vi "TLB Native Dynamic Events ver 0.26g.vi"() -> ()   [LabVIEW 2018]
uses:
  TLB Type Definitions/Intruction Type Definitions.ctl
  TLB Type Definitions/State Type Definitions, for 0.26g versions and later 3.ctl
  <vilib>/Studica/Studica Toolkit/NavX/TypeDefs/Flags/Z900_navX_Flags_OpStatusTypeDef.ctl
  <vilib>/Studica/Studica Toolkit/NavX/TypeDefs/Flags/Z900_navX_Flags_CalibrationStatusTypeDef.ctl
  TLB Type Definitions/Vision cluster.ctl
  TLB Type Definitions/PING CLUSTER.ctl
  TLB Type Definitions/Encoder cluster.ctl
  TLB Type Definitions/Stepper cluster.ctl
  TLB Type Definitions/Yaw Cluster.ctl
  TLB Type Definitions/IR Sensor Type Def.ctl
  TLB Type Definitions/Line Sensor Cluster.ctl
  TLB Type Definitions/Time cluster.ctl
  TLB Type Definitions/Box Colour Detection Cluster (0.26d and above).ctl
  Underlying VI's/FGV's/Box FGV/Box Colour FGV Colours.ctl
  <vilib>/Studica/Studica Toolkit/Background/DIO Channel.ctl
  TLB Type Definitions/Y Stepper cluster.ctl
  TLB Type Definitions/Motor Speed Cluster.ctl
  Labview Training Phase 2/Enum Controls/States for Action Engine.ctl
  Underlying VI's/NavX VI/navX type def.ctl
  <vilib>/Studica/Studica Toolkit/Background/I2C Channel.ctl
  Underlying VI's/I2C Master VI/Arduino_Interfacing.ctl
  Underlying VI's/Motor Control VI with PID/MOTOR CONTROL WITH PID AE DATA MODE TYPE DEF.ctl
  Underlying VI's/Motor Control VI with PID/MOTOR CONTROL WITH PID AE DIRECTION TYPE DEF.ctl
  Experimental VI's/Archived VI's/MOTOR CONTROL NO PID Type Def.ctl
  <vilib>/myRIO/Common/Instrument Driver Framework/myRIO v1.0/AI/typedefs/AI Channels List.ctl
  <vilib>/myRIO/Common/Instrument Driver Framework/myRIO v1.0/AI/typedefs/AI Channels Enum.ctl
  Underlying VI's/Line Sensor AE/Line Sensor AE Type Def.ctl
  Underlying VI's/I2C Master VI/I2C MASTER Type Def.ctl
  Underlying VI's/Elasped Timer/Elapsed timer control.ctl
  Underlying VI's/IMAQ Create Reference AE/IMAQ Reference AE.ctl
  Underlying VI's/FGV's/Box FGV/Box Colour FGV States.ctl
  Underlying VI's/I2C Master VI/I2C_MASTER_WRITE_NEW Type Def.ctl
  Underlying VI's/Modified webcam FGV/Webcam AE.ctl
  <vilib>/userdefined/High Color/IMAQdx.ctl
  <vilib>/Studica/Studica Toolkit/NavX/NavX.lvlib
  <vilib>/NI_Real-Time Target Support.lvlib
panel:
  out "Distance to move":dbl
  out "Same colour?":bool
  out "Box Colour Detection":T1
  out "Errors detected":bool
  out "Robot ready":bool
  out "Time cluster":T3
  out "Table IR obstruct":bool
  out "Front IR obstruct":bool
  out "CPU 1 Usage":dbl
  out "CPU 0 Usage":dbl
  out "Line sensors":T4
  out "IR Sensors":T5
  out "NAVX Values":T6
  out "Stepper position values":T7
  out "Encoder values":T8
  out "Ultrasonic sensors":T9
  out "Selected Task":T10=enum."Start Task 9"
  out "Object recognition mode":enum16{"Ball", "Soap", "Gel", "Pipe", "None"}(ring)
  out "Image Processing Error":errorcluster
  out "Object Detection":T11
  out "Status":T14 {"OP Status" items=["INITIALIZING", "SELFTEST_IN_PROGRESS", "ERROR", "IMU_AUTOCAL_IN_PROGRESS", "NORMAL"]; "Calibration Status" items=["IMU_CAL_STATE_MASK"=3, "IMU_CAL_STATE_INPROGRESS"=0, "IMU_CAL_STATE_ACCUMULATE"=1, "IMU_CAL_STATE_COMPLETE"=2]}
  out "General Errors":errorcluster
  in  "Red LED":bool
  out "Front Ultrasonic obstruct":bool
  out "Speed & distance":T15
  out "Task selection":u8
  out "NavX Readings":T16
  out "Arduino Data":T17
  out "TASK ENABLE":bool
  out "Rising Edge":bool
  in  "Green LED":bool
  out "State Logic":T18=enum."Startup"
  out "elements":T10[](array[typedef])
  in  "STOP TASK":bool
  in  "OK Button":bool
  in  "STOP":bool
  out "Queue Errors":errorcluster
  out "Action Queue Items":i32
  out "State Logic Queue Items":i32
  out "Action Queues items":string[](array[string])=["Hardware reset", "Software reset", ""]
  out "Action State":string
  # "VISION"
  # "TLB FRAMEWORK STATUS"
  # "System Health Status Update"
  # "Test Programme written by Calvin Loke    Dated: 28 Aug 2019\nTest Programme revised by Dr Alex See   Dated 30 Aug 2019\n\nRevision date: 20/03/2020\nProgramme version:   TLB Native Dynamic Events ver 0.19a"
  # "0: Task 1\n1: Task 2\n2: Task 3\n3: Task 4\n4: Task 5\n5: Task 6\n6: Task 7\n7: Task 8 Ball\n8: Task 8 Soap\n9: Task 8 Gel\n10: Task 8 Pipe\n11: Task 9 Blue\n12: Task 9 Black\n13: Task 9 Green\n14: Task 9 Red\n15: Task 9 Yellow"
  # "Ball: Right\nSoap: Left\nGel: Reverse\nPipe: Forward"
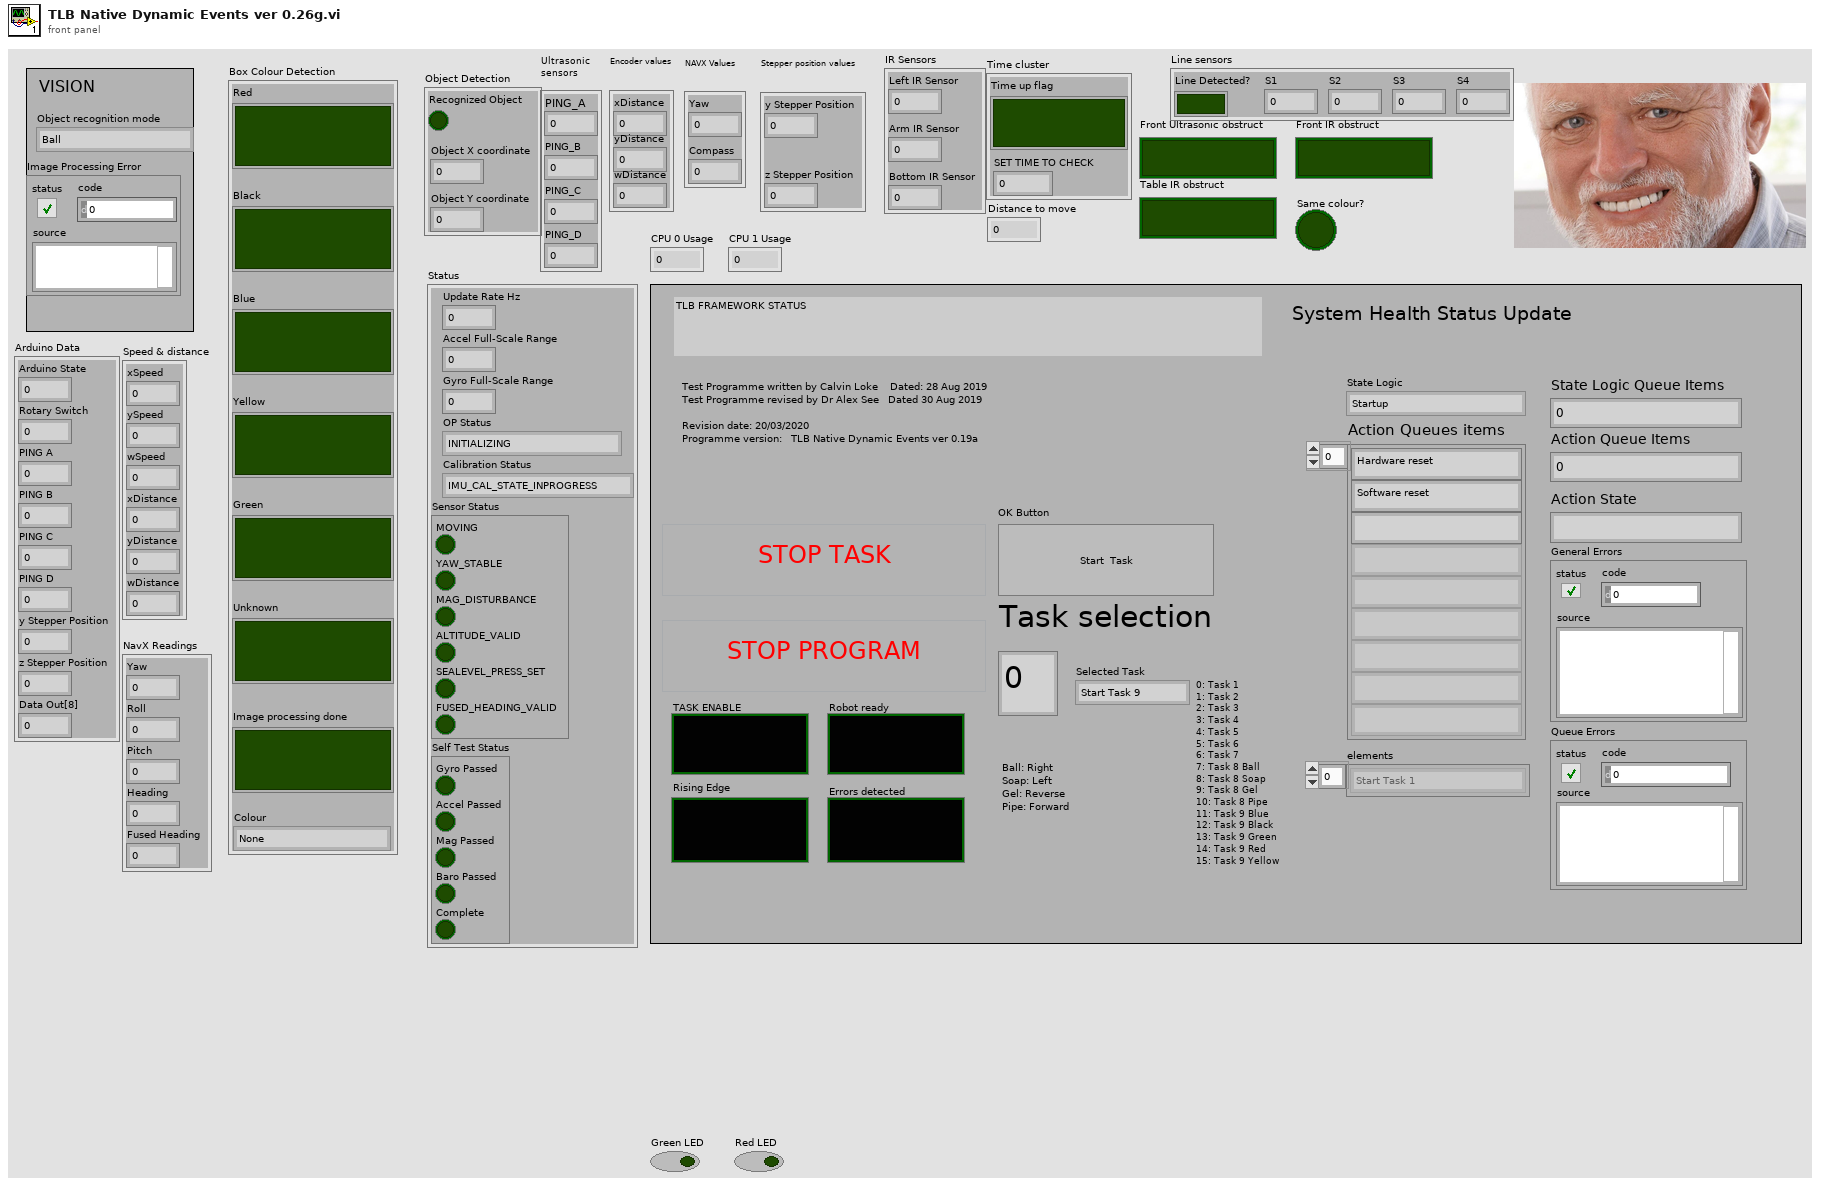
[diagram p1: front panel]
types:
  T1 = typedef "Box Colour Detection Cluster (0.26d and above).ctl" = cluster{"Red":bool, "Black":bool, "Blue":bool, "Yellow":bool, "Green":bool, "Unknown":bool, "Image processing done":bool, "Colour":T2}
  T2 = typedef "Box Colour FGV Colours.ctl" = enum16{"None", "Black", "Blue", "Green", "Red", "Yellow"}
  T3 = typedef "Time cluster.ctl" = cluster{"Time up flag":bool, "SET TIME TO CHECK":dbl}
  T4 = typedef "Line Sensor Cluster.ctl" = cluster{"Line Detected?":bool, "S1":dbl, "S2":dbl, "S3":dbl, "S4":dbl}
  T5 = typedef "IR Sensor Type Def.ctl" = cluster{"Left IR Sensor":dbl, "Arm IR Sensor":dbl, "Bottom IR Sensor":dbl}
  T6 = typedef "Yaw Cluster.ctl" = cluster{"Yaw":dbl, "Compass":dbl}
  T7 = typedef "Stepper cluster.ctl" = cluster{"y Stepper Position":u8, "z Stepper Position":u8}
  T8 = typedef "Encoder cluster.ctl" = cluster{"xDistance":dbl, "yDistance":dbl, "wDistance":dbl}
  T9 = typedef "PING CLUSTER.ctl" = cluster{"PING_A":u8, "PING_B":u8, "PING_C":u8, "PING_D":u8}
  T10 = typedef "Intruction Type Definitions.ctl" = enum16{"None", "Start Task 1", "Start Task 2", "Start Task 3", "Start Task 4", "Start Task 5", "Start Task 6", "Start Task 7", "Start Task 8 - BALL", "Start Task 8 - Gel", "Start Task 8 - Pipe", "Start Task 8 - Soap", "Start Task 9", "Start Task A", "Start Task B", "Exit"}
  T11 = typedef "Vision cluster.ctl" = cluster{"Recognized Object":bool, "Object X coordinate":dbl, "Object Y coordinate":dbl}
  T12 = typedef "NavX.lvlib/Z900_navX_Flags_OpStatusTypeDef.ctl" = u8
  T13 = typedef "NavX.lvlib/Z900_navX_Flags_CalibrationStatusTypeDef.ctl" = u8
  T14 = cluster{"Update Rate Hz":u8, "Accel Full-Scale Range":u8, "Gyro Full-Scale Range":u16, "OP Status":T12, "Calibration Status":T13, "Sensor Status":cluster{"MOVING":bool, "YAW_STABLE":bool, "MAG_DISTURBANCE":bool, "ALTITUDE_VALID":bool, "SEALEVEL_PRESS_SET":bool, "FUSED_HEADING_VALID":bool}, "Self Test Status":cluster{"Gyro Passed":bool, "Accel Passed":bool, "Mag Passed":bool, "Baro Passed":bool, "Complete":bool}}
  T15 = cluster{"xSpeed":dbl, "ySpeed":dbl, "wSpeed":dbl, "xDistance":dbl, "yDistance":dbl, "wDistance":dbl}
  T16 = cluster{"Yaw":dbl, "Roll":dbl, "Pitch":dbl, "Heading":dbl, "Fused Heading":dbl}
  T17 = cluster{"Arduino State":u8, "Rotary Switch":u8, "PING A":u8, "PING B":u8, "PING C":u8, "PING D":u8, "y Stepper Position":u8, "z Stepper Position":u8, "Data Out[8]":u8}
  T18 = typedef "State Type Definitions, for 0.26g versions and later 3.ctl" = enum16{"None", "Startup", "Move to Angle", "True Stop", "Idle", "Shutdown", "Task 1A", "Task 1B", "Task 2:Raise Arm", "Task 2:Sensor Mode", "Task 2:Reverse Mode", "Task 3", "Task 4_A", "Task 4_B", "Task 4_C", "Task 4_D", "Task 5A: RAISING ARM", "Task 5B: STILL WAITING", "Task 5C: GOING DOWN", "Task 5D: GRAB", "Task 5E: GOING UP", "Task 5F: ARM GRAB HEIGHT", "Task 5G: CLOSE CLAW", "Task 5H: RAISE ARM", "Task 6A: RAISE ARM", "Task 6B: CAM BURST", "Task 6C: PROCESS IMAGE", "Task 6D: BALL BUSTER", "Task 6E: STILL WAITING", "Task 6F: CAM BURST 2", "Task 6G: PROCESS IMAGE 2", "Task 6H: SKADI SOAPS", "Task 6I: STILL WAITING 2", "Task 6J: CAM BURST 3", "Task 6K: PROCESS IMAGE 3", "Task 6L: JAM IT IN", "Task 6M: STILL WAITING 3", "Task 6N: CAM BURST 4", "Task 6O: PROCESS IMAGE 4", "Task 6P: PIPE BOMB", "Task 7", "Task 8A: RAISE ARM", "Task 8B: MOVE TO BOX", "Task 8C: CAM BURST", "Task 8D: PROCESS IMAGE", "Task 8E: ROBOT ADJUST", "Task 8F: CAM BURST 2", "Task 8G: PROCESS IMAGE 2", "Task 8H: ARM ADJUST", "Task 8I: ARM GRAB HEIGHT", "Task 8J: CLOSE CLAW", "Task 8K: RAISE MY SWORD", "Task 9A: Raise Arm", "Task 9B: Rotate to Angle", "Task 9C: Detect Box", "Task 9D: MOVE FORWARD", "Task 9E: MOVE LEFT", "Task 9F: SCAN BOX", "Task 9G: MOVE RIGHT", "Task 9H: SCAN BOX 2", "Task 9I: ROTATE 90 CW", "Task 9J: FORWARD", "Task 9K: RAM WALL", "Task 9L: MOVE RIGHT", "Task 9M: SCAN BOX 3", "Task 9N: MOVE RIGHT", "Task 9O: SCAN BOX 4"}
  T19 = typedef "Motor Speed Cluster.ctl" = cluster{"ySpeed":dbl, "xSpeed":dbl, "wSpeed":dbl}
  T20 = typedef "Y Stepper cluster.ctl" = cluster{"yStepper desired":u8}
  T21 = typedef "DIO Channel.ctl" = enum16{"Not Connected", "A/DIO1", "A/DIO2", "A/DIO3", "A/DIO4", "A/DIO5", "A/DIO6", "A/DIO7", "A/DIO13", "B/DIO1", "B/DIO2", "B/DIO3", "B/DIO4", "B/DIO5", "B/DIO6", "B/DIO7", "B/DIO13", "C/DIO0", "C/DIO1", "C/DIO2", "C/DIO3", "C/DIO4", "C/DIO5", "C/DIO6", "C/DIO7"}
  T22 = cluster{"DIO Channel":T21, "FPGA VI Reference Out":refnum<k20>}
  T23 = typedef "States for Action Engine.ctl" = enum16{"Initialize", "Write", "Read"}
  T24 = typedef "NI_Real-Time Target Support.lvlib/RT CPU Load.ctl" = cluster{"Total (%)":dbl, "Time Critical (%)":dbl, "Timed Structures (%)":dbl, "High (%)":dbl, "Above Normal (%)":dbl, "Normal (%)":dbl, "Background (%)":dbl, "Idle (%)":dbl, "ISR (%)":dbl}
  T25 = cluster{"CPU loads[0]":T24, "CPU loads[1]":T24, "CPU loads[2]":T24, "CPU loads[3]":T24, "CPU loads[4]":T24, "CPU loads[5]":T24, "CPU loads[6]":T24, "CPU loads[7]":T24, "CPU loads[8]":T24}
  T26 = typedef "navX type def.ctl" = enum16{"Get i2C reference", "Read Values", "Zero Yaw"}
  T27 = typedef "Arduino_Interfacing.ctl" = enum16{"Initialize", "Write to Arduino", "Read From Arduino"}
  T28 = typedef "I2C Channel.ctl" = enum16{"Not Connected", "A", "B"}
  T29 = cluster{"I2C Ref Out":cluster{"I2C Channel":T28, "FPGA VI Reference Out":refnum<k20>}, "Connected":bool, "Slave Address (7-bit)":u8, "Registry":u8[]}
  T30 = typedef "Box Colour FGV States.ctl" = enum16{"Initialize", "Read", "Write"}
  T31 = typedef "MOTOR CONTROL WITH PID AE DIRECTION TYPE DEF.ctl" = enum16{"y-axis movement", "x-axis movement", "rotation", "stop", "reset encoders"}
  T32 = typedef "MOTOR CONTROL WITH PID AE DATA MODE TYPE DEF.ctl" = enum16{"Init AE", "Write to AE", "Read from AE"}
  T33 = typedef "Line Sensor AE Type Def.ctl" = enum16{"INIT AE", "READ FROM LINE SENSORS"}
  T34 = typedef "IMAQ Reference AE.ctl" = enum16{"Initialize AE", "Get IMAQ Reference", "Dispose Processing Buffer"}
  T35 = typedef "Elapsed timer control.ctl" = enum16{"Start", "Pause", "Initialize"}
  T36 = typedef "I2C_MASTER_WRITE_NEW Type Def.ctl" = enum16{"Ultrasonic sensors", "Stepper origin", "zStepper 13.3k", "zStepper 13k", "zStepper 12k", "zStepper 11k", "zStepper 10k", "zStepper 9k", "zStepper 8k", "zStepper 7k", "zStepper 6k", "zStepper 5k", "zStepper 4k", "zStepper 3k", "zStepper 2k", "zStepper 1k", "zStepper 900", "zStepper 800", "zStepper 700", "zStepper 600", "zStepper 500", "zStepper 400", "zStepper 300", "zStepper 200", "zStepper 100", "zStepper 0", "yStepper control", "Open Claw", "Close Claw", "Soft Reset"}
  T37 = typedef "Webcam AE.ctl" = enum16{"Initialize Camera", "Open Camera", "Continuous Acquisition", "Close Camera", "Retrieve Image", "Dispose Camera Image Buffer"}
  T38 = typedef "IMAQdx.ctl" = refnum<k21>
  T39 = typedef "MOTOR CONTROL NO PID Type Def.ctl" = enum16{"Init", "Front Back", "Left Right", "Rotate", "Stop", "Latch"}
  T40 = typedef "AI Channels List.ctl" = T41[]
  T41 = typedef "AI Channels Enum.ctl" = enum16{"Not Connected", "AudioIn/Left", "AudioIn/Right", "C/AI0", "C/AI1", "A/AI0", "A/AI1", "A/AI2", "A/AI3", "A/AI4", "A/AI5", "A/AI6", "A/AI7", "B/AI0", "B/AI1", "B/AI2", "B/AI3", "B/AI4", "B/AI5", "B/AI6", "B/AI7", "AI/AI0", "AI/AI1", "AI/AI2", "AI/AI3", "A/AI0 (DIFF)", "A/AI1 (DIFF)", "A/AI2 (DIFF)", "A/AI3 (DIFF)", "B/AI0 (DIFF)", "B/AI1 (DIFF)", "B/AI2 (DIFF)", "B/AI3 (DIFF)"}
  T42 = cluster{"S1":dbl, "S2":dbl, "S3":dbl, "S4":dbl, "Array[4]":dbl, "Array[5]":dbl, "Array[6]":dbl, "Array[7]":dbl, "Array[8]":dbl}
  T43 = typedef "I2C MASTER Type Def.ctl" = enum16{"Last State", "Mode 0", "Mode 1", "Mode 2", "Mode 3", "Mode 4", "Mode 5", "Mode 6", "Mode 7", "Mode 8", "Mode 9", "Mode 10"}
  T44 = typedef "IMAQ Image.ctl" = refnum<image>
  T45 = cluster{"Number of Matches":i32, "Object detected?":bool}
  T46 = cluster{"Red":bool, "Black":bool, "Blue":bool, "Yellow":bool, "Green":bool, "No recognizable coolour":bool}
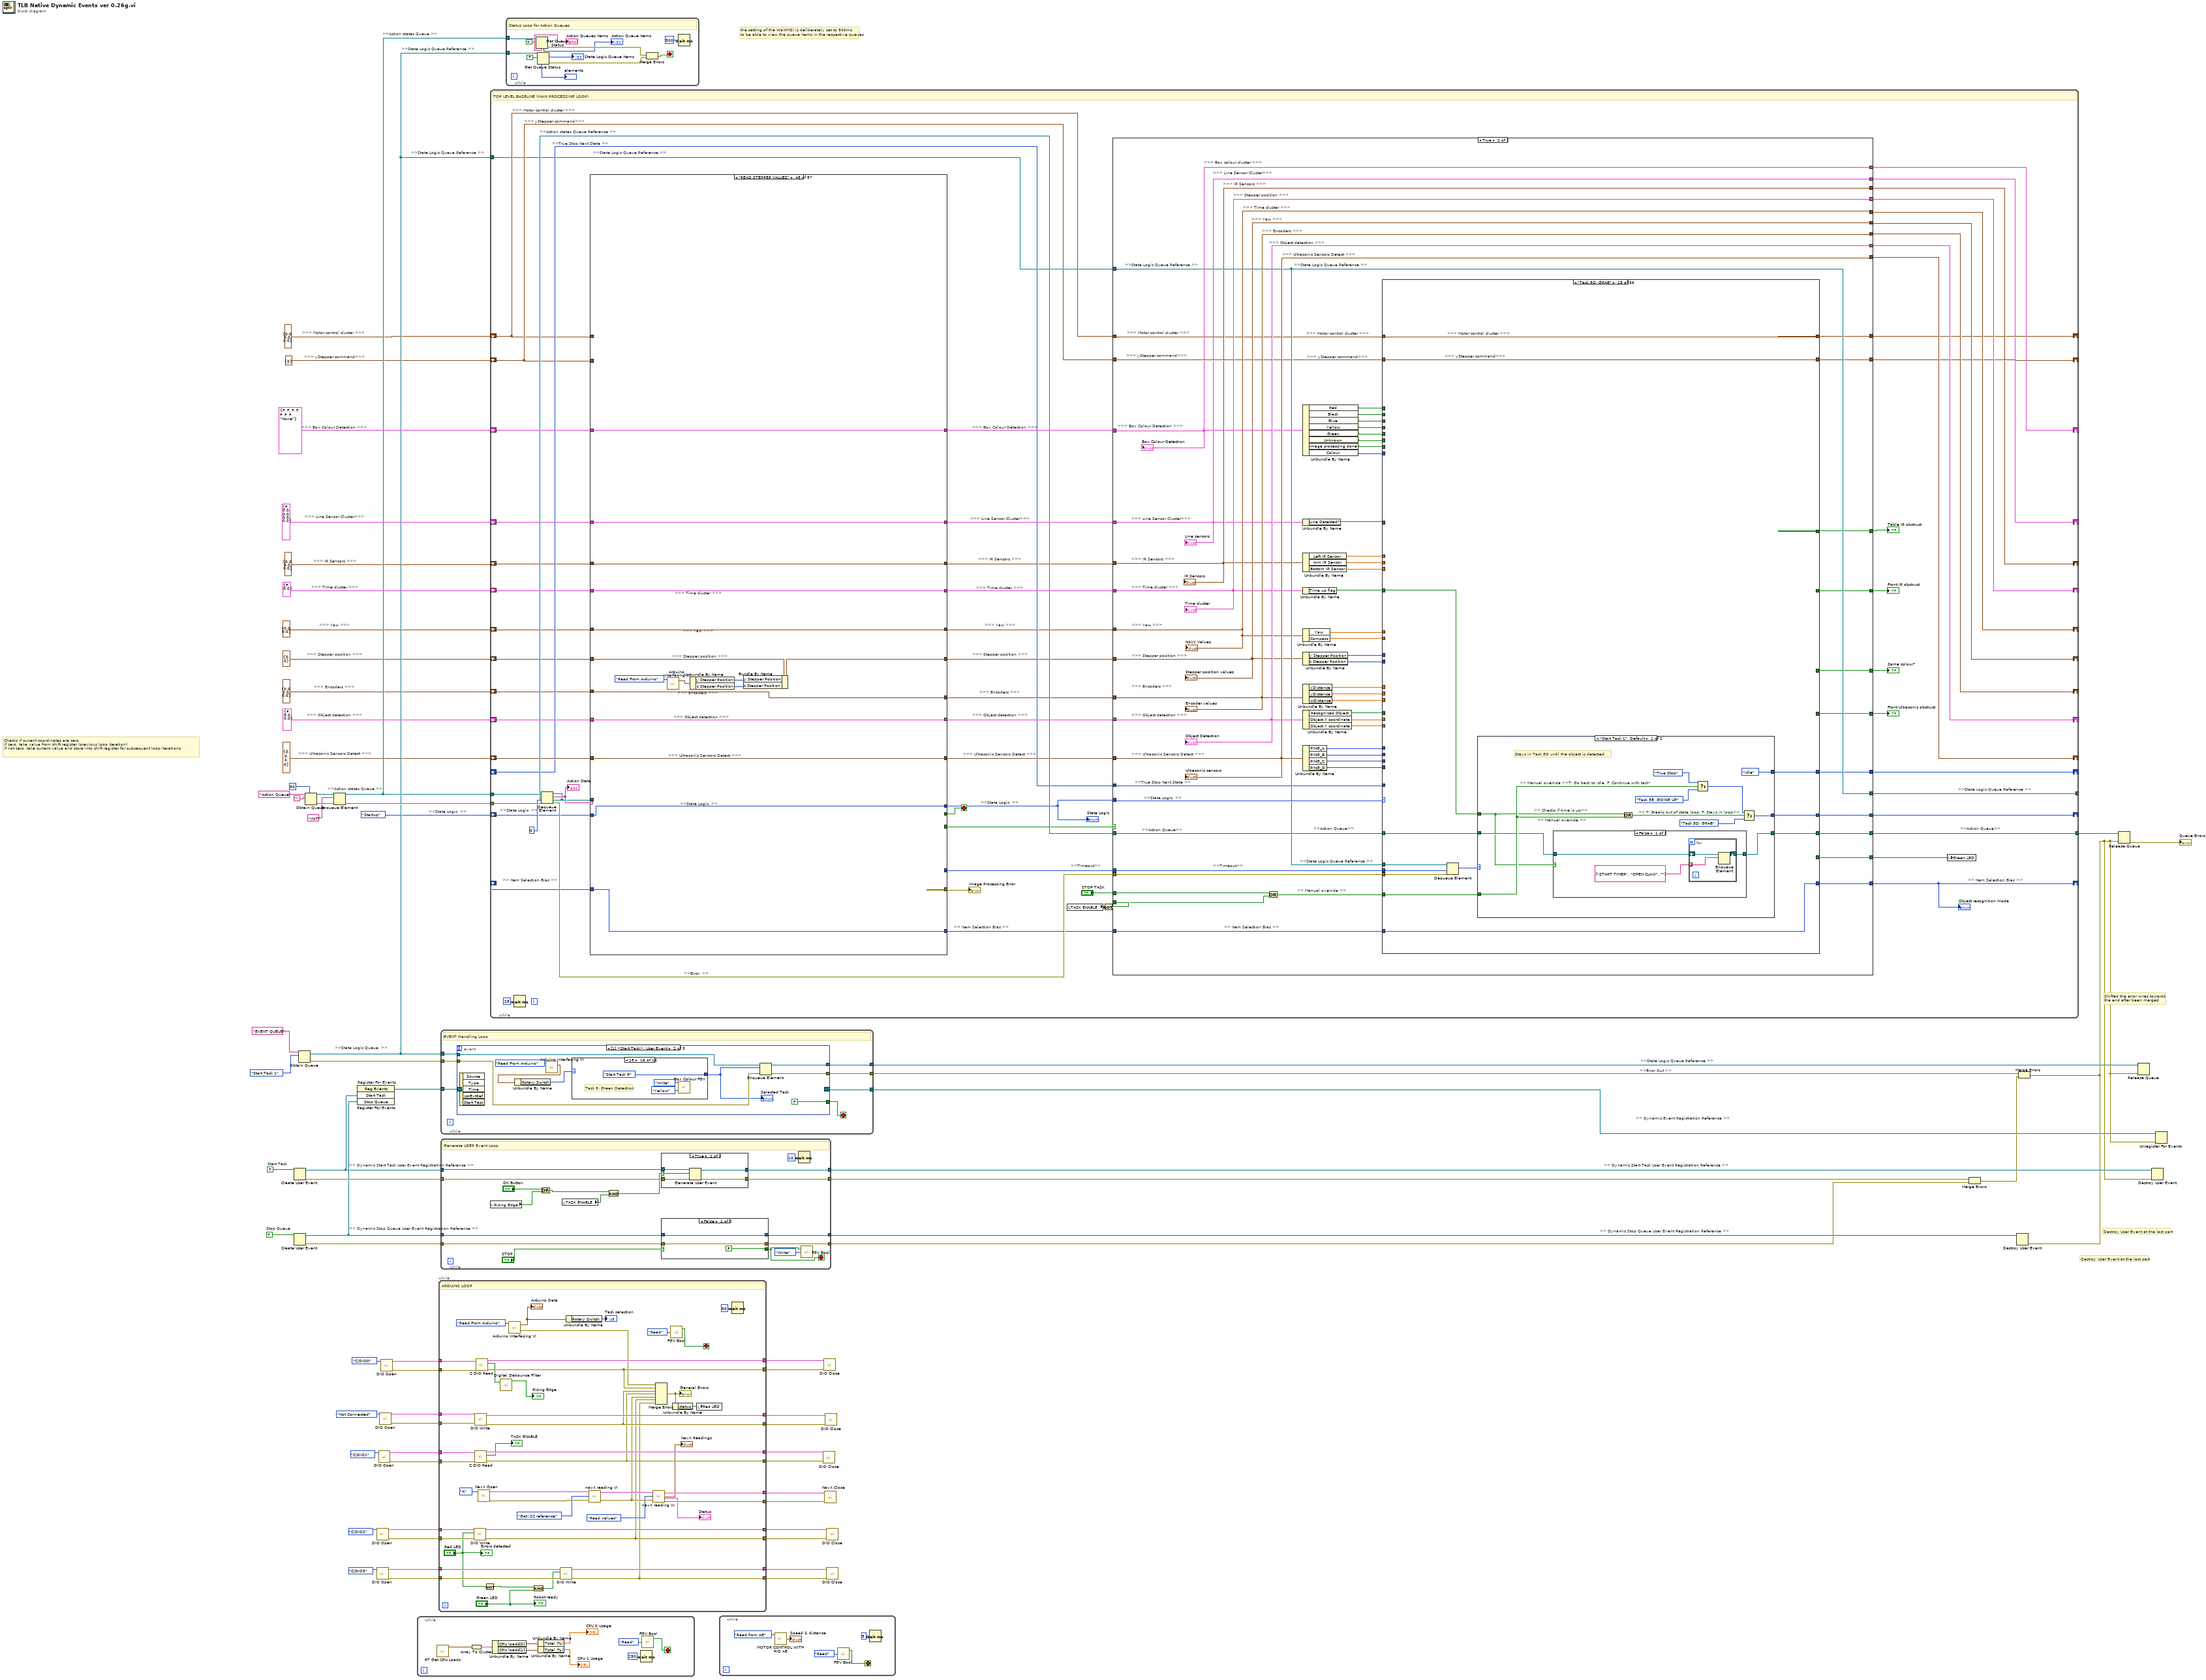
[diagram p0: block diagram]
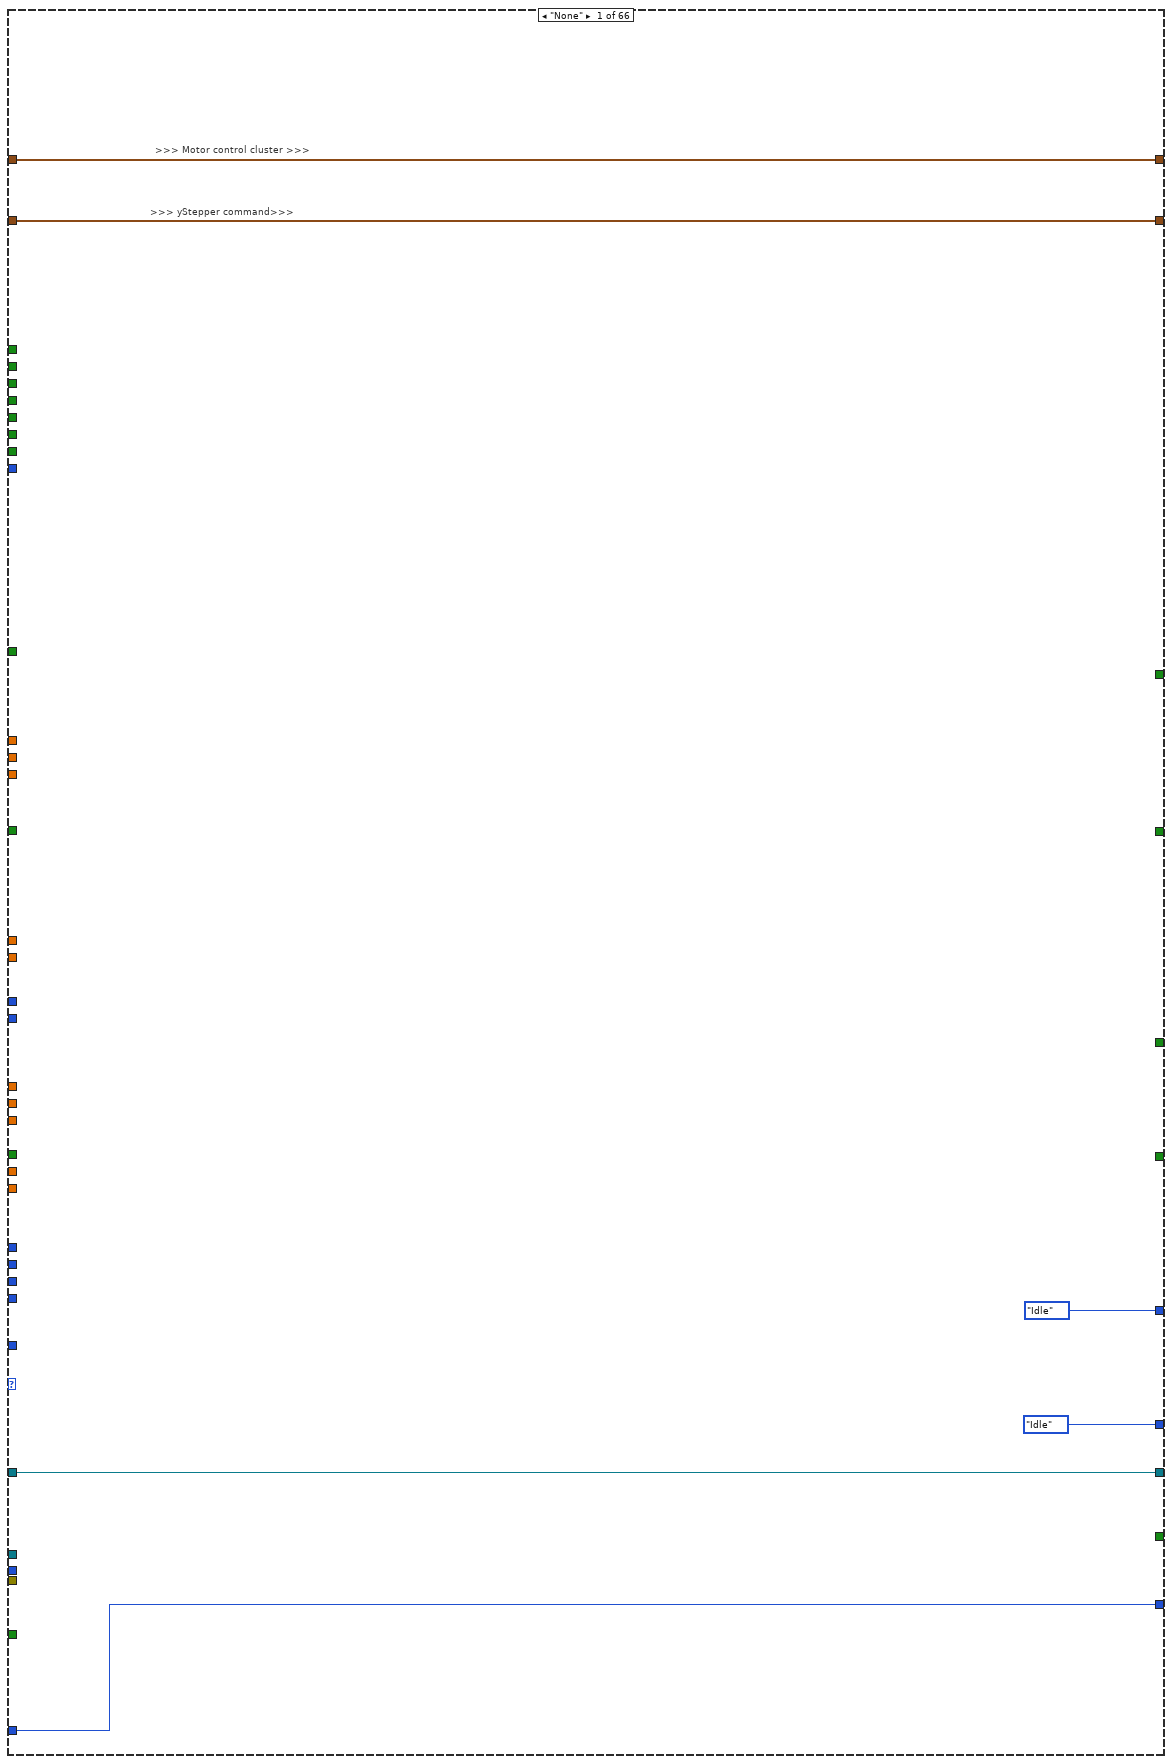
[diagram p3: hidden frame]
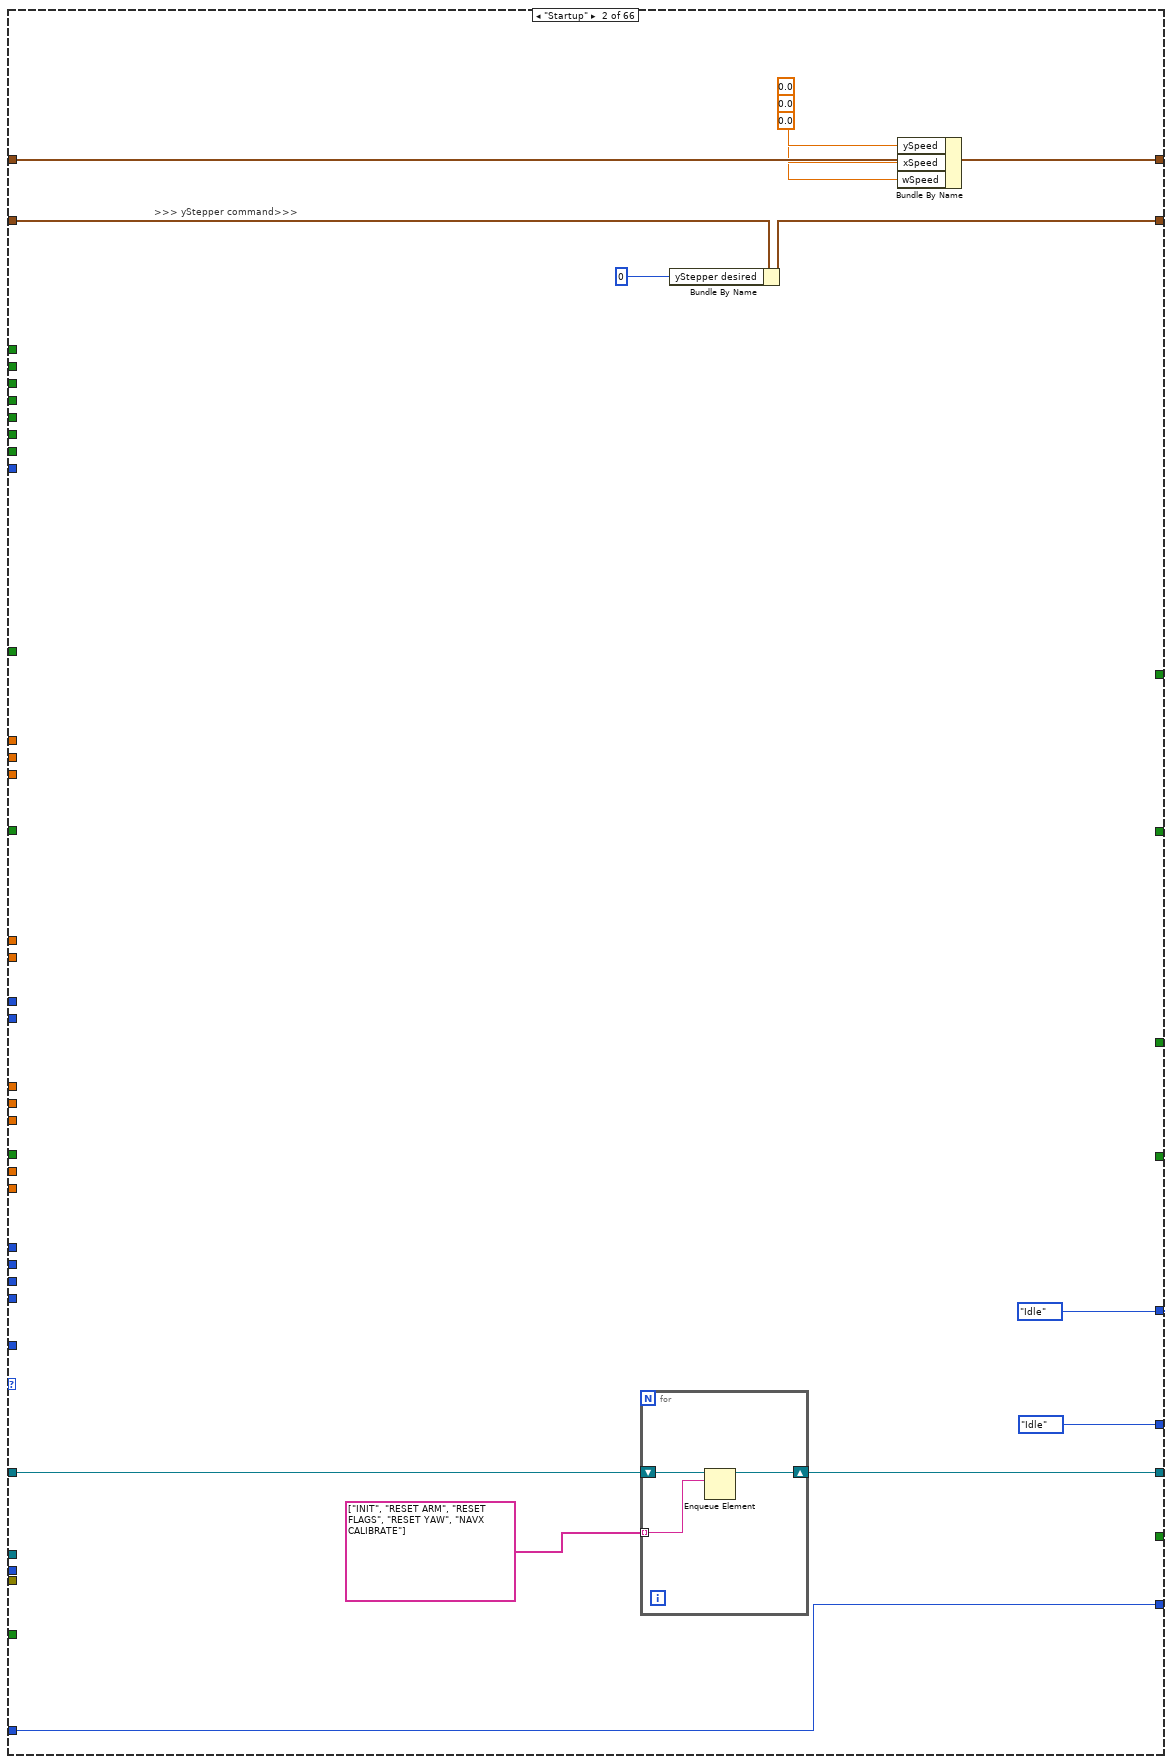
[diagram p4: hidden frame]
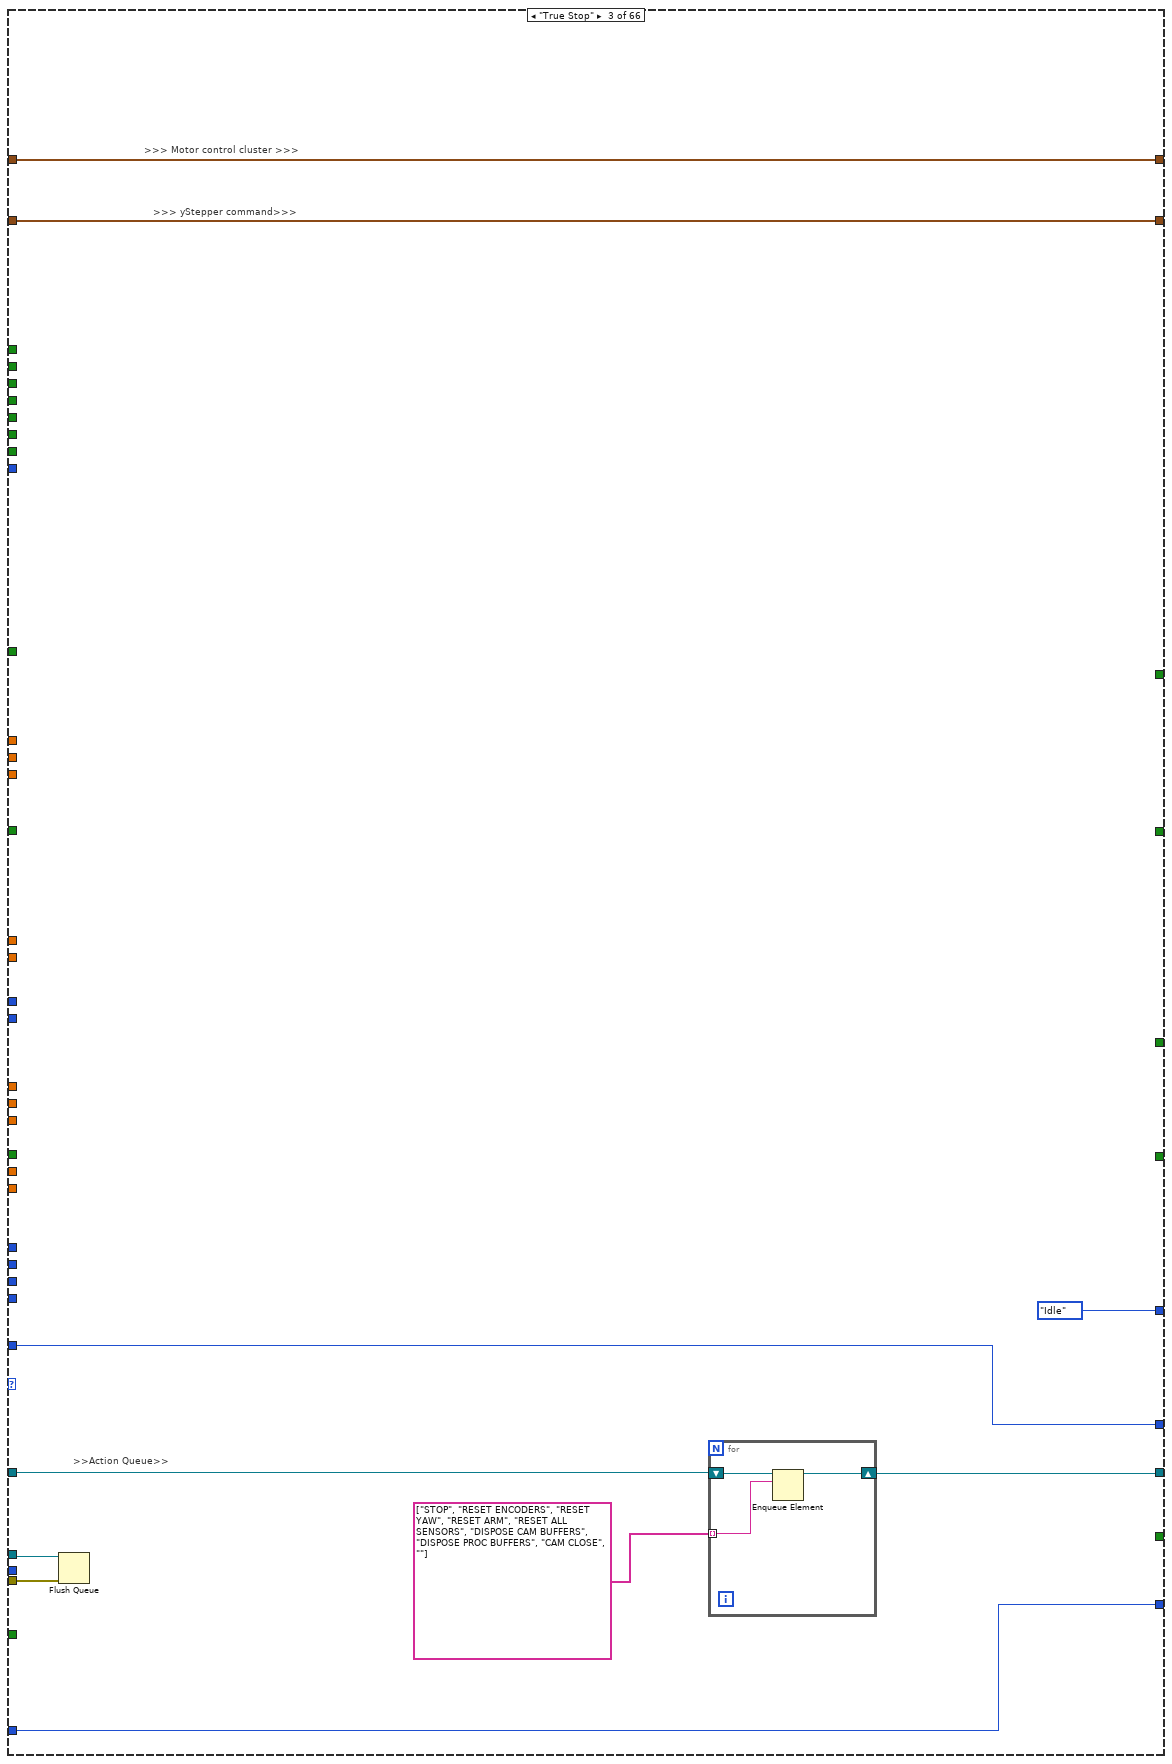
[diagram p5: hidden frame]
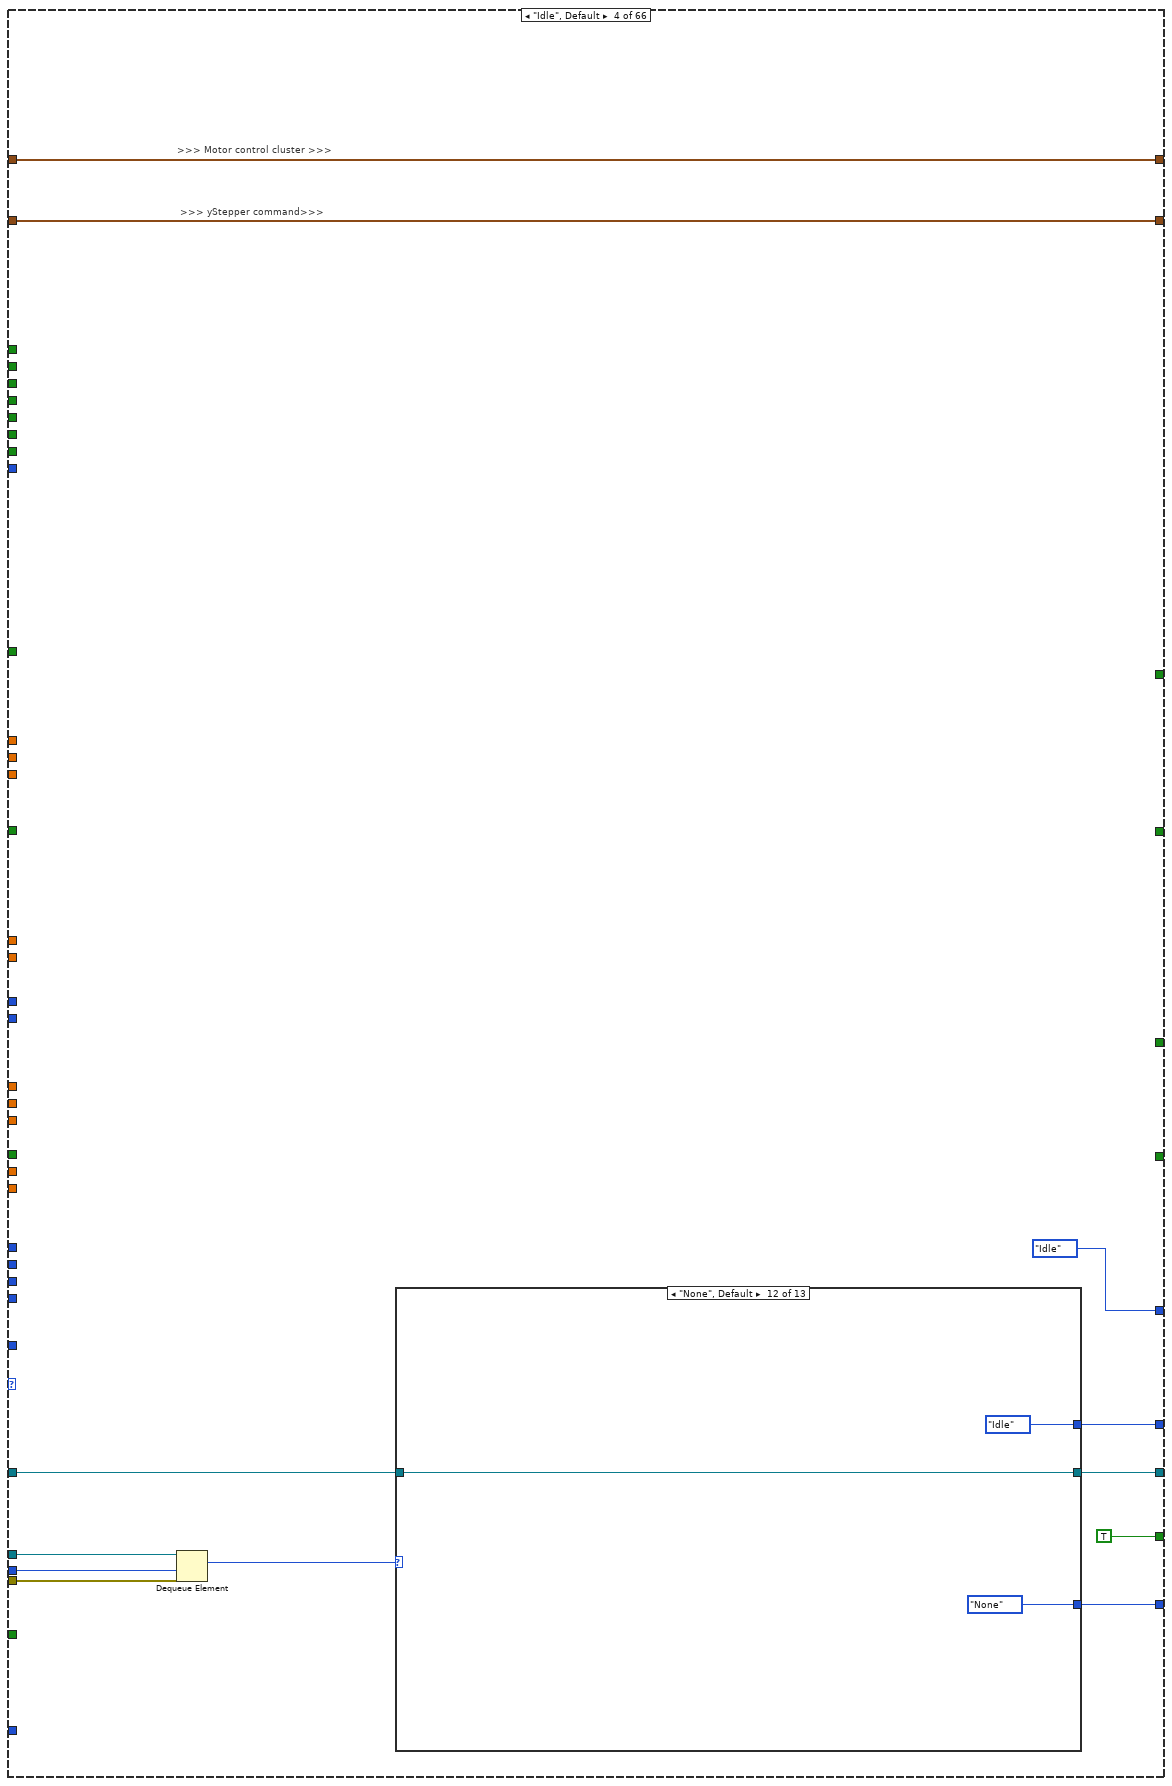
[diagram p6: hidden frame]
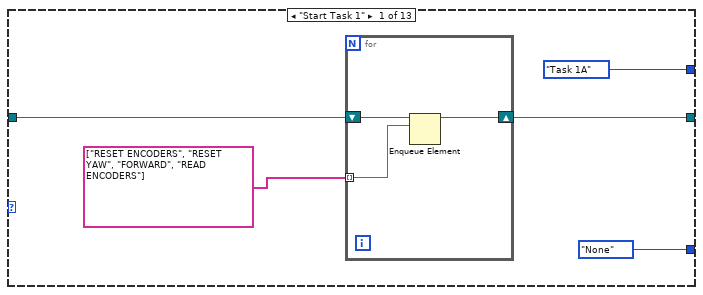
[diagram p7: hidden frame]
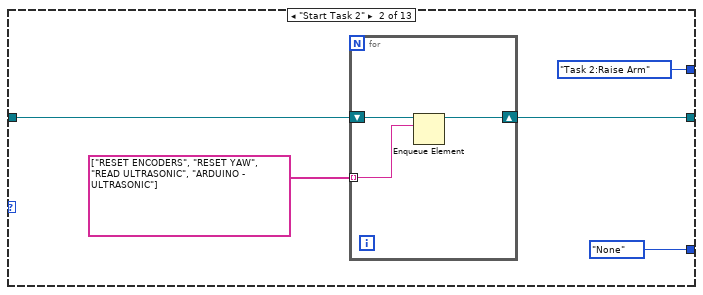
[diagram p8: hidden frame]
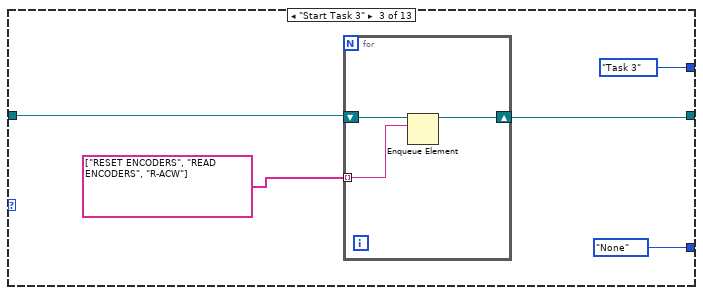
[diagram p9: hidden frame]
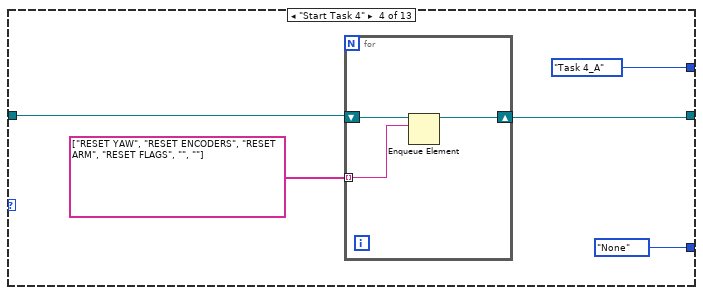
[diagram p10: hidden frame]
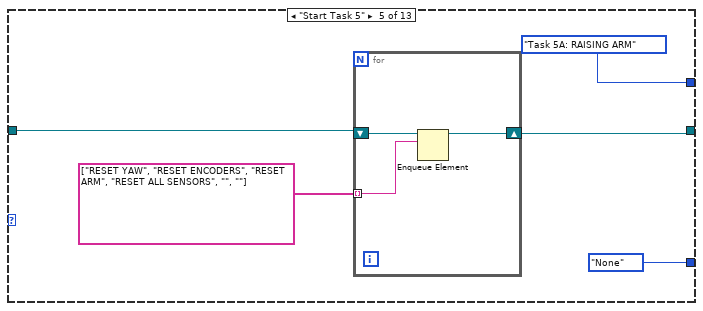
[diagram p11: hidden frame]
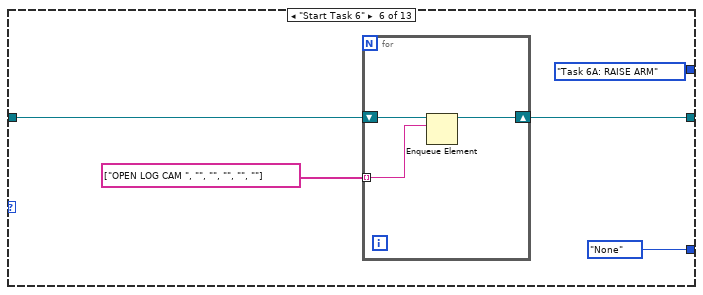
[diagram p12: hidden frame]
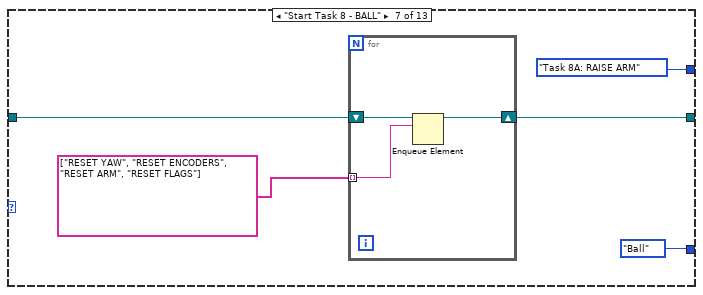
[diagram p13: hidden frame]
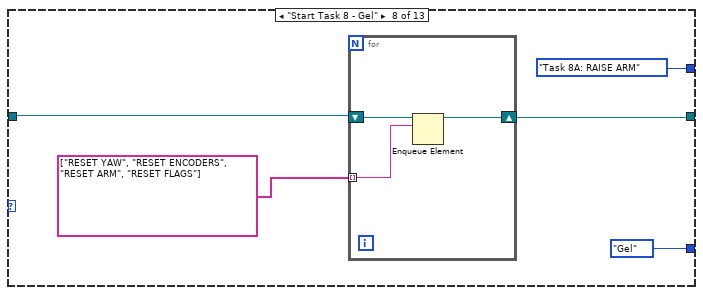
[diagram p14: hidden frame]
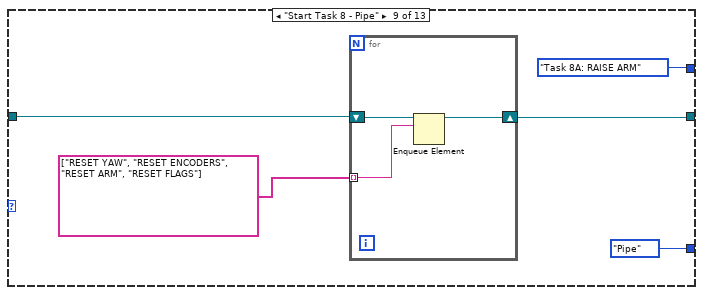
[diagram p15: hidden frame]
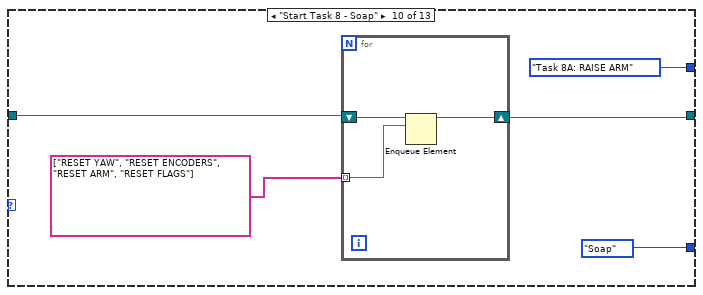
[diagram p16: hidden frame]
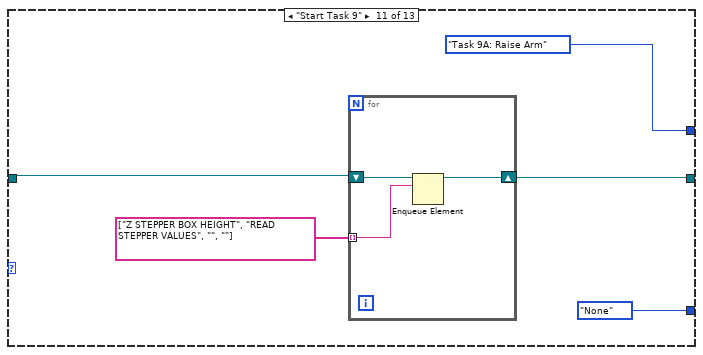
[diagram p17: hidden frame]
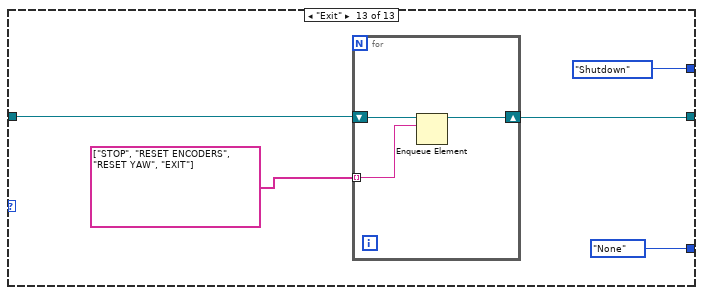
[diagram p18: hidden frame]
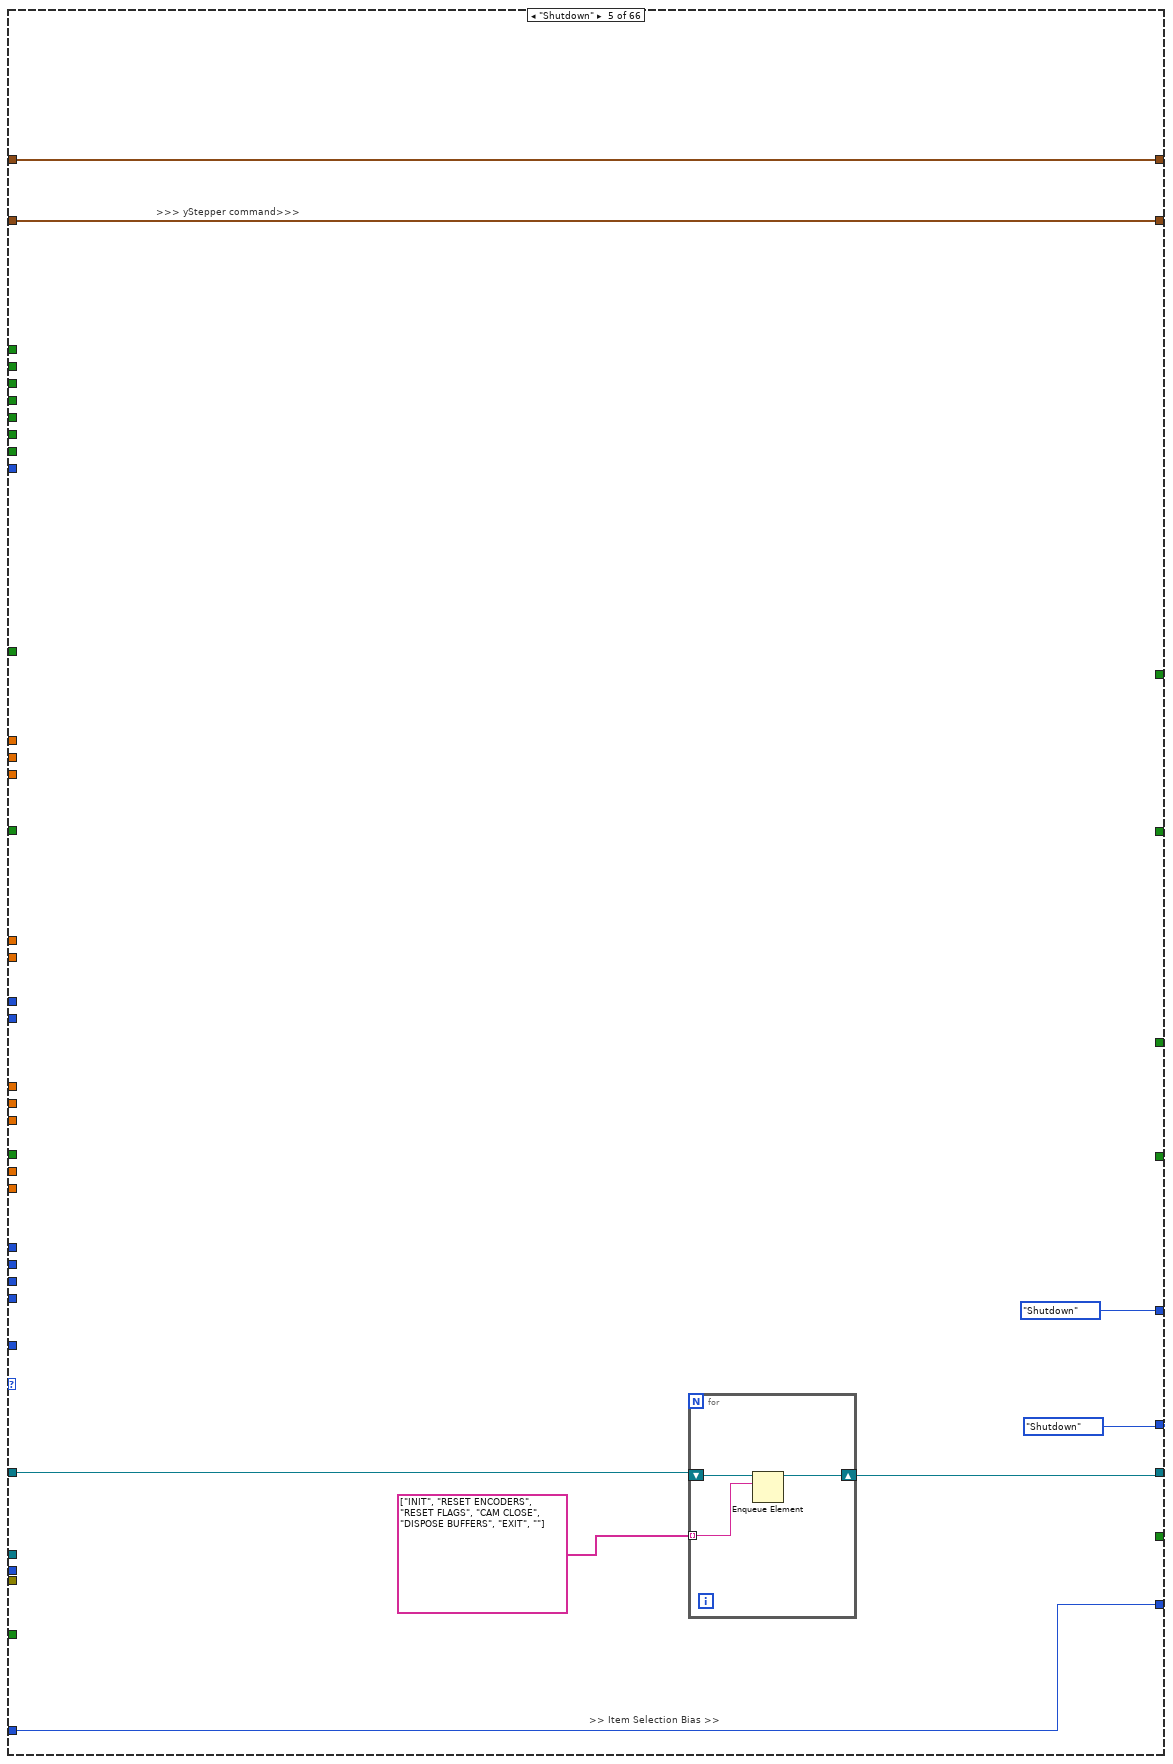
[diagram p19: hidden frame]
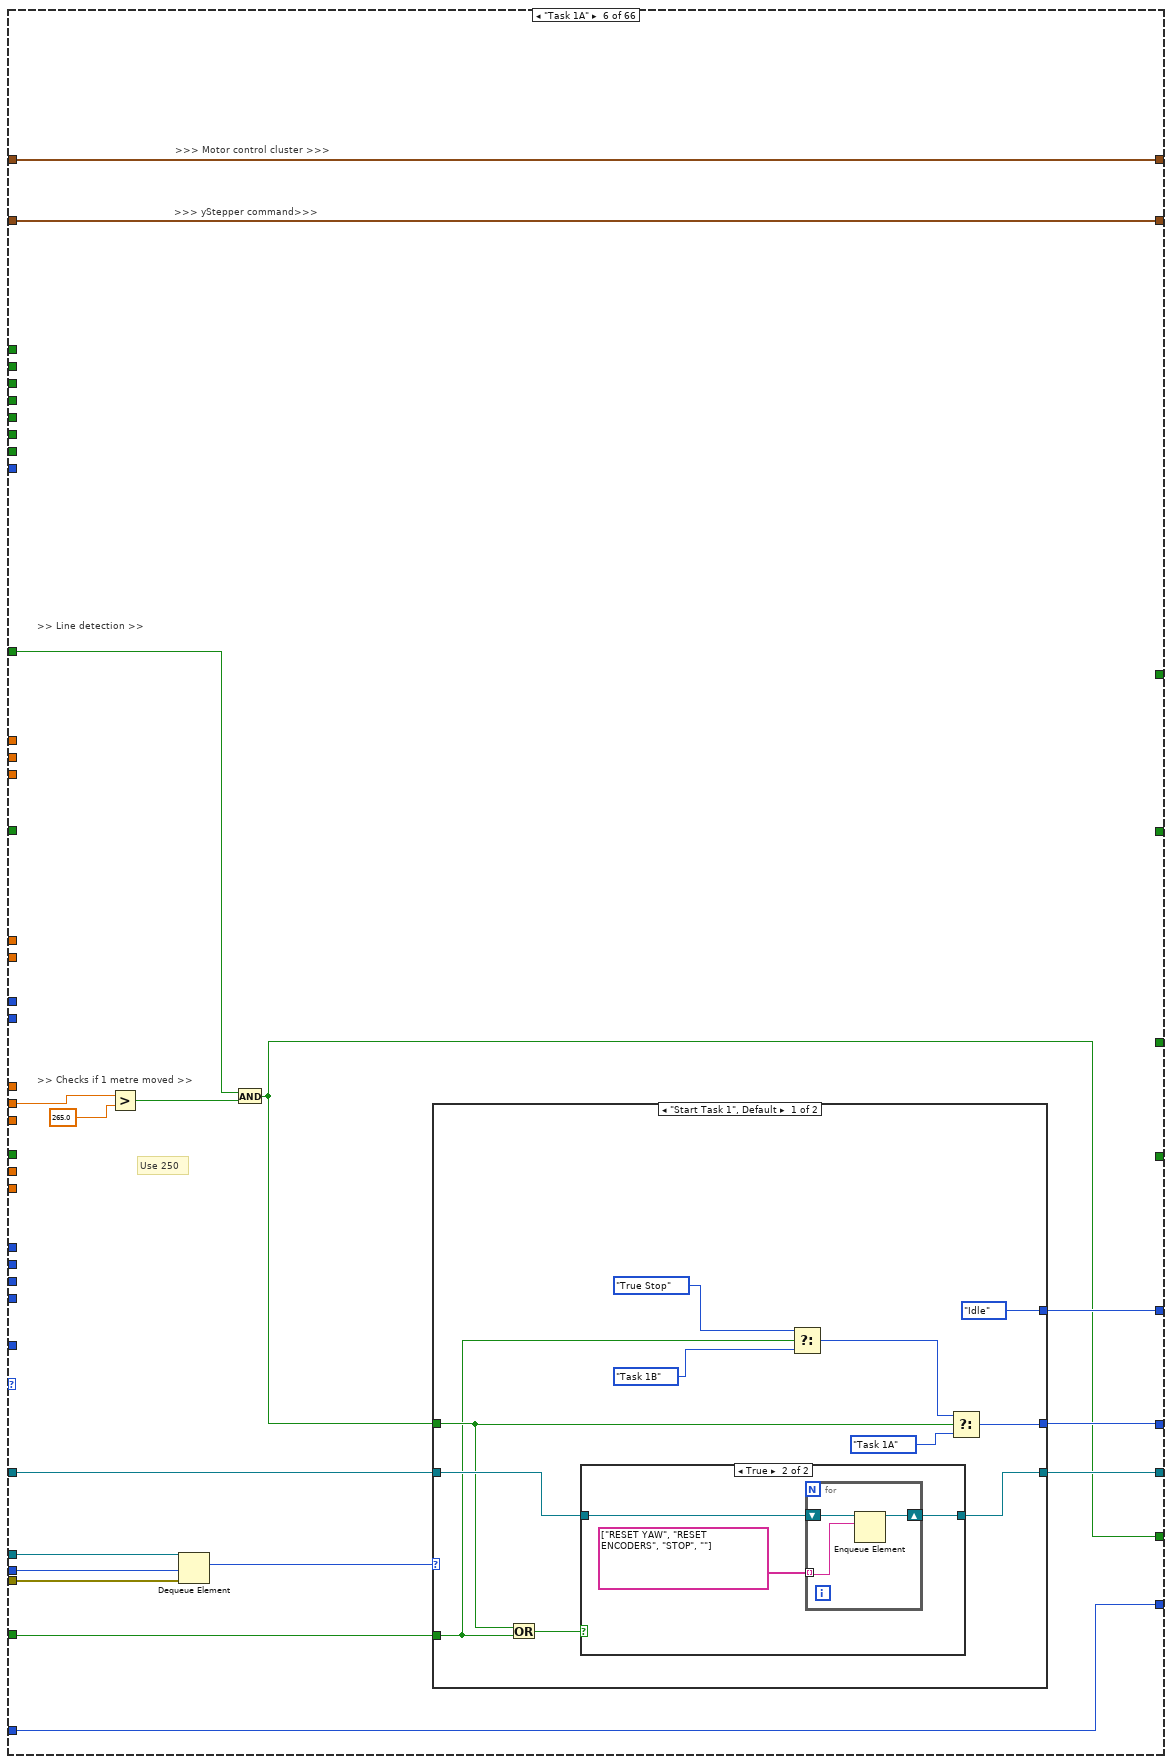
[diagram p20: hidden frame]
diagram:
  w69 = TRUE  # Stop Queue
  w68 = TRUE  # Start Task
  # ">>State Logic Queue Reference >>"
  # ">>Action states Queue >>"
  # ">>> Box Colour Detection >>>"
  # ">>State Logic Queue Reference >>"
  # ">>State Logic  >>"
  # ">>> Line Sensor Cluster>>>"
  # ">>> Motor control cluster >>>"
  # ">>> IR Sensors >>>"
  # "Checks if current coordinates are zero\nif zero, take value from shift register (previous loop iteration)\nif not zero, take current value and store into shift register for subsequent loop iterations"
  # ">>> yStepper command>>>"
  # ">>> Time cluster >>>"
  # ">>> Yaw >>>"
  # ">>> Stepper position >>>"
  # ">>> Encoders >>>"
  # ">>> Object detection >>>"
  # ">>> Ultrasonic Sensors Detect >>>"
  # "the setting of the Wait(MS) is deliberately set to 500ms\nto be able to view the queue items in the respective queues"
  # ">>Error Out >>"
  # ">> Dynamic Stop Queue User Event Registration Reference >>"
  # ">> Dynamic Start Task User Event Registration Reference >>"
  # ">> Dynamic Stop Queue User Event Registration Reference >>"
  # ">> Dynamic Start Task User Event Registration Reference >>"
  # ">> Dynamic Event Registration Reference >>"
  # ">>Action states Queue >>"
  # ">>State Logic Queue  >>"
  # ">>State Logic Queue Reference >>"
  # "Destroy User Event at the last part"
  # "Destroy User Event at the last part"
  # "Shifted the error wires towards\nthe end after been merged"
  n1 = Create User Event(user event datatype=w68) -> (user event=w60:refnum<user-event>, error out=w65:errorcluster)  [unwired: 1 in]
  n2 = Create User Event(user event datatype=w69) -> (user event=w61:refnum<user-event>, error out=w64:errorcluster)  [unwired: 1 in]
  n3 = Obtain Queue(name (unnamed)="EVENT QUEUE", element data type=Intruction_Type_Definitions."Start Task 1" ("Enum")) -> (queue out=w46:refnum<queue>, error out=w52:errorcluster)  [unwired: 3 in, 1 out]
  n4 = Obtain Queue(max queue size (-1, unlimited)=50, name (unnamed)="Action Queue", element data type="") -> (queue out=w55:refnum<queue>, error out=w51:errorcluster)  [unwired: 2 in, 1 out]
  n5 = Enqueue Element(queue=w55, element="INIT", error in (no error)=w51) -> (queue out=w47:refnum<queue>, error out=w50:errorcluster)  [unwired: 1 in, 1 out]
  n6 = register-events "Register For Events"(w60, w61) -> (reference out=w59:refnum<event-registration>)  [unwired: 2 in, 1 out]
  n7 = call <vilib>:"DIO Open.vi"("DIO Channel"=DIO_Channel."C/DIO2") -> ("error out"=w19:errorcluster, "DIO Info Out"=w20:T22)  [unwired: 9 in]
  n8 = call <vilib>:"DIO Open.vi"("DIO Channel"=DIO_Channel."C/DIO3") -> ("error out"=w14:errorcluster, "DIO Info Out"=w15:T22)  [unwired: 9 in]
  n9 = call <vilib>:"DIO Open.vi"("DIO Channel"=DIO_Channel."C/DIO1") -> ("error out"=w24:errorcluster, "DIO Info Out"=w25:T22)  [unwired: 9 in]
  n10 = call <vilib>:"DIO Open.vi"("DIO Channel"=DIO_Channel."Not Connected") -> ("error out"=w29:errorcluster, "DIO Info Out"=w31:T22)  [unwired: 9 in]
  n11 = call <vilib>:"DIO Open.vi"("DIO Channel"=DIO_Channel."C/DIO0") -> ("error out"=w34:errorcluster, "DIO Info Out"=w37:T22)  [unwired: 9 in]
  n12 = while {
    stop <- w76 stop-if-true
    n13 = call <vilib>:"RT Get CPU Loads.vi"() -> ("CPU loads"=w75:T24[])  [unwired: 10 in, 1 out]
    n14 = Array To Cluster(array=w75) -> (cluster=w74:T25)
    n15 = Unbundle By Name(w74) -> ("CPU loads[0]"=w73:T24, "CPU loads[1]"=w72:T24)
    n16 = Unbundle By Name(w73) -> ("Total (%)"=→"CPU 0 Usage":dbl)
    n17 = Unbundle By Name(w72) -> ("Total (%)"=→"CPU 1 Usage":dbl)
    n18 = Wait (ms)(milliseconds to wait=u32 250) -> ()  [unwired: 1 out]
    n19 = call "FGV Bool.vi"("Init/Read/Write State"=States_for_Action_Engine."Read") -> ("Output node"=w76:bool)  [unwired: 2 in, 1 out]
  }
  n20 = while {
    tunnel: w37 -> [w122]
    tunnel: [w121] -> w35
    tunnel: w34 -> [w120]
    tunnel: [w91] -> w33
    tunnel: w31 -> [w117]
    tunnel: [w116] -> w30
    tunnel: w29 -> [w115]
    tunnel: [w90] -> w28
    tunnel: [w114] -> w26
    tunnel: w25 -> [w113]
    tunnel: w24 -> [w112]
    tunnel: [w89] -> w23
    tunnel: w20 -> [w106]
    tunnel: w19 -> [w105]
    tunnel: [w104] -> w18
    tunnel: [w87] -> w17
    tunnel: w15 -> [w103]
    tunnel: w14 -> [w102]
    tunnel: [w101] -> w13
    tunnel: [w86] -> w12
    tunnel: [w98] -> w9
    tunnel: [w97] -> w10
    stop <- w124 stop-if-true
    # "ARDUINO LOOP"
    n21 = call <vilib>:"DIO Write.vi"("error in (no error)"=w105, "Input"="Red LED", "DIO Info In"=w106) -> ("error out"=w87:errorcluster, "DIO Info Out"=w104:T22)  [unwired: 7 in]
    n22 = call <vilib>:"DIO Write.vi"("error in (no error)"=w115, "DIO Info In"=w117) -> ("error out"=w90:errorcluster, "DIO Info Out"=w116:T22)  [unwired: 8 in]
    n23 = call <vilib>:"C DIO Read.vi"("error in (no error)"=w112, "DIO Info In in"=w113) -> ("error out"=w89:errorcluster, "IN"=→"TASK ENABLE":bool, "DIO Info In out"=w114:T22)  [unwired: 7 in]
    n24 = call <vilib>:"C DIO Read.vi"("error in (no error)"=w120, "DIO Info In in"=w122) -> ("error out"=w91:errorcluster, "IN"=w119:bool, "DIO Info In out"=w121:T22)  [unwired: 7 in]
    n25 = call <vilib>:"NavX Open.vi"("I2C Channel"=I2C_Channel."A") -> ("error out"=w108:errorcluster, "NavX Info"=w110:T29)  [unwired: 9 in]
    n26 = Not(x="Red LED") -> (.not. x?=w81:bool)
    n27 = call "Digital Debounce Filter.vi"("Boolean input"=w119) -> ("Rising Edge"=→"Rising Edge":bool)  [unwired: 1 in, 2 out]
    n28 = call "Arduino Interfacing VI.vi"("AE Mode"=Arduino_Interfacing."Read From Arduino") -> ("error out"=w92:errorcluster, "Arduino Data"=w94:T17)  [unwired: 3 in]
    "Arduino Data" <- w94
    n29 = And(x=w81, y="Green LED") -> (x .and. y?=w83:bool)
    n30 = call <vilib>:"DIO Write.vi"("error in (no error)"=w102, "Input"=w83, "DIO Info In"=w103) -> ("error out"=w86:errorcluster, "DIO Info Out"=w101:T22)  [unwired: 7 in]
    n31 = Unbundle By Name(w94) -> ("Rotary Switch"=→"Task selection":u8)
    n32 = call "navX reading VI.vi"("NavX Info In"=w110, "Mode"=navX_type_def."Get i2C reference", "error in (no error)"=w108) -> ("NavX Info Out"=w99:T29, "Error Out"=w88:errorcluster)  [unwired: 2 out]
    n33 = call "navX reading VI.vi"("NavX Info In"=w99, "Mode"=navX_type_def."Read Values", "error in (no error)"=w88) -> ("NavX Info Out"=w98:T29, "NavX Readings"=→"NavX Readings":T16, "Status"=→"Status":T14, "Error Out"=w97:errorcluster)
    n34 = Merge Errors(w92, w91, w90, w89, w88, w87, w86) -> (w84:errorcluster)
    "General Errors" <- w84
    n35 = call "FGV Bool.vi"("Init/Read/Write State"=States_for_Action_Engine."Read") -> ("Output node"=w124:bool)  [unwired: 2 in, 1 out]
    n36 = Unbundle By Name(w84) -> ("status"=w82:bool)
    n37 = local write "Red LED"(w82) -> ()
    n38 = Wait (ms)(milliseconds to wait=u32 50) -> ()  [unwired: 1 out]
    "Robot ready" <- "Green LED"
    "Errors detected" <- "Red LED"
  }
  n39 = while {
    tunnel: w60 -> [w142]
    tunnel: w61 -> [w141]
    tunnel: [w140] -> w67
    tunnel: [w139] -> w66
    tunnel: w65 -> [w138]
    tunnel: [w137] -> w63
    tunnel: w64 -> [w136]
    tunnel: [w135] -> w62
    stop <- w133 stop-if-true
    # "Generate USER Event Loop"
    n40 = local read "Rising Edge"() -> (w130:bool)
    n41 = Or(x="OK Button", y=w130) -> (x .or. y?=w129:bool)
    n42 = local read "TASK ENABLE"() -> (w128:bool)
    n43 = And(x=w129, y=w128) -> (x .and. y?=w127:bool)
    n44 = case shown="True" w127 {
      selector: w127 -> [_ w153]
      tunnel: w142 -> [w152 w157]
      tunnel: [w152 w156] -> w139
      tunnel: w138 -> [w151 w155]
      tunnel: [w151 w154] -> w137
      frame False {
      }
      frame True {
        n45 = Generate User Event(user event=w157, event data cluster=w153, error in=w155) -> (user event out=w156:refnum<user-event>, error out=w154:errorcluster)  [unwired: 1 in]
      }
    }
    n46 = case shown="False" "STOP" {
      selector: "STOP" -> [_ w146]
      tunnel: w141 -> [w145 w150]
      tunnel: [w145 w149] -> w140
      tunnel: w136 -> [w144 w148]
      tunnel: [w144 w147] -> w135
      tunnel: [FALSE w146] -> w133
      frame False {
      }
      frame True {
        n47 = Generate User Event(user event=w150, event data cluster=w146, error in=w148) -> (user event out=w149:refnum<user-event>, error out=w147:errorcluster)  [unwired: 1 in]
      }
    }
    n48 = Wait (ms)(milliseconds to wait=u32 10) -> ()  [unwired: 1 out]
    n49 = call "FGV Bool.vi"("Init/Read/Write State"=States_for_Action_Engine."Write", "Input Node"=w133) -> ()  [unwired: 1 in, 2 out]
  }
  n50 = while {
    tunnel: w59 -> [w164]
    tunnel: [w163] -> w58
    tunnel: w46 -> [w161]
    tunnel: [w160] -> w57
    tunnel: w52 -> [w159]
    tunnel: [w158] -> w49
    stop <- w162 stop-if-true
    # "EVENT Handling Loop"
    n51 = event shown="[1] <Start Task>: User Event" {
      selector: w164 -> [_ _ _]
      dyn-events: [_ _ _] -> w163
      timeout: _ -> [_ _ _]
      tunnel: [FALSE FALSE w211] -> w162
      tunnel: w161 -> [w169 w178 w209]
      tunnel: [w168 w177 w210] -> w160
      tunnel: w159 -> [w167 w176 w208]
      tunnel: [w166 w175 w207] -> w158
      event Timeout {
        n52 = event-data() -> ()  [unwired: 1 in, 3 out]
        n53 = Enqueue Element(queue=w169, element=Intruction_Type_Definitions."Start Task 1" ("Enum"), error in (no error)=w167) -> (queue out=w168:refnum<queue>, error out=w166:errorcluster)  [unwired: 1 in, 1 out]
      }
      event User Event {
        n54 = event-data() -> ()  [unwired: 1 in, 5 out]
        n55 = call "Arduino Interfacing VI.vi"("AE Mode"=Arduino_Interfacing."Read From Arduino") -> ("Arduino Data"=w172:T17)  [unwired: 3 in, 1 out]
        n56 = Unbundle By Name(w172) -> ("Rotary Switch"=w171:u8)
        n57 = case shown="15" w171 {
          tunnel: [Intruction_Type_Definitions."Start Task 1" ("Enum") Intruction_Type_Definitions."Start Task 2" ("Enum") Intruction_Type_Definitions."Start Task 3" ("Enum") Intruction_Type_Definitions."Start Task 4" ("Enum") Intruction_Type_Definitions."Start Task 5" ("Enum") Intruction_Type_Definitions."Start Task 6" ("Enum") Intruction_Type_Definitions."Start Task 7" ("Enum") Intruction_Type_Definitions."Start Task 8 - BALL" ("Enum") Intruction_Type_Definitions."Start Task 8 - Soap" ("Enum") Intruction_Type_Definitions."Start Task 8 - Gel" ("Enum") Intruction_Type_Definitions."Start Task 8 - Pipe" ("Enum") Intruction_Type_Definitions."Start Task 9" ("Enum") Intruction_Type_Definitions."Start Task 9" ("Enum") Intruction_Type_Definitions."Start Task 9" ("Enum") Intruction_Type_Definitions."Start Task 9" ("Enum") Intruction_Type_Definitions."Start Task 9" ("Enum")] -> w174
          frame 0, Default {
          }
          frame 1 {
          }
          frame 2 {
          }
          frame 3 {
          }
          frame 4 {
          }
          frame 5 {
          }
          frame 6 {
          }
          frame 7 {
          }
          frame 8 {
          }
          frame 9 {
          }
          frame 10 {
          }
          frame 11 {
            # "Task 9: Red Detection"
            n58 = call "Box Colour FGV.vi"("Colour to detect"=Box_Colour_FGV_Colours."Blue", "Init/R/W State"=Box_Colour_FGV_States."Write") -> ()  [unwired: 8 in, 2 out]
          }
          frame 12 {
            # "Task 9: Black Detection"
            n59 = call "Box Colour FGV.vi"("Colour to detect"=Box_Colour_FGV_Colours."Black", "Init/R/W State"=Box_Colour_FGV_States."Write") -> ()  [unwired: 8 in, 2 out]
          }
          frame 13 {
            # "Task 9: Blue Detection"
            n60 = call "Box Colour FGV.vi"("Colour to detect"=Box_Colour_FGV_Colours."Green", "Init/R/W State"=Box_Colour_FGV_States."Write") -> ()  [unwired: 8 in, 2 out]
          }
          frame 14 {
            # "Task 9: Yellow Detection"
            n61 = call "Box Colour FGV.vi"("Colour to detect"=Box_Colour_FGV_Colours."Red", "Init/R/W State"=Box_Colour_FGV_States."Write") -> ()  [unwired: 8 in, 2 out]
          }
          frame 15 {
            # "Task 9: Green Detection"
            n62 = call "Box Colour FGV.vi"("Colour to detect"=Box_Colour_FGV_Colours."Yellow", "Init/R/W State"=Box_Colour_FGV_States."Write") -> ()  [unwired: 8 in, 2 out]
          }
        }
        "Selected Task" <- w174
        n63 = Enqueue Element(queue=w178, element=w174, error in (no error)=w176) -> (queue out=w177:refnum<queue>, error out=w175:errorcluster)  [unwired: 1 in, 1 out]
      }
      event User Event {
        n64 = event-data() -> ("Stop Queue"=w211:bool)  [unwired: 1 in, 4 out]
        n65 = Enqueue Element At Opposite End(queue=w209, element=Intruction_Type_Definitions."Exit" ("Enum"), error in (no error)=w208) -> (queue out=w210:refnum<queue>, error out=w207:errorcluster)  [unwired: 1 in, 1 out]
      }
    }
  }
  n66 = while {
    tunnel: w46 -> [w214]
    tunnel: w47 -> [w272]
    tunnel: w50 -> [w270]
    tunnel: [w269] -> _
    tunnel: [w268] -> w40
    shift-right: [w261] -> _
    shift-left: T9 {"PING_A"=0, "PING_B"=0, "PING_C"=0, "PING_D"=0} -> [w263]
    shift-right: [w255] -> _
    shift-left: State_Type_Definitions,_for_0.26g_versions_and_later_3."Startup" ("Enum") -> [w258]
    shift-right: [w251] -> _
    shift-left: T8 {"xDistance"=0.0, "yDistance"=0.0, "wDistance"=0.0} -> [w253]
    shift-right: [w248] -> _
    shift-left: _ -> [w247]
    shift-right: [w244] -> _
    shift-left: T11 {"Recognized Object"=FALSE, "Object X coordinate"=0.0, "Object Y coordinate"=0.0} -> [w246]
    shift-right: [w241] -> _
    shift-left: T7 {"y Stepper Position"=0, "z Stepper Position"=0} -> [w243]
    shift-right: [w238] -> _
    shift-left: T6 {"Yaw"=0.0, "Compass"=0.0} -> [w240]
    shift-right: [w235] -> _
    shift-left: T3 {"Time up flag"=FALSE, "SET TIME TO CHECK"=0.0} -> [w237]
    shift-right: [w233] -> _
    shift-left: T20 {"yStepper desired"=0} -> [w234]
    shift-right: [w229] -> _
    shift-left: T5 {"Left IR Sensor"=0.0, "Arm IR Sensor"=0.0, "Bottom IR Sensor"=0.0} -> [w231]
    shift-right: [w227] -> _
    shift-left: T19 {"ySpeed"=0.0, "xSpeed"=0.0, "wSpeed"=0.0} -> [w228]
    shift-right: [w224] -> _
    shift-left: T4 {"Line Detected?"=FALSE, "S1"=0.0, "S2"=0.0, "S3"=0.0, "S4"=0.0} -> [w226]
    shift-right: [w222] -> _
    shift-left: _ -> [w221]
    shift-right: [w213] -> _
    shift-left: T1 {"Red"=FALSE, "Black"=FALSE, "Blue"=FALSE, "Yellow"=FALSE, "Green"=FALSE, "Unknown"=FALSE, "Image processing done"=FALSE, "Colour"=enum."None"} -> [w216]
    stop <- w260 stop-if-true
    # ">>> Box Colour Detection >>>"
    # ">>State Logic Queue Reference >>"
    # ">>Action Queue>>"
    # ">>State Logic Queue Reference >>"
    # ">>> Line Sensor Cluster>>>"
    # ">>> IR Sensors >>>"
    # ">>> Time cluster >>>"
    # ">>> Object detection >>>"
    # ">>> Yaw >>>"
    # ">>> Ultrasonic Sensors Detect >>>"
    # ">>> Encoders >>>"
    # ">>> Stepper position >>>"
    # ">>State Logic  >>"
    # ">> Item Selection Bias >>"
    # ">> Item Selection Bias >>"
    # ">> Item Selection Bias >>"
    # ">>State Logic  >>"
    # ">>> Motor control cluster >>>"
    # ">>> yStepper command>>>"
    # ">>True Stop Next State >>"
    # ">>Error  >>"
    # ">>Timeout>>"
    # ">>Action states Queue Reference >>"
    # "TOP LEVEL BASELINE (MAIN PROCESSING LOOP)"
    n67 = Wait (ms)(milliseconds to wait=u32 25) -> ()  [unwired: 1 out]
    n68 = Dequeue Element(queue=w272, timeout in ms (-1)=0, error in (no error)=w270) -> (queue out=w264:refnum<queue>, element=w271:string, error out=w265:errorcluster)  [unwired: 1 out]
    "Action State" <- w271
    n69 = case shown="\"READ STEPPER VALUES\"" w271 {
      tunnel: [_ _ _ _ _ _ _ _ _ _ _ _ _ _ _ _ _ _ _ _ 0 w3641 _ _ _ _ _ _ _ _ _ _ _ _ _ _ _ _ _ _ _ _ _ _ _ _ _ _ _ _ _ _ _ _ _ _ _] -> w267
      tunnel: w264 -> [_ _ _ _ _ _ _ _ _ _ _ _ _ _ _ _ _ _ _ _ _ _ _ _ _ _ _ _ _ _ _ _ _ _ _ _ _ _ _ _ _ _ _ _ _ _ _ _ _ _ _ _ _ _ _ _ _]
      tunnel: w263 -> [w3313 w3325 w3340 w3354 w3374 w3389 w3403 w3417 w3433 w3448 w3462 w3472 w3490 w3507 w3522 w3537 w3561 w3571 w3602 w3615 w3629 w3642 w3654 w3667 w3687 w3722 w3759 w3773 w3784 w3796 w3809 w3824 w3840 w3852 w3864 w3884 w3907 w3918 w3934 w3965 w3975 w3988 w4001 w4014 w4024 w4042 w4052 w4071 w4080 w4096 w4112 w4128 w4144 w4160 w4174 w4189 w4209]
      tunnel: [w3313 w3325 w3340 w3354 w3374 w3389 w3403 w3417 w3433 w3448 w3462 w3472 w3490 w3508 w3522 w3537 w3561 w3571 w3603 w3615 w3629 w3642 w3654 w3667 w3687 w3721 w3758 w3773 w3784 w3796 w3809 w3824 w3840 w3852 w3864 w3884 w3907 w3918 w3934 w3965 w3975 w3988 w4001 w4014 w4024 w4042 w4052 w4071 w4080 w4096 w4112 w4128 w4144 w4160 w4174 w4189 w4209] -> w262
      tunnel: [TRUE TRUE _ _ _ _ _ _ _ _ _ _ _ _ _ _ _ _ _ _ _ _ _ _ _ _ _ _ _ _ _ _ _ _ _ _ _ _ _ _ _ _ _ _ _ _ _ _ _ _ _ _ _ _ _ _ _] -> w260
      tunnel: w258 -> [w3311 w3323 w3339 w3353 w3373 w3388 w3402 w3416 w3432 w3447 w3461 w3471 w3489 w3506 w3521 w3535 w3554 w3570 w3601 w3614 w3626 w3639 w3653 w3666 w3686 w3720 w3757 w3772 w3783 w3795 w3801 w3823 w3839 w3851 w3863 w3883 w3906 w3917 w3928 w3959 w3974 w3987 w4000 w4013 w4023 w4033 w4051 w4070 w4079 w4095 w4111 w4127 w4143 w4159 w4173 w4179 w4197]
      tunnel: [_ _ _ _ _ _ _ _ _ _ _ _ _ _ _ _ _ _ _ _ _ TRUE _ _ _ _ _ _ _ _ _ _ _ _ _ _ _ _ _ _ _ _ _ _ _ _ _ _ _ _ _ _ _ _ _ _ _] -> w257
      tunnel: [w3311 w3323 w3339 w3353 w3373 w3388 w3402 w3416 w3432 w3447 w3461 w3471 w3489 w3506 w3521 w3535 w3554 w3570 w3601 w3614 w3626 w3639 w3653 w3666 w3686 w3720 w3757 w3772 w3783 w3795 w3801 w3823 w3839 w3851 w3863 w3883 w3906 w3917 w3928 w3959 w3974 w3987 w4000 w4013 w4023 w4033 w4051 w4070 w4079 w4095 w4111 w4127 w4143 w4159 w4173 w4179 w4197] -> w256
      tunnel: w253 -> [w3310 w3322 w3338 w3356 w3372 w3387 w3401 w3415 w3431 w3446 w3460 w3473 w3488 w3505 w3523 w3539 w3556 w3572 w3600 w3616 w3625 w3638 w3655 w3668 w3682 w3711 w3747 w3771 w3786 w3797 w3806 w3825 w3841 w3853 w3865 w3885 w3908 w3920 w3932 w3963 w3977 w3990 w4003 w4016 w4026 w4037 w4054 w4073 w4082 w4098 w4114 w4130 w4146 w4162 w4176 w4181 w4202]
      tunnel: [w3310 w3322 w3338 w3356 w3372 w3387 w3401 w3415 w3431 w3446 w3460 w3473 w3487 w3505 w3523 w3539 w3556 w3572 w3599 w3616 w3625 w3638 w3655 w3668 w3682 w3710 w3746 w3771 w3786 w3797 w3806 w3825 w3841 w3853 w3865 w3885 w3908 w3920 w3932 w3963 w3977 w3990 w4003 w4016 w4026 w4037 w4054 w4073 w4082 w4098 w4114 w4130 w4146 w4162 w4176 w4181 w4202] -> w252
      tunnel: w246 -> [w3309 w3321 w3337 w3355 w3371 w3386 w3400 w3414 w3430 w3445 w3458 w3470 w3486 w3504 w3516 w3538 w3555 w3569 w3591 w3613 w3624 w3637 w3652 w3665 w3685 w3715 w3752 w3769 w3785 w3794 w3807 w3822 w3838 w3847 w3862 w3881 w3901 w3919 w3933 w3964 w3976 w3989 w4002 w4015 w4025 w4036 w4053 w4072 w4081 w4097 w4113 w4129 w4145 w4161 w4175 w4180 w4201]
      tunnel: [w3309 w3321 w3337 w3355 w3371 w3386 w3400 w3414 w3430 w3445 w3458 w3470 w3486 w3504 w3516 w3538 w3555 w3569 w3590 w3613 w3624 w3637 w3652 w3665 w3684 w3714 w3751 w3769 w3785 w3794 w3807 w3822 w3838 w3847 w3862 w3880 w3901 w3919 w3933 w3964 w3976 w3989 w4002 w4015 w4025 w4036 w4053 w4072 w4081 w4097 w4113 w4129 w4145 w4161 w4175 w4180 w4201] -> w245
      tunnel: w243 -> [w3308 w3320 w3336 w3357 w3370 w3385 w3399 w3413 w3429 w3444 w3457 w3469 w3485 w3503 w3524 w3540 w3557 w3568 w3596 w3612 w3623 w3636 w3651 w3664 w3681 w3706 w3742 w3768 w3782 w3793 w3805 w3821 w3837 w3850 w3861 w3886 w3909 w3921 w3931 w3962 w3973 w3986 w3999 w4012 w4027 w4038 w4055 w4069 w4083 w4099 w4115 w4131 w4147 w4163 w4177 w4182 w4203]
      tunnel: [w3308 w3320 w3336 w3357 w3370 w3385 w3399 w3413 w3429 w3444 w3457 w3469 w3485 w3503 w3524 w3540 w3557 w3568 w3595 w3612 w3623 w3636 w3651 w3664 w3681 w3705 w3741 w3768 w3782 w3793 w3805 w3821 w3837 w3850 w3861 w3886 w3909 w3921 w3931 w3962 w3973 w3986 w3999 w4012 w4027 w4038 w4055 w4068 w4083 w4099 w4115 w4131 w4147 w4163 w4177 w4182 w4203] -> w242
      tunnel: w240 -> [w3307 w3319 w3334 w3358 w3368 w3383 w3397 w3412 w3427 w3442 w3456 w3468 w3484 w3496 w3519 w3541 w3558 w3567 w3586 w3611 w3622 w3635 w3650 w3663 w3680 w3702 w3738 w3767 w3779 w3792 w3804 w3820 w3836 w3849 w3860 w3887 w3910 w3922 w3930 w3961 w3972 w3983 w3996 w4009 w4028 w4039 w4056 w4063 w4084 w4100 w4116 w4132 w4148 w4164 w4178 w4183 w4204]
      tunnel: [w3307 w3319 w3334 w3358 w3368 w3383 w3397 w3412 w3427 w3442 w3456 w3468 w3484 w3496 w3518 w3541 w3558 w3567 w3585 w3611 w3622 w3635 w3650 w3663 w3680 w3701 w3737 w3767 w3779 w3792 w3804 w3820 w3836 w3849 w3860 w3887 w3910 w3922 w3930 w3961 w3972 w3983 w3996 w4009 w4028 w4039 w4056 w4063 w4084 w4100 w4116 w4132 w4148 w4164 w4178 w4183 w4204] -> w239
      tunnel: w237 -> [w3305 w3318 w3335 w3359 w3369 w3384 w3398 w3411 w3428 w3443 w3455 w3467 w3483 w3495 w3515 w3542 w3559 w3566 w3582 w3608 w3621 w3634 w3649 w3662 w3679 w3699 w3735 w3765 w3778 w3791 w3803 w3819 w3835 w3848 w3859 w3888 w3911 w3923 w3929 w3960 w3971 w3982 w3995 w4008 w4029 w4040 w4057 w4062 w4078 w4094 w4110 w4126 w4142 w4158 w4172 w4184 w4205]
      tunnel: [w3305 w3318 w3335 w3359 w3369 w3384 w3398 w3411 w3428 w3443 w3455 w3467 w3483 w3495 w3515 w3542 w3559 w3566 w3582 w3608 w3621 w3634 w3649 w3662 w3678 w3698 w3734 w3765 w3778 w3791 w3803 w3819 w3835 w3848 w3859 w3888 w3911 w3923 w3929 w3960 w3971 w3982 w3995 w4008 w4029 w4040 w4057 w4062 w4078 w4092 w4108 w4124 w4140 w4157 w4171 w4184 w4205] -> w236
      tunnel: w234 -> [_ _ _ _ _ _ _ _ _ _ _ _ _ _ _ _ _ _ _ _ _ _ _ _ _ _ _ _ _ _ _ _ _ _ _ _ _ _ _ _ _ _ _ _ _ _ w4048 _ _ _ _ _ _ _ _ _ _]
      tunnel: [w3304 w3317 w3329 w3349 w3363 w3378 w3393 w3407 w3423 w3437 w3452 w3466 w3477 w3494 w3512 w3533 w3560 w3565 w3579 w3607 w3620 w3633 w3648 w3659 w3672 w3692 w3726 w3764 w3777 w3790 w3808 w3813 w3829 w3845 w3857 w3876 w3904 w3915 w3935 w3966 w3970 w3981 w3994 w4007 w4020 w4041 w4046 w4061 w4077 w4090 w4106 w4122 w4138 w4155 w4168 w4188 w4208] -> w230
      tunnel: w231 -> [w3304 w3317 w3329 w3349 w3363 w3378 w3393 w3407 w3423 w3437 w3452 w3466 w3477 w3494 w3512 w3534 w3560 w3565 w3579 w3607 w3620 w3633 w3648 w3659 w3672 w3693 w3727 w3764 w3777 w3790 w3808 w3813 w3829 w3845 w3857 w3876 w3904 w3915 w3935 w3966 w3970 w3981 w3994 w4007 w4020 w4041 w4046 w4061 w4077 w4090 w4106 w4122 w4138 w4155 w4168 w4188 w4208]
      tunnel: w228 -> [_ _ _ _ _ _ _ _ w3422 _ _ _ _ _ _ _ _ _ _ _ _ _ _ _ _ _ _ _ _ _ _ _ _ _ _ _ _ _ _ _ _ _ _ _ _ _ _ _ _ _ _ _ _ _ _ _ _]
      tunnel: w226 -> [w3303 w3316 w3328 w3343 w3362 w3377 w3392 w3406 w3420 w3436 w3451 w3465 w3476 w3493 w3511 w3529 w3553 w3564 w3577 w3606 w3619 w3632 w3647 w3658 w3675 w3695 w3730 w3763 w3776 w3789 w3800 w3812 w3828 w3844 w3856 w3874 w3903 w3914 w3926 w3958 w3969 w3980 w3993 w4006 w4019 w4032 w4045 w4060 w4076 w4089 w4105 w4121 w4137 w4154 w4167 w4187 w4207]
      tunnel: [w3303 w3316 w3328 w3343 w3362 w3377 w3392 w3406 w3420 w3436 w3451 w3465 w3476 w3493 w3511 w3529 w3552 w3564 w3577 w3606 w3619 w3632 w3647 w3658 w3674 w3694 w3729 w3763 w3776 w3789 w3800 w3812 w3828 w3844 w3856 w3874 w3903 w3914 w3926 w3958 w3969 w3980 w3993 w4006 w4019 w4032 w4045 w4060 w4076 w4089 w4105 w4121 w4137 w4154 w4167 w4187 w4207] -> w225
      tunnel: [_ _ _ _ _ _ _ _ _ _ _ _ _ _ _ _ _ _ _ _ _ _ _ _ _ _ _ _ _ _ _ _ _ _ _ w3868 w3898 _ _ _ _ _ _ _ _ _ _ _ _ _ _ _ _ _ _ _ _] -> w223
      tunnel: w221 -> [w3302 w3315 w3327 w3342 w3361 w3376 w3391 w3405 w3419 w3435 w3450 w3464 w3475 w3492 w3510 w3528 w3544 w3563 w3575 w3605 w3618 w3631 w3646 w3657 w3676 w3696 w3731 w3762 w3775 w3788 w3799 w3811 w3827 w3843 w3855 w3870 w3902 w3913 w3925 w3957 w3968 w3979 w3992 w4005 w4018 w4031 w4044 w4059 w4075 w4088 w4104 w4120 w4136 w4153 w4166 w4186 w4206]
      tunnel: [w3302 w3315 w3327 w3342 w3361 w3376 w3391 w3405 w3419 w3435 w3450 w3464 w3475 w3492 w3510 w3528 w3544 w3563 w3575 w3605 w3618 w3631 w3646 w3657 w3676 w3696 w3731 w3762 w3775 w3788 w3799 w3811 w3827 w3843 w3855 w3870 w3902 w3913 w3925 w3957 w3968 w3979 w3992 w4005 w4018 w4031 w4044 w4059 w4075 w4088 w4104 w4120 w4136 w4153 w4166 w4186 w4206] -> w220
      tunnel: w216 -> [w3301 w3314 w3326 w3341 w3360 w3375 w3390 w3404 w3418 w3434 w3449 w3463 w3474 w3491 w3509 w3525 w3543 w3562 w3574 w3604 w3617 w3630 w3645 w3656 w3671 w3689 w3725 w3761 w3774 w3787 w3798 w3810 w3826 w3842 w3854 w3873 w3896 w3912 w3924 w3956 w3967 w3978 w3991 w4004 w4017 w4030 w4043 w4058 w4074 w4087 w4103 w4119 w4135 w4152 w4165 w4185 w4200]
      tunnel: [w3301 w3314 w3326 w3341 w3360 w3375 w3390 w3404 w3418 w3434 w3449 w3463 w3474 w3491 w3509 w3525 w3543 w3562 w3574 w3604 w3617 w3630 w3645 w3656 w3670 w3689 w3725 w3761 w3774 w3787 w3798 w3810 w3826 w3842 w3854 w3873 w3889 w3912 w3924 w3955 w3967 w3978 w3991 w4004 w4017 w4030 w4043 w4058 w4074 w4087 w4103 w4119 w4135 w4152 w4165 w4185 w4199] -> w215
      frame "Exit" {
        # ">>State Logic  >>"
        # ">>> Time cluster >>>"
        # ">>> Yaw >>>"
        # ">>> Stepper position >>>"
        # ">>> Encoders >>>"
        # ">>> Object detection >>>"
        # ">>> Ultrasonic Sensors Detect >>>"
        n70 = call "Imaq Dispose"("All Images? (No)"=TRUE) -> ()  [unwired: 5 in, 1 out]
      }
      frame "----Movement States----" {
        # ">>State Logic  >>"
        # ">>> Time cluster >>>"
        # ">>> Yaw >>>"
        # ">>> Stepper position >>>"
        # ">>> Encoders >>>"
        # ">>> Object detection >>>"
        # ">>> Ultrasonic Sensors Detect >>>"
      }
      frame "FORWARD" {
        # "High voltage values: 30\nMid voltage values: 40\nLow voltage values: 50"
        # ">>State Logic  >>"
        # ">>> Time cluster >>>"
        # ">>> Yaw >>>"
        # ">>> Stepper position >>>"
        # ">>> Encoders >>>"
        # ">>> Object detection >>>"
        # ">>> Ultrasonic Sensors Detect >>>"
        n71 = Unbundle By Name(w3334) -> ("Yaw"=w3330:dbl)
        n72 = call "MOTOR CONTROL WITH PID AE.vi"("Yaw"=w3330, "Speed"=30.0, "Direction"=MOTOR_CONTROL_WITH_PID_AE_DIRECTION_TYPE_DEF."y-axis movement", "AE Mode"=MOTOR_CONTROL_WITH_PID_AE_DATA_MODE_TYPE_DEF."Write to AE") -> ()  [unwired: 1 out]
      }
      frame "FORWARD - IR ASSIST" {
        # "Algorithm sensitivity"
        # "Distance to maintain from wall"
        # ">>State Logic  >>"
        # ">>> Time cluster >>>"
        # ">>> Yaw >>>"
        # ">>> Stepper position >>>"
        # ">>> Encoders >>>"
        # ">>> Object detection >>>"
        # ">>> Ultrasonic Sensors Detect >>>"
        n73 = Unbundle By Name(w3349) -> ("Left IR Sensor"=w3348:dbl)
        n74 = Subtract(x=w3348, y=20.0) -> (x-y=w3346:dbl)
        n75 = Multiply(x=w3346, y=0.2) -> (x*y=w3344:dbl)
        n76 = call "MOTOR CONTROL WITH PID AE.vi"("Yaw"=w3344, "Speed"=35.0, "Direction"=MOTOR_CONTROL_WITH_PID_AE_DIRECTION_TYPE_DEF."y-axis movement", "AE Mode"=MOTOR_CONTROL_WITH_PID_AE_DATA_MODE_TYPE_DEF."Write to AE") -> ()  [unwired: 1 out]
      }
      frame "LEFT" {
        # ">>State Logic  >>"
        # ">>> Time cluster >>>"
        # ">>> Yaw >>>"
        # ">>> Stepper position >>>"
        # ">>> Encoders >>>"
        # ">>> Object detection >>>"
        # ">>> Ultrasonic Sensors Detect >>>"
        n77 = Unbundle By Name(w3368) -> ("Yaw"=w3365:dbl)
        n78 = call "MOTOR CONTROL WITH PID AE.vi"("Yaw"=w3365, "Speed"=-25.0, "Direction"=MOTOR_CONTROL_WITH_PID_AE_DIRECTION_TYPE_DEF."x-axis movement", "AE Mode"=MOTOR_CONTROL_WITH_PID_AE_DATA_MODE_TYPE_DEF."Write to AE") -> ()  [unwired: 1 out]
      }
      frame "RIGHT" {
        # ">>> Time cluster >>>"
        # ">>> Yaw >>>"
        # ">>> Stepper position >>>"
        # ">>> Encoders >>>"
        # ">>> Object detection >>>"
        # ">>> Ultrasonic Sensors Detect >>>"
        n79 = Unbundle By Name(w3383) -> ("Yaw"=w3379:dbl)
        n80 = call "MOTOR CONTROL WITH PID AE.vi"("Yaw"=w3379, "Speed"=25.0, "Direction"=MOTOR_CONTROL_WITH_PID_AE_DIRECTION_TYPE_DEF."x-axis movement", "AE Mode"=MOTOR_CONTROL_WITH_PID_AE_DATA_MODE_TYPE_DEF."Write to AE") -> ()  [unwired: 1 out]
      }
      frame "R-ACW" {
        # ">>> IR Sensors >>>"
        # ">>> Time cluster >>>"
        # ">>> Yaw >>>"
        # ">>> Stepper position >>>"
        # ">>> Encoders >>>"
        # ">>> Object detection >>>"
        # ">>> Ultrasonic Sensors Detect >>>"
        n81 = call "MOTOR CONTROL WITH PID AE.vi"("Speed"=10.0, "Direction"=MOTOR_CONTROL_WITH_PID_AE_DIRECTION_TYPE_DEF."rotation", "AE Mode"=MOTOR_CONTROL_WITH_PID_AE_DATA_MODE_TYPE_DEF."Write to AE") -> ()  [unwired: 1 in, 1 out]
      }
      frame "R-CW" {
        (unwired) -0.2 ("Speed")
        # ">>> Time cluster >>>"
        # ">>> Yaw >>>"
        # ">>> Stepper position >>>"
        # ">>> Encoders >>>"
        # ">>> Object detection >>>"
        # ">>> Ultrasonic Sensors Detect >>>"
        n82 = call "MOTOR CONTROL WITH PID AE.vi"("Speed"=-10.0, "Direction"=MOTOR_CONTROL_WITH_PID_AE_DIRECTION_TYPE_DEF."rotation", "AE Mode"=MOTOR_CONTROL_WITH_PID_AE_DATA_MODE_TYPE_DEF."Write to AE") -> ()  [unwired: 1 in, 1 out]
      }
      frame "X AXIS - SLOW" {
        # ">>> Line Sensor Cluster>>>"
        # ">>> IR Sensors >>>"
        # ">>> Time cluster >>>"
        # ">>> Yaw >>>"
        # ">>> Stepper position >>>"
        # ">>> Encoders >>>"
        # ">>> Object detection >>>"
        # ">>> Ultrasonic Sensors Detect >>>"
        n83 = Unbundle By Name(w3422) -> ("xSpeed"=w3421:dbl)
        n84 = Unbundle By Name(w3427) -> ("Yaw"=w3424:dbl)
        n85 = call "MOTOR CONTROL WITH PID AE.vi"("Yaw"=w3424, "Speed"=w3421, "Direction"=MOTOR_CONTROL_WITH_PID_AE_DIRECTION_TYPE_DEF."x-axis movement", "AE Mode"=MOTOR_CONTROL_WITH_PID_AE_DATA_MODE_TYPE_DEF."Write to AE") -> ()  [unwired: 1 out]
      }
      frame "REVERSE" {
        # ">>> Time cluster >>>"
        # ">>> Yaw >>>"
        # ">>> Stepper position >>>"
        # ">>> Encoders >>>"
        # ">>> Object detection >>>"
        # ">>> Ultrasonic Sensors Detect >>>"
        n86 = Unbundle By Name(w3442) -> ("Yaw"=w3438:dbl)
        n87 = call "MOTOR CONTROL WITH PID AE.vi"("Yaw"=w3438, "Speed"=-40.0, "Direction"=MOTOR_CONTROL_WITH_PID_AE_DIRECTION_TYPE_DEF."y-axis movement", "AE Mode"=MOTOR_CONTROL_WITH_PID_AE_DATA_MODE_TYPE_DEF."Write to AE") -> ()  [unwired: 1 out]
      }
      frame "STOP" {
        n88 = Wait (ms)(milliseconds to wait=u32 100) -> ()  [unwired: 1 out]
        n89 = call "MOTOR CONTROL WITH PID AE.vi"("Direction"=MOTOR_CONTROL_WITH_PID_AE_DIRECTION_TYPE_DEF."stop", "AE Mode"=MOTOR_CONTROL_WITH_PID_AE_DATA_MODE_TYPE_DEF."Write to AE") -> ()  [unwired: 2 in, 1 out]
      }
      frame "----SENSOR READING---- " {
      }
      frame "READ ENCODERS" {
        # ">>> Time cluster >>>"
        # ">>> Yaw >>>"
        # ">>> Stepper position >>>"
        # ">>> Object detection >>>"
        # ">>> Current encoder distance >>>"
        # ">>> Ultrasonic Sensors Detect >>>"
        n90 = call "MOTOR CONTROL WITH PID AE.vi"("AE Mode"=MOTOR_CONTROL_WITH_PID_AE_DATA_MODE_TYPE_DEF."Read from AE") -> ("Speed & distance"=w3481:T15)  [unwired: 3 in]
        n91 = Unbundle By Name(w3481) -> ("xDistance"=w3480:dbl, "yDistance"=w3479:dbl, "wDistance"=w3478:dbl)
        n92 = Bundle By Name(cluster=w3488, "xDistance"=w3480, "yDistance"=w3479, "wDistance"=w3478) -> (w3487:T8)
      }
      frame "READ ULTRASONIC" {
        (unwired) navX_type_def."Read Values" ("Mode")
        (unwired) MOTOR_CONTROL_NO_PID_Type_Def."Latch" ("Direction")
        # ">>> Line Sensor Cluster>>>"
        # ">>> IR Sensors >>>"
        # ">>State Logic  >>"
        # ">>> Time cluster >>>"
        # ">>> Ultrasonic Sensors Detect >>>"
        # ">>> Object detection >>>"
        # ">>> Encoders >>>"
        # ">>> Stepper position >>>"
        # ">>> Yaw >>>"
        n93 = call "Arduino Interfacing VI.vi"("AE Mode"=Arduino_Interfacing."Read From Arduino") -> ("Arduino Data"=w3501:T17)  [unwired: 3 in, 1 out]
        n94 = Unbundle By Name(w3501) -> ("PING A"=w3500:u8, "PING B"=w3499:u8, "PING C"=w3498:u8, "PING D"=w3497:u8)
        n95 = Bundle By Name(cluster=w3507, "PING_A"=w3500, "PING_B"=w3499, "PING_C"=w3498, "PING_D"=w3497) -> (w3508:T9)
      }
      frame "READ NAVX" {
        # ">> Item Selection Bias >>"
        # ">>State Logic  >>"
        # ">>> Line Sensor Cluster>>>"
        # ">>> IR Sensors >>>"
        # ">>> Time cluster >>>"
        # ">>> Yaw >>>"
        # ">>> Ultrasonic Sensors Detect >>>"
        # ">>> Object detection >>>"
        # ">>> Encoders >>>"
        # ">>> Stepper position >>>"
        n96 = call "navX reading VI.vi"("Mode"=navX_type_def."Read Values") -> ("NavX Readings"=w3514:T16)  [unwired: 2 in, 3 out]
        n97 = Unbundle By Name(w3514) -> ("Heading"=w3513:dbl)
        n98 = Unbundle By Name(w3514) -> ("Yaw"=w3517:dbl)
        n99 = Bundle By Name(cluster=w3519, "Yaw"=w3517, "Compass"=w3513) -> (w3518:T6)
      }
      frame "READ IR" {
        w3527 = T40 [enum."B/AI2"] items=["Not Connected", "AudioIn/Left", "AudioIn/Right", "C/AI0", "C/AI1", "A/AI0", "A/AI1", "A/AI2", "A/AI3", "A/AI4", "A/AI5", "A/AI6", "A/AI7", "B/AI0", "B/AI1", "B/AI2", "B/AI3", "B/AI4", "B/AI5", "B/AI6", "B/AI7", "AI/AI0", "AI/AI1", "AI/AI2", "AI/AI3", "A/AI0 (DIFF)", "A/AI1 (DIFF)", "A/AI2 (DIFF)", "A/AI3 (DIFF)", "B/AI0 (DIFF)", "B/AI1 (DIFF)", "B/AI2 (DIFF)", "B/AI3 (DIFF)"] ("AI Channel")
        w3531 = T40 [enum."B/AI1"] items=["Not Connected", "AudioIn/Left", "AudioIn/Right", "C/AI0", "C/AI1", "A/AI0", "A/AI1", "A/AI2", "A/AI3", "A/AI4", "A/AI5", "A/AI6", "A/AI7", "B/AI0", "B/AI1", "B/AI2", "B/AI3", "B/AI4", "B/AI5", "B/AI6", "B/AI7", "AI/AI0", "AI/AI1", "AI/AI2", "AI/AI3", "A/AI0 (DIFF)", "A/AI1 (DIFF)", "A/AI2 (DIFF)", "A/AI3 (DIFF)", "B/AI0 (DIFF)", "B/AI1 (DIFF)", "B/AI2 (DIFF)", "B/AI3 (DIFF)"] ("AI Channel")
        w3536 = T40 [enum."B/AI0"] items=["Not Connected", "AudioIn/Left", "AudioIn/Right", "C/AI0", "C/AI1", "A/AI0", "A/AI1", "A/AI2", "A/AI3", "A/AI4", "A/AI5", "A/AI6", "A/AI7", "B/AI0", "B/AI1", "B/AI2", "B/AI3", "B/AI4", "B/AI5", "B/AI6", "B/AI7", "AI/AI0", "AI/AI1", "AI/AI2", "AI/AI3", "A/AI0 (DIFF)", "A/AI1 (DIFF)", "A/AI2 (DIFF)", "A/AI3 (DIFF)", "B/AI0 (DIFF)", "B/AI1 (DIFF)", "B/AI2 (DIFF)", "B/AI3 (DIFF)"] ("AI Channel")
        # ">>> Line Sensor Cluster>>>"
        # ">>> IR Sensors >>>"
        # ">>State Logic  >>"
        # ">>> Time cluster >>>"
        # ">>> Ultrasonic Sensors Detect >>>"
        # ">>> Object detection >>>"
        # ">>> Encoders >>>"
        # ">>> Stepper position >>>"
        # ">>> Yaw >>>"
        n100 = call <vilib>:"Sharp IR.vi"("AI Channel"=w3536) -> ("Sharp IR Distance"=w3532:dbl)  [unwired: 8 in, 2 out]
        n101 = call <vilib>:"Sharp IR.vi"("AI Channel"=w3531) -> ("Sharp IR Distance"=w3530:dbl)  [unwired: 8 in, 2 out]
        n102 = call <vilib>:"Sharp IR.vi"("AI Channel"=w3527) -> ("Sharp IR Distance"=w3526:dbl)  [unwired: 8 in, 2 out]
        n103 = Bundle By Name(cluster=w3534, "Left IR Sensor"=w3532, "Arm IR Sensor"=w3530, "Bottom IR Sensor"=w3526) -> (w3533:T5)
      }
      frame "READ LINE SENSOR" {
        # ">>> IR Sensors >>>"
        # ">>> Line Sensor Cluster>>>"
        # ">>State Logic  >>"
        # ">>> Time cluster >>>"
        # ">>> Object detection >>>"
        # ">>> Yaw >>>"
        # ">>> Ultrasonic Sensors Detect >>>"
        # ">>> Encoders >>>"
        # ">>> Stepper position >>>"
        n104 = call "Line Sensor AE.vi"("AE State"=Line_Sensor_AE_Type_Def."READ FROM LINE SENSORS") -> ("Line Detected?"=w3550:bool, "Line Sensor Raw Values"=w3549:T42)
        n105 = Unbundle By Name(w3549) -> ("S1"=w3548:dbl, "S2"=w3547:dbl, "S3"=w3546:dbl, "S4"=w3545:dbl)
        n106 = Bundle By Name(cluster=w3553, "Line Detected?"=w3550, "S1"=w3548, "S2"=w3547, "S3"=w3546, "S4"=w3545) -> (w3552:T4)
      }
      frame "----SYSTEM MODES----" {
        (unwired) I2C_MASTER_Type_Def."Last State" ("Arduino Mode")
        # ">>> Object detection >>>"
        # ">>> Yaw >>>"
        # ">>> Ultrasonic Sensors Detect >>>"
        # ">>> Encoders >>>"
        # ">>> Stepper position >>>"
      }
      frame "INIT" {
        w3597 = u8 0
        w3598 = 0.0
        # ">>> IR Sensors >>>"
        # ">>> IR Sensors >>>"
        # ">>> Line Sensor Cluster>>>"
        # ">>> Time cluster >>>"
        # ">>> Object detection >>>"
        # ">>> Yaw >>>"
        # ">>> Ultrasonic Sensors Detect >>>"
        # ">>> Encoders >>>"
        # ">>> Stepper position >>>"
        # ">>State Logic  >>"
        n107 = call "Arduino Interfacing VI.vi"("AE Mode"=Arduino_Interfacing."Initialize") -> ()  [unwired: 3 in, 2 out]
        n108 = call "FGV Bool.vi"("Init/Read/Write State"=States_for_Action_Engine."Initialize") -> ()  [unwired: 2 in, 2 out]
        n109 = call "Elasped Timer.vi"("Action"=Elapsed_timer_control."Initialize") -> ()  [unwired: 7 in, 4 out]
        n110 = call "MOTOR CONTROL WITH PID AE.vi"("AE Mode"=MOTOR_CONTROL_WITH_PID_AE_DATA_MODE_TYPE_DEF."Init AE") -> ()  [unwired: 3 in, 1 out]
        n111 = call "IMAQ Reference AE.vi"("IMAQ AE States"=IMAQ_Reference_AE."Initialize AE") -> ()  [unwired: 1 in, 2 out]
        n112 = call "Line Sensor AE.vi"("AE State"=Line_Sensor_AE_Type_Def."INIT AE") -> ()  [unwired: 2 out]
        n113 = Bundle By Name(cluster=w3591, "Recognized Object"=FALSE, "Object X coordinate"=0.0, "Object Y coordinate"=0.0) -> (w3590:T11)
        n114 = Bundle By Name(cluster=w3596, "y Stepper Position"=u8 0, "z Stepper Position"=u8 0) -> (w3595:T7)
        n115 = Bundle By Name(cluster=w3600, "xDistance"=w3598, "yDistance"=w3598, "wDistance"=w3598) -> (w3599:T8)
        n116 = Bundle By Name(cluster=w3602, "PING_A"=w3597, "PING_B"=w3597, "PING_C"=w3597, "PING_D"=w3597) -> (w3603:T9)
        n117 = invoke class="VI" method="Default Vals.Reinit All"() -> ()  [unwired: 3 in, 3 out]
        n118 = Bundle By Name(cluster=w3586, "Yaw"=0.0) -> (w3585:T6)
        n119 = call "Box Colour FGV.vi"("Init/R/W State"=Box_Colour_FGV_States."Initialize") -> ()  [unwired: 9 in, 2 out]
      }
      frame "ARDUINO - ULTRASONIC" {
        # ">>> Time cluster >>>"
        # ">>> Line Sensor Cluster>>>"
        # ">>> Object detection >>>"
        # ">>> Yaw >>>"
        # ">>> Ultrasonic Sensors Detect >>>"
        # ">>> Encoders >>>"
        # ">>> Stepper position >>>"
        # ">>State Logic  >>"
        n120 = call "Arduino Interfacing VI.vi"("Data to Write"=I2C_MASTER_WRITE_NEW_Type_Def."Ultrasonic sensors", "AE Mode"=Arduino_Interfacing."Write to Arduino") -> ()  [unwired: 2 in, 2 out]
      }
      frame "NAVX CALIBRATE" {
        # ">>> Object detection >>>"
        # ">>> Yaw >>>"
        # ">>> Ultrasonic Sensors Detect >>>"
        # ">>> Encoders >>>"
        # ">>> Stepper position >>>"
        # ">>State Logic  >>"
        # "Adds a 15 second delay to the startup process \nfor the NavX to calibrate"
        n121 = Wait (ms)(milliseconds to wait=u32 1000) -> ()  [unwired: 1 out]
      }
      frame "NO ACTION", Default {
        (unwired) u8 0 ("y Stepper value")
        (unwired) TRUE ("Latch")
        (unwired) navX_type_def."Read Values" ("Mode")
        (unwired) MOTOR_CONTROL_NO_PID_Type_Def."Latch" ("Direction")
        # ">>> Object detection >>>"
        # ">>> Yaw >>>"
        # ">>> Ultrasonic Sensors Detect >>>"
        # ">>> Encoders >>>"
        # ">>> Stepper position >>>"
        # ">>State Logic  >>"
        n122 = case shown="\"Idle\"" w3639 {
          tunnel: [0 100] -> w3641
          frame "Startup", Default {
          }
          frame "Idle" {
          }
        }
      }
      frame "----RESET CASES----" {
        (unwired) I2C_MASTER_Type_Def."Last State" ("Arduino Mode")
        # ">>> Object detection >>>"
        # ">>> Yaw >>>"
        # ">>> Ultrasonic Sensors Detect >>>"
        # ">>> Encoders >>>"
        # ">>> Stepper position >>>"
        # ">>State Logic  >>"
      }
      frame "RESET ENCODERS" {
        # ">>> Object detection >>>"
        # ">>> Yaw >>>"
        # ">>> Ultrasonic Sensors Detect >>>"
        # ">>> Encoders >>>"
        # ">>> Stepper position >>>"
        # ">>State Logic  >>"
        n123 = call "MOTOR CONTROL WITH PID AE.vi"("Direction"=MOTOR_CONTROL_WITH_PID_AE_DIRECTION_TYPE_DEF."reset encoders", "AE Mode"=MOTOR_CONTROL_WITH_PID_AE_DATA_MODE_TYPE_DEF."Write to AE") -> ()  [unwired: 2 in, 1 out]
      }
      frame "RESET FLAGS" {
        w3669 = FALSE ("Line Detected?")
        # ">>> Line Sensor Cluster>>>"
        # ">>> IR Sensors >>>"
        # ">>> Time cluster >>>"
        # ">>> Object detection >>>"
        # ">>> Yaw >>>"
        # ">>> Ultrasonic Sensors Detect >>>"
        # ">>> Encoders >>>"
        # ">>> Stepper position >>>"
        # ">>> Line Sensor Cluster>>>"
        # ">>> IR Sensors >>>"
        # ">>> Time cluster >>>"
        # ">>> Object detection >>>"
        # ">>> Yaw >>>"
        # ">>> Ultrasonic Sensors Detect >>>"
        # ">>> Encoders >>>"
        # ">>> Stepper position >>>"
        # "Resets BOOLEAN FLAGS only"
        n124 = Wait (ms)(milliseconds to wait=u32 20) -> ()  [unwired: 1 out]
        n125 = Bundle By Name(cluster=w3685, "Recognized Object"=FALSE) -> (w3684:T11)
        n126 = Bundle By Name(cluster=w3675, "Line Detected?"=FALSE) -> (w3674:T4)
        n127 = Bundle By Name(cluster=w3679, "Time up flag"=FALSE) -> (w3678:T3)
        n128 = Bundle By Name(cluster=w3671, "Red"=w3669, "Black"=w3669, "Blue"=w3669, "Yellow"=w3669, "Green"=w3669, "Unknown"=w3669, "Image processing done"=w3669) -> (w3670:T1)
      }
      frame "RESET SENSOR VALUES" {
        w3690 = 0.0 ("S4")
        w3691 = 0.0 ("S4")
        # "Resets SENSOR VALUES only"
        # ">>> Line Sensor Cluster>>>"
        # ">>> IR Sensors >>>"
        # ">>> Time cluster >>>"
        # ">>> Object detection >>>"
        # ">>> Yaw >>>"
        # ">>> Ultrasonic Sensors Detect >>>"
        # ">>> Encoders >>>"
        # ">>> Stepper position >>>"
        # ">>> Line Sensor Cluster>>>"
        # ">>> IR Sensors >>>"
        # ">>> Time cluster >>>"
        # ">>> Object detection >>>"
        # ">>> Yaw >>>"
        # ">>> Ultrasonic Sensors Detect >>>"
        # ">>> Encoders >>>"
        # ">>> Stepper position >>>"
        # "Resets any software variables\nand/or non-critical states"
        n129 = Wait (ms)(milliseconds to wait=u32 20) -> ()  [unwired: 1 out]
        n130 = Bundle By Name(cluster=w3699, "SET TIME TO CHECK"=0.0) -> (w3698:T3)
        n131 = Bundle By Name(cluster=w3715, "Object X coordinate"=0.0, "Object Y coordinate"=0.0) -> (w3714:T11)
        n132 = Bundle By Name(cluster=w3706, "y Stepper Position"=u8 0, "z Stepper Position"=u8 0) -> (w3705:T7)
        n133 = Bundle By Name(cluster=w3693, "Left IR Sensor"=w3690, "Arm IR Sensor"=w3690) -> (w3692:T5)
        n134 = Bundle By Name(cluster=w3711, "xDistance"=0.0, "yDistance"=0.0, "wDistance"=0.0) -> (w3710:T8)
        n135 = Bundle By Name(cluster=w3722, "PING_A"=u8 0, "PING_B"=u8 0, "PING_C"=u8 0, "PING_D"=u8 0) -> (w3721:T9)
        n136 = Bundle By Name(cluster=w3702, "Yaw"=0.0) -> (w3701:T6)
        n137 = Bundle By Name(cluster=w3695, "S1"=w3691, "S2"=w3691, "S3"=w3691, "S4"=w3691) -> (w3694:T4)
      }
      frame "RESET ALL SENSORS" {
        w3724 = 0.0 ("SET TIME TO CHECK")
        # ">>> Line Sensor Cluster>>>"
        # ">>> IR Sensors >>>"
        # ">>> Time cluster >>>"
        # ">>> Object detection >>>"
        # ">>> Yaw >>>"
        # ">>> Ultrasonic Sensors Detect >>>"
        # ">>> Encoders >>>"
        # ">>> Stepper position >>>"
        # ">>> Line Sensor Cluster>>>"
        # ">>> IR Sensors >>>"
        # ">>> Time cluster >>>"
        # ">>> Object detection >>>"
        # ">>> Yaw >>>"
        # ">>> Ultrasonic Sensors Detect >>>"
        # ">>> Encoders >>>"
        # ">>> Stepper position >>>"
        # "Resets ALL SENSOR PARAMTERS"
        n138 = Wait (ms)(milliseconds to wait=u32 20) -> ()  [unwired: 1 out]
        n139 = Bundle By Name(cluster=w3735, "Time up flag"=FALSE, "SET TIME TO CHECK"=0.0) -> (w3734:T3)
        n140 = Bundle By Name(cluster=w3752, "Recognized Object"=FALSE, "Object X coordinate"=0.0, "Object Y coordinate"=0.0) -> (w3751:T11)
        n141 = Bundle By Name(cluster=w3742, "y Stepper Position"=u8 0, "z Stepper Position"=u8 0) -> (w3741:T7)
        n142 = Bundle By Name(cluster=w3727, "Left IR Sensor"=w3724, "Arm IR Sensor"=w3724, "Bottom IR Sensor"=w3724) -> (w3726:T5)
        n143 = Bundle By Name(cluster=w3730, "Line Detected?"=FALSE) -> (w3729:T4)
        n144 = Bundle By Name(cluster=w3747, "xDistance"=0.0, "yDistance"=0.0, "wDistance"=0.0) -> (w3746:T8)
        n145 = Bundle By Name(cluster=w3759, "PING_A"=u8 0, "PING_B"=u8 0, "PING_C"=u8 0, "PING_D"=u8 0) -> (w3758:T9)
        n146 = Bundle By Name(cluster=w3738, "Yaw"=0.0) -> (w3737:T6)
      }
      frame "RESET YAW" {
        n147 = Wait (ms)(milliseconds to wait=u32 100) -> ()  [unwired: 1 out]
        n148 = call "navX reading VI.vi"("Mode"=navX_type_def."Zero Yaw") -> ()  [unwired: 2 in, 4 out]
      }
      frame "RESET ARM" {
        n149 = call "Arduino Interfacing VI.vi"("Data to Write"=I2C_MASTER_WRITE_NEW_Type_Def."Soft Reset", "AE Mode"=Arduino_Interfacing."Write to Arduino") -> ()  [unwired: 2 in, 2 out]
      }
      frame "--------CAM STATES-------" {
      }
      frame "OPEN IMAQ REF" {
        # ">>> Line Sensor Cluster>>>"
        # ">>State Logic  >>"
        # ">>> Time cluster >>>"
        # ">>> Object detection >>>"
        # ">>> Yaw >>>"
        # ">>> Ultrasonic Sensors Detect >>>"
        # ">>> Encoders >>>"
        # ">>> Stepper position >>>"
        # ">>> IR Sensors >>>"
        n150 = call "IMAQ Reference AE.vi"("IMAQ AE States"=IMAQ_Reference_AE."Initialize AE") -> ()  [unwired: 1 in, 2 out]
      }
      frame "OPEN LOG CAM" {
        n151 = call "Webcam AE.vi"("Session In"=T38 "cam0", "Camera states"=Webcam_AE."Initialize Camera") -> ("error out"=w3816:errorcluster, "Session Out"=w3815:T38)  [unwired: 1 in, 1 out]
        n152 = call "Webcam AE.vi"("error in (no error)"=w3816, "Session In"=w3815, "Camera states"=Webcam_AE."Open Camera") -> ()  [unwired: 3 out]
      }
      frame "OPEN LIFE CAM" {
        n153 = call "Webcam AE.vi"("Session In"=T38 "cam1", "Camera states"=Webcam_AE."Initialize Camera") -> ("error out"=w3832:errorcluster, "Session Out"=w3831:T38)  [unwired: 1 in, 1 out]
        n154 = call "Webcam AE.vi"("error in (no error)"=w3832, "Session In"=w3831, "Camera states"=Webcam_AE."Open Camera") -> ()  [unwired: 3 out]
      }
      frame "CAM ACQ" {
        # ">>State Logic  >>"
        # ">>> Time cluster >>>"
        # ">>> Yaw >>>"
        # ">>> Stepper position >>>"
        # ">>> Encoders >>>"
        # ">>> Object detection >>>"
        # ">>> Ultrasonic Sensors Detect >>>"
        n155 = call "Webcam AE.vi"("Camera states"=Webcam_AE."Continuous Acquisition") -> ()  [unwired: 2 in, 3 out]
      }
      frame "CAM CLOSE" {
        # ">>> Box Colour Detection >>>"
        # ">>> Line Sensor Cluster>>>"
        # ">>> IR Sensors >>>"
        # ">>State Logic  >>"
        # ">>> Time cluster >>>"
        # ">>> Yaw >>>"
        # ">>> Stepper position >>>"
        # ">>> Encoders >>>"
        # ">>> Object detection >>>"
        # ">>> Ultrasonic Sensors Detect >>>"
        n156 = call "Webcam AE.vi"("Camera states"=Webcam_AE."Close Camera") -> ()  [unwired: 2 in, 3 out]
      }
      frame "PROCESS IMAGE" {
        # ">>> Line Sensor Cluster>>>"
        # ">>> IR Sensors >>>"
        # ">> Item Selection Bias >>"
        # ">> Item Selection Bias >>"
        # ">>State Logic  >>"
        # ">>> Time cluster >>>"
        # ">>> Yaw >>>"
        # ">>> Stepper position >>>"
        # ">>> Encoders >>>"
        # ">>> Object detection >>>"
        # ">>> Ultrasonic Sensors Detect >>>"
        n157 = call "Webcam AE.vi"("Camera states"=Webcam_AE."Retrieve Image") -> ("error out"=w3869:errorcluster, "Image Out"=w3872:T44)  [unwired: 2 in, 1 out]
        n158 = call "IMAQ Reference AE.vi"("IMAQ AE States"=IMAQ_Reference_AE."Get IMAQ Reference") -> ("Image Out"=w3871:T44)  [unwired: 1 in, 1 out]
        n159 = call "Object Detection SubVI v2.vi"("Error In"=w3869, "Mode"=w3870, "Image Dest"=w3871, "Image in"=w3872) -> ("Error out"=w3868:errorcluster, "Object Center Coordinates"=w3867:cluster{"x":sgl, "y":sgl}, "Object detection cluster"=w3866:T45)  [unwired: 1 out]
        n160 = Unbundle By Name(w3866) -> ("Object detected?"=w3877:bool)
        n161 = Unbundle By Name(w3867) -> ("x"=w3879:sgl, "y"=w3878:sgl)
        n162 = Bundle By Name(cluster=w3881, "Recognized Object"=w3877, "Object X coordinate"=w3879, "Object Y coordinate"=w3878) -> (w3880:T11)
      }
      frame "COLOUR PROCESSING" {
        # ">>> Box Colour Detection >>>"
        # ">>> Box Colour Detection >>>"
        # ">>> Line Sensor Cluster>>>"
        # ">>> IR Sensors >>>"
        # ">> Item Selection Bias >>"
        # ">> Item Selection Bias >>"
        # ">>State Logic  >>"
        # ">>> Time cluster >>>"
        # ">>> Yaw >>>"
        # ">>> Stepper position >>>"
        # ">>> Encoders >>>"
        # ">>> Object detection >>>"
        # ">>> Ultrasonic Sensors Detect >>>"
        n163 = call "Webcam AE.vi"("Camera states"=Webcam_AE."Retrieve Image") -> ("error out"=w3899:errorcluster, "Image Out"=w3900:T44)  [unwired: 2 in, 1 out]
        n164 = call "Box Colour Detection SubVI.vi"("Image In"=w3900, "Error In"=w3899) -> ("Colour output boolean cluster"=w3897:T46, "Error out"=w3898:errorcluster)  [unwired: 1 out]
        n165 = Unbundle By Name(w3897) -> ("Red"=w3895:bool, "Black"=w3894:bool, "Blue"=w3893:bool, "Yellow"=w3892:bool, "Green"=w3891:bool, "No recognizable coolour"=w3890:bool)
        n166 = Bundle By Name(cluster=w3896, "Red"=w3895, "Black"=w3894, "Blue"=w3893, "Yellow"=w3892, "Green"=w3891, "Unknown"=w3890) -> (w3889:T1)
      }
      frame "DISPOSE CAM BUFFERS" {
        # ">> Item Selection Bias >>"
        # ">>> Line Sensor Cluster>>>"
        # ">>> IR Sensors >>>"
        # ">>State Logic  >>"
        # ">>> Time cluster >>>"
        # ">>> Yaw >>>"
        # ">>> Stepper position >>>"
        # ">>> Encoders >>>"
        # ">>> Object detection >>>"
        # ">>> Ultrasonic Sensors Detect >>>"
        n167 = call "Webcam AE.vi"("Camera states"=Webcam_AE."Dispose Camera Image Buffer") -> ()  [unwired: 2 in, 3 out]
      }
      frame "DISPOSE PROC BUFFERS" {
        # ">>> Box Colour Detection >>>"
        # ">>> Line Sensor Cluster>>>"
        # ">>State Logic  >>"
        # ">>> IR Sensors >>>"
        # ">>> Time cluster >>>"
        # ">>> Object detection >>>"
        # ">>> Yaw >>>"
        # ">>> Ultrasonic Sensors Detect >>>"
        # ">>> Encoders >>>"
        # ">>> Stepper position >>>"
        n168 = call "IMAQ Reference AE.vi"("IMAQ AE States"=IMAQ_Reference_AE."Dispose Processing Buffer") -> ()  [unwired: 1 in, 2 out]
      }
      frame "BOX COLOUR" {
        # ">>> Box Colour Detection >>>"
        # ">>> Line Sensor Cluster>>>"
        # ">>State Logic  >>"
        # ">>> IR Sensors >>>"
        # ">>> Time cluster >>>"
        # ">>> Object detection >>>"
        # ">>> Yaw >>>"
        # ">>> Ultrasonic Sensors Detect >>>"
        # ">>> Encoders >>>"
        # ">>> Stepper position >>>"
        n169 = call "Box Colour Detection Sequence.vi"() -> ("Colour scan time out?"=w3952:bool, "Colour output boolean cluster"=w3954:T46)  [unwired: 9 in, 1 out]
        n170 = Unbundle By Name(w3954) -> ("Red"=w3951:bool, "Black"=w3947:bool, "Blue"=w3944:bool, "Yellow"=w3943:bool, "Green"=w3940:bool, "No recognizable coolour"=w3953:bool)
        n171 = Select(t=Box_Colour_FGV_Colours."Green" ("Colour"), s=w3940, f=Box_Colour_FGV_Colours."None" ("Colour")) -> (s? t:f=w3938:T2)
        n172 = Select(t=Box_Colour_FGV_Colours."Yellow" ("Colour"), s=w3943, f=w3938) -> (s? t:f=w3937:T2)
        n173 = Select(t=Box_Colour_FGV_Colours."Blue" ("Colour"), s=w3944, f=w3937) -> (s? t:f=w3946:T2)
        n174 = Select(t=Box_Colour_FGV_Colours."Black" ("Colour"), s=w3947, f=w3946) -> (s? t:f=w3949:T2)
        n175 = Select(t=Box_Colour_FGV_Colours."Red" ("Colour"), s=w3951, f=w3949) -> (s? t:f=w3936:T2)
        n176 = Bundle By Name(cluster=w3956, "Red"=w3951, "Black"=w3947, "Blue"=w3944, "Yellow"=w3943, "Green"=w3940, "Unknown"=w3953, "Image processing done"=w3952, "Colour"=w3936) -> (w3955:T1)
      }
      frame "-----ARM ACTIONS-----" {
      }
      frame "CLOSE CLAW" {
        n177 = call "Arduino Interfacing VI.vi"("Data to Write"=I2C_MASTER_WRITE_NEW_Type_Def."Close Claw", "AE Mode"=Arduino_Interfacing."Write to Arduino") -> ()  [unwired: 2 in, 2 out]
      }
      frame "OPEN CLAW" {
        n178 = call "Arduino Interfacing VI.vi"("Data to Write"=I2C_MASTER_WRITE_NEW_Type_Def."Open Claw", "AE Mode"=Arduino_Interfacing."Write to Arduino") -> ()  [unwired: 2 in, 2 out]
      }
      frame "Z STEPPER CAM HEIGHT" {
        n179 = call "Arduino Interfacing VI.vi"("Data to Write"=I2C_MASTER_WRITE_NEW_Type_Def."zStepper 6k", "AE Mode"=Arduino_Interfacing."Write to Arduino") -> ()  [unwired: 2 in, 2 out]
      }
      frame "Z STEPPER GRAB HEIGHT" {
        # ">>State Logic  >>"
        # ">>> Time cluster >>>"
        # ">>> Yaw >>>"
        # ">>> Stepper position >>>"
        # ">>> Encoders >>>"
        # ">>> Object detection >>>"
        # ">>> Ultrasonic Sensors Detect >>>"
        n180 = call "Arduino Interfacing VI.vi"("Data to Write"=I2C_MASTER_WRITE_NEW_Type_Def."zStepper 100", "AE Mode"=Arduino_Interfacing."Write to Arduino") -> ()  [unwired: 2 in, 2 out]
      }
      frame "Z STEPPER BOX HEIGHT" {
        # ">>> IR Sensors >>>"
        # ">>> Time cluster >>>"
        # ">>> Yaw >>>"
        # ">>> Stepper position >>>"
        # ">>> Encoders >>>"
        # ">>> Object detection >>>"
        # ">>> Ultrasonic Sensors Detect >>>"
        n181 = call "Arduino Interfacing VI.vi"("Data to Write"=I2C_MASTER_WRITE_NEW_Type_Def."zStepper 5k", "AE Mode"=Arduino_Interfacing."Write to Arduino") -> ()  [unwired: 2 in, 2 out]
      }
      frame "Y STEPPER CONTROL" {
        # ">>State Logic  >>"
        # ">>> yStepper command>>>"
        # ">>> Time cluster >>>"
        # ">>> Yaw >>>"
        # ">>> Stepper position >>>"
        # ">>> Encoders >>>"
        # ">>> Object detection >>>"
        # ">>> Ultrasonic Sensors Detect >>>"
        n182 = Unbundle By Name(w4048) -> ("yStepper desired"=w4047:u8)
        n183 = call "Arduino Interfacing VI.vi"("y Stepper value"=w4047, "Data to Write"=I2C_MASTER_WRITE_NEW_Type_Def."yStepper control", "AE Mode"=Arduino_Interfacing."Write to Arduino") -> ()  [unwired: 1 in, 2 out]
      }
      frame "READ STEPPER VALUES" {
        # ">>State Logic  >>"
        # ">>> Time cluster >>>"
        # ">>> Yaw >>>"
        # ">>> Stepper position >>>"
        # ">>> Encoders >>>"
        # ">>> Object detection >>>"
        # ">>> Ultrasonic Sensors Detect >>>"
        n184 = call "Arduino Interfacing VI.vi"("AE Mode"=Arduino_Interfacing."Read From Arduino") -> ("Arduino Data"=w4066:T17)  [unwired: 3 in, 1 out]
        n185 = Unbundle By Name(w4066) -> ("y Stepper Position"=w4065:u8, "z Stepper Position"=w4064:u8)
        n186 = Bundle By Name(cluster=w4069, "y Stepper Position"=w4065, "z Stepper Position"=w4064) -> (w4068:T7)
      }
      frame " -----TIMING-----" {
        # ">>State Logic  >>"
        # ">>> Time cluster >>>"
        # ">>> Yaw >>>"
        # ">>> Stepper position >>>"
        # ">>> Encoders >>>"
        # ">>> Object detection >>>"
        # ">>> Ultrasonic Sensors Detect >>>"
      }
      frame "SET TIMER 1" {
        w4085 = 1.0 ("Time Setting")
        # ">>State Logic  >>"
        # ">>> Time cluster >>>"
        # ">>> Yaw >>>"
        # ">>> Stepper position >>>"
        # ">>> Encoders >>>"
        # ">>> Object detection >>>"
        # ">>> Ultrasonic Sensors Detect >>>"
        n187 = Wait (ms)(milliseconds to wait=u32 250) -> ()  [unwired: 1 out]
        n188 = call "Elasped Timer.vi"("Time Setting"=w4085, "Action"=Elapsed_timer_control."Initialize") -> ()  [unwired: 6 in, 4 out]
        n189 = Bundle By Name(cluster=w4094, "Time up flag"=FALSE, "SET TIME TO CHECK"=w4085) -> (w4092:T3)
      }
      frame "SET TIMER 2" {
        w4101 = 2.0 ("Time Setting")
        # ">>State Logic  >>"
        # ">>> Time cluster >>>"
        # ">>> Yaw >>>"
        # ">>> Stepper position >>>"
        # ">>> Encoders >>>"
        # ">>> Object detection >>>"
        # ">>> Ultrasonic Sensors Detect >>>"
        n190 = Wait (ms)(milliseconds to wait=u32 250) -> ()  [unwired: 1 out]
        n191 = call "Elasped Timer.vi"("Time Setting"=w4101, "Action"=Elapsed_timer_control."Initialize") -> ()  [unwired: 6 in, 4 out]
        n192 = Bundle By Name(cluster=w4110, "Time up flag"=FALSE, "SET TIME TO CHECK"=w4101) -> (w4108:T3)
      }
      frame "SET TIMER 3" {
        w4117 = 3.0 ("Time Setting")
        # ">>State Logic  >>"
        # ">>> Time cluster >>>"
        # ">>> Yaw >>>"
        # ">>> Stepper position >>>"
        # ">>> Encoders >>>"
        # ">>> Object detection >>>"
        # ">>> Ultrasonic Sensors Detect >>>"
        n193 = Wait (ms)(milliseconds to wait=u32 250) -> ()  [unwired: 1 out]
        n194 = call "Elasped Timer.vi"("Time Setting"=w4117, "Action"=Elapsed_timer_control."Initialize") -> ()  [unwired: 6 in, 4 out]
        n195 = Bundle By Name(cluster=w4126, "Time up flag"=FALSE, "SET TIME TO CHECK"=w4117) -> (w4124:T3)
      }
      frame "SET TIMER 4" {
        w4133 = 4.0 ("Time Setting")
        # ">>State Logic  >>"
        # ">>> Time cluster >>>"
        # ">>> Yaw >>>"
        # ">>> Stepper position >>>"
        # ">>> Encoders >>>"
        # ">>> Object detection >>>"
        # ">>> Ultrasonic Sensors Detect >>>"
        n196 = call "Elasped Timer.vi"("Time Setting"=w4133, "Action"=Elapsed_timer_control."Initialize") -> ()  [unwired: 6 in, 4 out]
        n197 = Wait (ms)(milliseconds to wait=u32 250) -> ()  [unwired: 1 out]
        n198 = Bundle By Name(cluster=w4142, "Time up flag"=FALSE, "SET TIME TO CHECK"=w4133) -> (w4140:T3)
      }
      frame "SET TIMER 5" {
        w4150 = 5.0 ("Time Setting")
        # ">>State Logic  >>"
        # ">>> Time cluster >>>"
        # ">>> Yaw >>>"
        # ">>> Stepper position >>>"
        # ">>> Encoders >>>"
        # ">>> Object detection >>>"
        # ">>> Ultrasonic Sensors Detect >>>"
        n199 = call "Elasped Timer.vi"("Time Setting"=w4150, "Action"=Elapsed_timer_control."Initialize") -> ("Time Out?!"=w4149:bool)  [unwired: 6 in, 3 out]
        n200 = Wait (ms)(milliseconds to wait=u32 250) -> ()  [unwired: 1 out]
        n201 = Bundle By Name(cluster=w4158, "Time up flag"=w4149, "SET TIME TO CHECK"=w4150) -> (w4157:T3)
      }
      frame "START TIMER" {
        # ">>State Logic  >>"
        # ">>> Time cluster >>>"
        # ">>> Yaw >>>"
        # ">>> Stepper position >>>"
        # ">>> Encoders >>>"
        # ">>> Object detection >>>"
        # ">>> Ultrasonic Sensors Detect >>>"
        n202 = call "Elasped Timer.vi"("Action"=Elapsed_timer_control."Start") -> ("Time Out?!"=w4169:bool)  [unwired: 7 in, 3 out]
        n203 = Bundle By Name(cluster=w4172, "Time up flag"=w4169) -> (w4171:T3)
      }
      frame "-----MISC-----" {
        # ">>> Box Colour Detection >>>"
        # ">>> Line Sensor Cluster>>>"
        # ">>> IR Sensors >>>"
        # ">>> Time cluster >>>"
        # ">>> Object detection >>>"
        # ">>> Yaw >>>"
        # ">>> Ultrasonic Sensors Detect >>>"
        # ">>> Encoders >>>"
        # ">>> Stepper position >>>"
      }
      frame "Task 9" {
        # ">>> Box Colour Detection >>>"
        # ">>> Line Sensor Cluster>>>"
        # ">>> IR Sensors >>>"
        # ">>> Time cluster >>>"
        # ">>> Object detection >>>"
        # ">>> Yaw >>>"
        # ">>> Ultrasonic Sensors Detect >>>"
        # ">>> Encoders >>>"
        # ">>> Stepper position >>>"
        n204 = call "Colour Processing Test Env.vi"() -> ("Colour scan time out?"=w4198:bool, "Colour output boolean cluster"=w4196:T46)  [unwired: 10 in]
        n205 = Unbundle By Name(w4196) -> ("Red"=w4190:bool, "Black"=w4191:bool, "Blue"=w4192:bool, "Yellow"=w4193:bool, "Green"=w4194:bool, "No recognizable coolour"=w4195:bool)
        n206 = Bundle By Name(cluster=w4200, "Red"=w4190, "Black"=w4191, "Blue"=w4192, "Yellow"=w4193, "Green"=w4194, "Unknown"=w4195, "Image processing done"=w4198) -> (w4199:T1)
      }
    }
    "State Logic" <- w256
    "Image Processing Error" <- w223
    n207 = local read "TASK ENABLE"() -> (w250:bool)
    n208 = Not(x=w250) -> (.not. x?=w249:bool)
    n209 = case shown="True" w257 {
      tunnel: w214 -> [w288 w342]
      tunnel: w264 -> [w284 w344]
      tunnel: [w288 w342] -> w269
      tunnel: [w284 w345] -> w268
      tunnel: w265 -> [_ w340]
      tunnel: w267 -> [_ w341]
      tunnel: w262 -> [w287 w347]
      tunnel: [w287 w347] -> w261
      tunnel: "STOP TASK" -> [_ w330]
      tunnel: w256 -> [w286 w346]
      tunnel: [w286 w343] -> w255
      tunnel: w252 -> [w285 w336]
      tunnel: [w285 w336] -> w251
      tunnel: w249 -> [_ w331]
      tunnel: [w283 w328] -> w248
      tunnel: w247 -> [w283 w327]
      tunnel: w245 -> [w282 w324]
      tunnel: [w282 w324] -> w244
      tunnel: w242 -> [w281 w320]
      tunnel: [w281 w320] -> w241
      tunnel: w239 -> [w280 w318]
      tunnel: [w280 w318] -> w238
      tunnel: w236 -> [w279 w316]
      tunnel: [w279 w316] -> w235
      tunnel: w234 -> [w278 w315]
      tunnel: [w278 w314] -> w233
      tunnel: [_ w312] -> w232
      tunnel: w230 -> [w277 w310]
      tunnel: [w277 w310] -> w229
      tunnel: w228 -> [w276 w309]
      tunnel: [w276 w308] -> w227
      tunnel: w225 -> [w275 w305]
      tunnel: [w275 w305] -> w224
      tunnel: [w274 w304] -> w222
      tunnel: w220 -> [w274 w303]
      tunnel: [_ w301] -> w219
      tunnel: [_ w300] -> w218
      tunnel: [_ w299] -> w217
      tunnel: w215 -> [w273 w298]
      tunnel: [w273 w298] -> w213
      tunnel: [_ w289] -> w212
      frame False {
        # ">>> Box Colour Detection >>>"
        # ">>> Line Sensor Cluster>>>"
        # ">> Item Selection Bias >>"
        # ">>State Logic Queue Reference >>"
        # ">>Action states Queue Reference >>"
        # ">>True Stop Next State >>"
        # ">>State Logic  >>"
        # ">>> IR Sensors >>>"
        # ">>> Line Sensor Cluster>>>"
        # ">>> Line Sensor Cluster>>>"
        # ">>> Motor control cluster >>>"
        # ">>> yStepper command>>>"
        # ">>> Motor control cluster >>>"
        # ">>> yStepper command>>>"
        # ">>> Motor control cluster >>>"
        # ">>> IR Sensors >>>"
        # ">>> IR Sensors >>>"
        # ">>> yStepper command>>>"
        # ">>> Time cluster >>>"
        # ">>> Yaw >>>"
        # ">>> Stepper position >>>"
        # ">>> Encoders >>>"
        # ">>> Object detection >>>"
        # ">>> Ultrasonic Sensors Detect >>>"
        # ">>> Time cluster >>>"
        # ">>> Yaw >>>"
        # ">>> Stepper position >>>"
        # ">>> Encoders >>>"
        # ">>> Object detection >>>"
        # ">>> Ultrasonic Sensors Detect >>>"
      }
      frame True {
        # ">>> Box colour cluster >>>"
        # ">>State Logic Queue Reference >>"
        # ">>> Box Colour Detection >>>"
        # ">> Item Selection Bias >>"
        # ">>> IR Sensors >>>"
        # ">>> Line Sensor Cluster>>>"
        # ">>> Line Sensor Cluster>>>"
        # ">>> Motor control cluster >>>"
        # ">>> yStepper command>>>"
        # ">>> IR Sensors >>>"
        # ">>> Motor control cluster >>>"
        # ">>State Logic Queue Reference >>"
        # ">>Timeout>>"
        # ">>> yStepper command>>>"
        # ">>> Time cluster >>>"
        # ">>> Object detection >>>"
        # ">>> Yaw >>>"
        # ">>> Ultrasonic Sensors Detect >>>"
        # ">>> Encoders >>>"
        # ">>> Stepper position >>>"
        # ">>State Logic  >>"
        # ">>True Stop Next State >>"
        # ">>Action Queue>>"
        # ">> Manual override >>"
        # ">>> Time cluster >>>"
        # ">>> Yaw >>>"
        # ">>> Stepper position >>>"
        # ">>> Encoders >>>"
        # ">>> Object detection >>>"
        # ">>> Ultrasonic Sensors Detect >>>"
        # ">>Action Queue>>"
        # ">>State Logic Queue Reference >>"
        n210 = Or(x=w330, y=w331) -> (x .or. y?=w329:bool)
        n211 = Unbundle By Name(w298) -> ("Red"=w297:bool, "Black"=w296:bool, "Blue"=w295:bool, "Yellow"=w294:bool, "Green"=w293:bool, "Unknown"=w292:bool, "Image processing done"=w291:bool, "Colour"=w290:T2)
        n212 = Unbundle By Name(w305) -> ("Line Detected?"=w306:bool)
        n213 = Unbundle By Name(w310) -> ("Left IR Sensor"=w311:dbl, "Arm IR Sensor"=w307:dbl, "Bottom IR Sensor"=w302:dbl)
        n214 = Unbundle By Name(w316) -> ("Time up flag"=w317:bool)
        n215 = Unbundle By Name(w318) -> ("Yaw"=w319:dbl, "Compass"=w313:dbl)
        n216 = Unbundle By Name(w320) -> ("y Stepper Position"=w322:u8, "z Stepper Position"=w321:u8)
        n217 = Unbundle By Name(w336) -> ("xDistance"=w333:dbl, "yDistance"=w334:dbl, "wDistance"=w335:dbl)
        n218 = Unbundle By Name(w324) -> ("Recognized Object"=w323:bool, "Object X coordinate"=w326:dbl, "Object Y coordinate"=w325:dbl)
        n219 = Unbundle By Name(w347) -> ("PING_A"=w339:u8, "PING_B"=w338:u8, "PING_C"=w337:u8, "PING_D"=w332:u8)
        n220 = case shown="\"Task 5D: GRAB\"" w346 {
          tunnel: [w352 w364 w378 w389 w499 w516 w562 w600 w654 w696 w745 w788 w843 w891 w935 w995 w1036 w1079 w1128 w1171 w1224 w1262 w1314 w1360 w1406 w1447 w1496 w1540 w1586 w1627 w1676 w1720 w1766 w1807 w1856 w1900 w1946 w1987 w2036 w2071 w2089 w2137 w2178 w2228 w2284 w2323 w2372 w2415 w2468 w2506 w2558 w2595 w2643 w2686 w2736 w2780 w2828 w2884 w2925 w2977 w3025 w3070 w3114 w3162 w3213 w3256] -> w345
          tunnel: w344 -> [w352 w367 w379 w392 w501 w517 w563 w609 w652 w700 w746 w794 w836 w894 w942 w985 w1039 w1085 w1127 w1174 w1214 w1268 w1304 w1355 w1398 w1446 w1495 w1539 w1578 w1626 w1675 w1719 w1758 w1806 w1855 w1899 w1938 w1986 w2035 w2071 w2079 w2140 w2184 w2227 w2283 w2329 w2371 w2418 w2458 w2512 w2548 w2599 w2650 w2691 w2741 w2785 w2829 w2882 w2926 w2978 w3027 w3076 w3121 w3167 w3212 w3252]
          tunnel: [State_Type_Definitions,_for_0.26g_versions_and_later_3."Idle" ("Enum") State_Type_Definitions,_for_0.26g_versions_and_later_3."Idle" ("Enum") w374 w391 State_Type_Definitions,_for_0.26g_versions_and_later_3."Shutdown" ("Enum") w518 w564 w607 w655 w697 w744 w789 w842 w892 w937 w994 w1037 w1086 w1129 w1173 w1223 w1269 w1313 w1361 w1399 w1448 w1497 w1541 w1579 w1628 w1677 w1721 w1759 w1808 w1857 w1901 w1939 w1988 w2037 State_Type_Definitions,_for_0.26g_versions_and_later_3."Idle" ("Enum") w2088 w2138 w2185 w2229 w2285 w2330 w2373 w2417 w2467 w2513 w2557 w2596 w2644 w2687 w2737 w2781 w2827 w2885 w2924 w2976 w3026 w3069 w3116 w3168 w3214 w3255] -> w343
          tunnel: w342 -> [_ _ w377 w395 _ w522 w569 w603 w651 w701 w752 w793 w840 w895 w941 w992 w1034 w1084 w1125 w1175 w1221 w1267 w1311 w1358 w1405 w1444 w1493 w1537 w1585 w1624 w1673 w1717 w1765 w1804 w1853 w1897 w1945 w1984 w2033 _ w2086 w2135 w2183 w2225 w2281 w2328 w2369 w2419 w2465 w2511 w2555 w2603 w2649 w2694 w2744 w2788 w2837 w2881 w2927 w2971 w3028 w3075 w3120 w3166 w3211 w3261]
          tunnel: w341 -> [_ _ _ w394 _ w521 w568 w602 w650 w702 w751 w792 w839 w888 w940 w991 w1033 w1083 w1124 w1176 w1220 w1266 w1310 w1357 w1403 w1443 w1492 w1536 w1583 w1623 w1672 w1716 w1763 w1803 w1852 w1896 w1943 w1983 w2032 _ w2085 w2134 w2182 w2224 w2280 w2327 w2368 w2420 w2464 w2510 w2554 w2598 w2648 w2693 w2743 w2787 w2835 w2880 w2928 w2972 w3029 w3074 w3119 w3165 w3210 w3260]
          tunnel: w340 -> [_ _ w376 w390 _ w520 w567 w601 w649 w703 w750 w791 w838 w887 w939 w993 w1035 w1082 w1123 w1177 w1222 w1265 w1312 w1356 w1404 w1442 w1491 w1535 w1584 w1622 w1671 w1715 w1764 w1802 w1851 w1895 w1944 w1982 w2031 _ w2087 w2136 w2181 w2223 w2279 w2326 w2367 w2421 w2466 w2509 w2556 w2602 w2647 w2692 w2742 w2786 w2836 w2879 w2929 w2973 w3030 w3073 w3118 w3164 w3209 w3259]
          tunnel: w329 -> [_ _ _ _ _ w507 w561 w608 w648 w704 w747 w787 w841 w893 w943 w986 w1040 w1080 w1126 w1178 w1215 w1263 w1305 w1359 w1401 w1445 w1494 w1538 w1581 w1625 w1674 w1718 w1761 w1805 w1854 w1898 w1941 w1985 w2034 _ w2080 w2141 w2179 w2226 w2282 w2324 w2370 w2422 w2459 w2507 w2549 w2601 w2642 w2690 w2740 w2784 w2831 w2878 w2930 w2974 w3031 w3072 w3117 w3163 w3208 w3258]
          tunnel: w339 -> [_ _ _ _ _ _ _ _ _ _ _ _ _ _ _ _ _ _ _ _ _ _ _ _ _ _ _ _ _ _ _ _ _ _ _ _ _ _ _ _ _ _ _ _ _ _ _ _ _ _ _ _ _ _ _ _ _ _ _ _ _ _ _ _ _ _]
          tunnel: w338 -> [_ _ _ _ _ _ _ _ w647 _ _ _ w832 w876 w933 _ _ _ _ _ _ _ _ _ _ _ _ _ _ _ _ _ _ _ _ _ _ _ _ _ _ w2127 _ _ _ _ _ _ _ _ _ _ _ _ _ _ _ _ _ _ _ _ _ _ _ _]
          tunnel: w337 -> [_ _ _ _ _ _ _ _ w646 _ _ _ w833 w877 w934 _ _ _ _ _ _ _ _ _ _ _ _ _ _ _ _ _ _ _ _ _ _ _ _ _ _ w2128 _ _ _ _ _ _ _ _ _ _ _ _ _ _ _ _ _ _ _ _ _ _ _ _]
          tunnel: w335 -> [_ _ _ _ _ _ _ _ _ _ w749 _ _ _ _ _ _ _ _ _ _ _ _ _ _ _ _ _ _ _ _ _ _ _ _ _ _ _ _ _ _ _ _ _ _ _ _ _ _ _ _ _ _ _ _ _ _ _ _ w2970 _ _ _ _ _ _]
          tunnel: w334 -> [_ _ _ _ _ w515 w560 _ _ w695 _ _ _ _ w938 _ _ _ _ _ _ _ _ _ _ _ _ _ _ _ _ _ _ _ w1844 _ _ _ w2024 _ _ _ _ _ _ _ _ _ _ _ _ _ _ _ _ _ _ _ _ _ _ _ _ _ _ _]
          tunnel: w333 -> [_ _ _ _ _ _ _ _ _ _ _ _ _ w882 _ _ _ _ _ _ _ _ _ _ _ _ w1484 _ _ _ w1664 _ _ _ _ _ _ _ _ _ _ _ _ _ w2270 _ _ _ _ _ _ _ _ _ _ _ _ w2871 _ _ _ _ _ _ _ _]
          tunnel: w332 -> [_ _ _ _ _ _ _ _ _ _ _ _ _ _ _ _ _ _ _ _ _ _ _ _ _ _ _ _ _ _ _ _ _ _ _ _ _ _ _ _ _ _ _ _ _ _ _ _ _ _ _ _ _ _ _ _ _ _ _ _ _ _ _ _ _ _]
          tunnel: [State_Type_Definitions,_for_0.26g_versions_and_later_3."Idle" ("Enum") State_Type_Definitions,_for_0.26g_versions_and_later_3."Idle" ("Enum") State_Type_Definitions,_for_0.26g_versions_and_later_3."Idle" ("Enum") State_Type_Definitions,_for_0.26g_versions_and_later_3."Idle" ("Enum") State_Type_Definitions,_for_0.26g_versions_and_later_3."Shutdown" ("Enum") w513 w558 w606 w653 w698 w741 w786 w835 w890 w936 w996 w1038 w1078 w1130 w1172 w1225 w1261 w1315 w1362 w1400 w1449 w1498 w1542 w1580 w1629 w1678 w1722 w1760 w1809 w1858 w1902 w1940 w1989 w2038 w2073 w2090 w2139 w2177 w2230 w2286 w2322 w2374 w2416 w2469 w2505 w2559 w2597 w2645 w2689 w2739 w2783 w2826 w2883 w2923 w2975 w3024 w3068 w3115 w3169 w3215 w3254] -> w328
          tunnel: w327 -> [_ _ w374 _ _ _ _ _ _ _ _ _ _ _ _ _ _ _ _ _ _ _ _ _ _ _ _ _ _ _ _ _ _ _ _ _ _ _ _ w2073 _ _ _ _ _ _ _ _ _ _ _ _ _ _ _ _ _ _ _ _ _ _ _ _ _ _]
          tunnel: w323 -> [_ _ _ _ _ _ _ _ _ _ _ _ _ _ _ _ _ _ _ _ _ _ _ _ _ w1436 _ _ _ w1616 _ _ _ w1796 _ _ _ w1976 _ _ _ _ _ w2218 _ _ _ _ _ _ _ _ _ _ _ _ _ _ _ _ _ _ _ _ _ _]
          tunnel: w326 -> [_ _ _ _ _ _ _ _ _ _ _ _ _ _ _ _ _ _ _ _ _ _ _ _ _ _ _ _ _ _ _ _ _ _ _ _ _ _ _ _ _ _ _ _ w2276 _ _ _ _ _ _ _ _ _ _ _ _ _ _ _ _ _ _ _ _ _]
          tunnel: w325 -> [_ _ _ _ _ _ _ _ _ _ _ _ _ _ _ _ _ _ _ w1167 _ _ _ _ _ _ _ _ _ _ _ _ _ _ _ _ _ _ _ _ _ _ _ _ _ _ _ w2411 _ _ _ _ _ _ _ _ _ _ _ _ _ _ _ _ _ _]
          tunnel: w322 -> [_ _ _ _ _ _ _ _ _ _ _ _ _ _ _ _ _ _ _ w1166 _ _ _ _ _ _ _ _ _ _ _ _ _ _ _ _ _ _ _ _ _ _ _ _ _ _ _ w2410 _ _ _ _ _ _ _ _ _ _ _ _ _ _ _ _ _ _]
          tunnel: w321 -> [_ _ _ _ _ _ _ w605 _ _ _ w784 _ _ _ w989 _ w1074 _ _ w1218 _ w1308 w1354 _ _ _ _ _ _ _ _ _ _ _ _ _ _ _ _ w2083 _ _ _ _ _ _ _ w2462 _ w2552 w2600 _ _ _ _ _ _ _ _ _ _ _ _ _ _]
          tunnel: w319 -> [_ _ _ _ _ _ _ _ _ _ _ _ _ _ _ _ _ _ _ _ _ _ _ _ _ _ _ _ _ _ _ _ _ _ _ _ _ _ _ _ _ _ _ _ _ _ _ _ _ _ _ _ _ _ _ _ _ _ _ _ _ _ _ _ _ _]
          tunnel: w317 -> [_ _ _ _ _ _ _ _ _ _ _ _ _ _ _ _ _ _ w1120 _ _ w1259 _ _ w1394 w1437 _ _ w1574 w1617 _ _ w1754 w1797 _ _ w1934 w1977 _ _ _ _ w2175 w2217 _ w2320 w2364 _ _ w2503 _ _ _ _ _ _ _ _ _ _ _ _ _ _ _ _]
          tunnel: w315 -> [w350 w362 w373 w387 w497 w512 w557 w604 w645 w699 w740 w785 w834 w886 w932 w984 w1031 w1077 w1121 w1169 w1213 w1260 w1303 w1352 w1397 w1440 w1489 w1533 w1577 w1620 w1669 w1713 w1757 w1800 w1849 w1893 w1937 w1980 w2029 w2074 w2078 w2132 w2176 w2221 w2277 w2321 w2365 w2413 w2457 w2504 w2547 w2594 w2646 w2688 w2738 w2782 w2834 w2877 w2932 w2980 w3033 w3080 w3123 w3171 w3217 w3266]
          tunnel: [w350 w361 w373 w387 w497 w512 w557 w604 w645 w699 w740 w785 w834 w886 w932 w984 w1031 w1077 w1121 w1168 w1213 w1260 w1303 w1352 w1397 w1440 w1489 w1533 w1577 w1620 w1669 w1713 w1757 w1800 w1849 w1893 w1937 w1980 w2029 w2074 w2078 w2132 w2176 w2221 w2277 w2321 w2365 w2412 w2457 w2504 w2547 w2594 w2646 w2688 w2738 w2782 w2834 w2877 w2932 w2980 w3033 w3080 w3123 w3171 w3217 w3266] -> w314
          tunnel: w313 -> [_ _ _ _ _ _ _ _ _ _ _ _ _ _ _ _ _ _ _ _ _ _ _ _ _ _ _ _ _ _ _ _ _ _ _ _ _ _ _ _ _ _ _ _ _ _ _ _ _ _ _ _ w2641 _ _ _ _ _ _ _ _ _ _ _ _ _]
          tunnel: [_ _ _ TRUE _ w506 w554 w597 w642 w691 w737 w780 _ _ _ _ _ _ _ _ _ _ _ w1348 _ w1437 _ _ _ w1617 _ _ _ w1797 _ _ _ w1977 _ _ _ _ _ w2217 w2265 _ _ _ _ _ _ w2591 w2636 w2683 w2727 w2777 w2821 w2870 w2918 w2968 w3015 _ _ _ w3207 w3251] -> w312
          tunnel: w311 -> [_ _ _ _ _ _ _ _ _ _ _ _ _ _ _ _ _ _ _ _ _ _ _ _ _ _ _ _ _ _ _ _ _ _ _ _ _ _ _ _ _ _ _ _ _ _ _ _ _ _ _ _ _ _ _ _ _ _ _ _ _ w3067 _ _ _ _]
          tunnel: w309 -> [w349 w359 w372 w385 w496 w511 w556 w599 w644 w693 w739 w782 w827 w875 w931 w983 w1030 w1076 w1119 w1163 w1212 w1258 w1302 w1351 w1396 w1439 w1488 w1532 w1576 w1619 w1668 w1712 w1756 w1799 w1848 w1892 w1936 w1979 w2028 w2075 w2077 w2126 w2174 w2220 w2273 w2319 w2363 w2407 w2456 w2502 w2546 w2593 w2638 w2685 w2735 w2779 w2833 w2876 w2934 w2982 w3035 w3081 w3125 w3173 w3219 w3267]
          tunnel: [w349 w358 w372 w385 w496 w511 w556 w599 w644 w693 w739 w782 w827 w875 w931 w983 w1030 w1076 w1119 w1163 w1212 w1258 w1302 w1351 w1396 w1439 w1488 w1532 w1576 w1619 w1668 w1712 w1756 w1799 w1848 w1892 w1936 w1979 w2028 w2075 w2077 w2126 w2174 w2220 w2272 w2319 w2363 w2407 w2456 w2502 w2546 w2593 w2638 w2685 w2735 w2779 w2833 w2876 w2934 w2982 w3035 w3081 w3125 w3173 w3219 w3267] -> w308
          tunnel: w307 -> [_ _ _ _ _ _ _ _ _ _ _ _ _ _ _ _ _ _ _ _ _ _ _ _ _ _ _ _ _ _ _ _ _ _ _ _ _ _ _ _ _ _ _ _ _ _ _ _ _ _ _ _ _ _ w2733 _ _ _ _ _ w3022 _ _ _ _ _]
          tunnel: w306 -> [_ _ _ _ _ w508 _ _ _ _ _ _ _ _ w929 _ _ _ _ _ _ _ _ _ _ _ _ _ _ _ _ _ _ _ _ _ _ _ _ _ _ _ _ _ _ _ _ _ _ _ _ _ _ w2683 _ w2777 _ w2872 _ _ _ _ w3113 _ w3207 _]
          tunnel: [w348 w354 w371 w384 w495 w510 w555 w598 w643 w692 w738 w781 w826 w874 w930 w982 w1029 w1075 w1118 w1162 w1211 w1257 w1301 w1350 enum16{"Ball", "Soap", "Gel", "Pipe", "None"}."Ball" ("Object recognition mode") w1438 w1487 enum16{"Ball", "Soap", "Gel", "Pipe", "None"}."Soap" ("Object recognition mode") enum16{"Ball", "Soap", "Gel", "Pipe", "None"}."Soap" ("Object recognition mode") w1618 w1667 enum16{"Ball", "Soap", "Gel", "Pipe", "None"}."Gel" ("Object recognition mode") enum16{"Ball", "Soap", "Gel", "Pipe", "None"}."Gel" ("Object recognition mode") w1798 w1847 enum16{"Ball", "Soap", "Gel", "Pipe", "None"}."Pipe" ("Object recognition mode") enum16{"Ball", "Soap", "Gel", "Pipe", "None"}."Pipe" ("Object recognition mode") w1978 w2027 w2070 w2076 w2125 w2173 w2219 w2266 w2318 w2362 w2406 w2455 w2501 w2545 w2592 w2637 w2684 w2732 w2778 w2832 w2875 w2933 w2981 w3034 w3071 w3124 w3172 w3218 w3257] -> w304
          tunnel: w303 -> [w348 w354 w371 _ w495 w510 w555 w598 w643 w692 w738 w781 w826 w874 w930 w982 w1029 w1075 w1118 w1162 w1211 w1257 w1301 w1350 _ w1438 w1487 _ _ w1618 w1667 _ _ w1798 w1847 _ _ w1978 w2027 w2070 w2076 w2125 w2173 w2219 w2266 w2318 w2362 w2406 w2455 w2501 w2545 w2592 w2637 w2684 w2732 w2778 w2832 w2875 w2933 w2981 w3034 w3071 w3124 w3172 w3218 w3257]
          tunnel: w302 -> [_ _ _ _ _ _ _ _ _ _ _ _ _ _ _ _ _ _ _ _ _ _ _ _ _ _ _ _ _ _ _ _ _ _ _ _ _ _ _ _ _ w2124 _ _ _ _ _ _ _ _ _ _ _ _ w2731 _ _ _ _ _ w3016 _ _ _ _ _]
          tunnel: [_ _ _ _ _ _ _ _ w642 _ _ _ _ _ _ _ _ _ _ _ _ _ _ _ _ _ _ _ _ _ _ _ _ _ _ _ _ _ _ _ _ _ _ _ _ _ _ _ _ _ _ _ _ _ _ _ _ _ _ _ _ _ _ _ _ _] -> w301
          tunnel: [_ _ _ _ _ _ _ _ _ _ _ _ _ _ _ _ _ _ _ _ _ _ _ _ _ _ _ _ _ _ _ _ _ _ _ _ _ _ _ _ _ _ _ _ _ _ _ _ _ _ _ _ _ _ w2729 _ _ _ _ _ w3014 _ _ _ _ _] -> w300
          tunnel: [_ _ _ _ _ _ _ _ _ _ _ _ _ _ _ _ _ _ _ _ _ _ _ _ _ _ _ _ _ _ _ _ _ _ _ _ _ _ _ _ _ _ _ _ _ _ _ _ _ _ _ _ _ _ w2728 _ _ _ _ _ w3014 _ _ _ _ _] -> w299
          tunnel: w297 -> [_ _ _ _ _ _ _ _ _ _ _ _ _ _ _ _ _ _ _ _ _ _ _ _ _ _ _ _ _ _ _ _ _ _ _ _ _ _ _ _ _ _ _ _ _ _ _ _ _ _ _ _ _ _ _ _ _ _ _ _ _ _ _ _ _ _]
          tunnel: w296 -> [_ _ _ _ _ _ _ _ _ _ _ _ _ _ _ _ _ _ _ _ _ _ _ _ _ _ _ _ _ _ _ _ _ _ _ _ _ _ _ _ _ _ _ _ _ _ _ _ _ _ _ _ _ _ _ _ _ _ _ _ _ _ _ _ _ _]
          tunnel: w295 -> [_ _ _ _ _ _ _ _ _ _ _ _ _ _ _ _ _ _ _ _ _ _ _ _ _ _ _ _ _ _ _ _ _ _ _ _ _ _ _ _ _ _ _ _ _ _ _ _ _ _ _ _ _ _ _ _ _ _ _ _ _ _ _ _ _ _]
          tunnel: w294 -> [_ _ _ _ _ _ _ _ _ _ _ _ _ _ _ _ _ _ _ _ _ _ _ _ _ _ _ _ _ _ _ _ _ _ _ _ _ _ _ _ _ _ _ _ _ _ _ _ _ _ _ _ _ _ _ _ _ _ _ _ _ _ _ _ _ _]
          tunnel: w293 -> [_ _ _ _ _ _ _ _ _ _ _ _ _ _ _ _ _ _ _ _ _ _ _ _ _ _ _ _ _ _ _ _ _ _ _ _ _ _ _ _ _ _ _ _ _ _ _ _ _ _ _ _ _ _ _ _ _ _ _ _ _ _ _ _ _ _]
          tunnel: w292 -> [_ _ _ _ _ _ _ _ _ _ _ _ _ _ _ _ _ _ _ _ _ _ _ _ _ _ _ _ _ _ _ _ _ _ _ _ _ _ _ _ _ _ _ _ _ _ _ _ _ _ _ _ _ _ _ _ _ _ _ _ _ _ _ _ _ _]
          tunnel: w291 -> [_ _ _ _ _ _ _ _ _ _ _ _ _ _ _ _ _ _ _ _ _ _ _ _ _ _ _ _ _ _ _ _ _ _ _ _ _ _ _ _ _ _ _ _ _ _ _ _ _ _ _ _ _ _ _ _ w2821 _ w2918 _ _ _ _ w3157 _ w3251]
          tunnel: w290 -> [_ _ _ _ _ _ _ _ _ _ _ _ _ _ _ _ _ _ _ _ _ _ _ _ _ _ _ _ _ _ _ _ _ _ _ _ _ _ _ _ _ _ _ _ _ _ _ _ _ _ _ _ _ _ _ _ w2824 _ w2920 _ _ _ _ w3159 _ w3253]
          tunnel: [_ _ _ _ _ _ _ _ _ _ _ _ _ _ _ _ _ _ _ _ _ _ _ _ _ _ _ _ _ _ _ _ _ _ _ _ _ _ _ _ _ _ _ _ _ _ _ _ _ _ _ _ _ _ _ _ w2822 _ w2919 _ _ _ _ _ _ _] -> w289
          frame "None" {
            # ">>> Motor control cluster >>>"
            # ">>> yStepper command>>>"
          }
          frame "Startup" {
            # ">>> yStepper command>>>"
            n221 = for {
              shift-right: [w370] -> w364
              shift-left: w367 -> [w369]
              tunnel: string[] ["INIT", "RESET ARM", "RESET FLAGS", "RESET YAW", "NAVX CALIBRATE"] -> [w368] mode=indexing
              n222 = Enqueue Element(queue=w369, element=w368) -> (queue out=w370:refnum<queue>)  [unwired: 2 in, 2 out]
            }
            n223 = Bundle By Name(cluster=w362, "yStepper desired"=u8 0) -> (w361:T20)
            n224 = Bundle By Name(cluster=w359, "ySpeed"=0.0, "xSpeed"=0.0, "wSpeed"=0.0) -> (w358:T19)
          }
          frame "True Stop" {
            # ">>Action Queue>>"
            # ">>> Motor control cluster >>>"
            # ">>> yStepper command>>>"
            n225 = Flush Queue(queue=w377, error in (no error)=w376) -> ()  [unwired: 3 out]
            n226 = for {
              shift-right: [w383] -> w378
              shift-left: w379 -> [w382]
              tunnel: string[] ["STOP", "RESET ENCODERS", "RESET YAW", "RESET ARM", "RESET ALL SENSORS", "DISPOSE CAM BUFFERS", "DISPOSE PROC BUFFERS", "CAM CLOSE", ""] -> [w381] mode=indexing
              n227 = Enqueue Element(queue=w382, element=w381) -> (queue out=w383:refnum<queue>)  [unwired: 2 in, 2 out]
            }
          }
          frame "Idle", Default {
            # ">>> Motor control cluster >>>"
            # ">>> yStepper command>>>"
            n228 = Dequeue Element(queue=w395, timeout in ms (-1)=w394, error in (no error)=w390) -> (element=w393:T10)  [unwired: 3 out]
            n229 = case shown="\"None\", Default" w393 {
              tunnel: [w398 w406 w414 w422 w430 w438 w446 w454 w462 w469 w479 w486 w489] -> w389
              tunnel: w392 -> [w399 w407 w415 w423 w431 w439 w447 w455 w463 w470 w478 w486 w490]
              tunnel: [State_Type_Definitions,_for_0.26g_versions_and_later_3."Task 1A" ("Enum") State_Type_Definitions,_for_0.26g_versions_and_later_3."Task 2:Raise Arm" ("Enum") State_Type_Definitions,_for_0.26g_versions_and_later_3."Task 3" ("Enum") State_Type_Definitions,_for_0.26g_versions_and_later_3."Task 4_A" ("Enum") State_Type_Definitions,_for_0.26g_versions_and_later_3."Task 5A: RAISING ARM" ("Enum") State_Type_Definitions,_for_0.26g_versions_and_later_3."Task 6A: RAISE ARM" ("Enum") State_Type_Definitions,_for_0.26g_versions_and_later_3."Task 8A: RAISE ARM" ("Enum") State_Type_Definitions,_for_0.26g_versions_and_later_3."Task 8A: RAISE ARM" ("Enum") State_Type_Definitions,_for_0.26g_versions_and_later_3."Task 8A: RAISE ARM" ("Enum") State_Type_Definitions,_for_0.26g_versions_and_later_3."Task 8A: RAISE ARM" ("Enum") State_Type_Definitions,_for_0.26g_versions_and_later_3."Task 9A: Raise Arm" ("Enum") State_Type_Definitions,_for_0.26g_versions_and_later_3."Idle" ("Enum") State_Type_Definitions,_for_0.26g_versions_and_later_3."Shutdown" ("Enum")] -> w391
              tunnel: [enum16{"Ball", "Soap", "Gel", "Pipe", "None"}."None" ("Object recognition mode") enum16{"Ball", "Soap", "Gel", "Pipe", "None"}."None" ("Object recognition mode") enum16{"Ball", "Soap", "Gel", "Pipe", "None"}."None" ("Object recognition mode") enum16{"Ball", "Soap", "Gel", "Pipe", "None"}."None" ("Object recognition mode") enum16{"Ball", "Soap", "Gel", "Pipe", "None"}."None" ("Object recognition mode") enum16{"Ball", "Soap", "Gel", "Pipe", "None"}."None" ("Object recognition mode") enum16{"Ball", "Soap", "Gel", "Pipe", "None"}."Ball" ("Object recognition mode") enum16{"Ball", "Soap", "Gel", "Pipe", "None"}."Gel" ("Object recognition mode") enum16{"Ball", "Soap", "Gel", "Pipe", "None"}."Pipe" ("Object recognition mode") enum16{"Ball", "Soap", "Gel", "Pipe", "None"}."Soap" ("Object recognition mode") enum16{"Ball", "Soap", "Gel", "Pipe", "None"}."None" ("Object recognition mode") enum16{"Ball", "Soap", "Gel", "Pipe", "None"}."None" ("Object recognition mode") enum16{"Ball", "Soap", "Gel", "Pipe", "None"}."None" ("Object recognition mode")] -> w384
              frame "Start Task 1" {
                n230 = for {
                  shift-right: [w403] -> w398
                  shift-left: w399 -> [w402]
                  tunnel: string[] ["RESET ENCODERS", "RESET YAW", "FORWARD", "READ ENCODERS"] -> [w401] mode=indexing
                  n231 = Enqueue Element(queue=w402, element=w401) -> (queue out=w403:refnum<queue>)  [unwired: 2 in, 2 out]
                }
              }
              frame "Start Task 2" {
                n232 = for {
                  shift-right: [w411] -> w406
                  shift-left: w407 -> [w410]
                  tunnel: string[] ["RESET ENCODERS", "RESET YAW", "READ ULTRASONIC", "ARDUINO - ULTRASONIC"] -> [w409] mode=indexing
                  n233 = Enqueue Element(queue=w410, element=w409) -> (queue out=w411:refnum<queue>)  [unwired: 2 in, 2 out]
                }
              }
              frame "Start Task 3" {
                n234 = for {
                  shift-right: [w419] -> w414
                  shift-left: w415 -> [w418]
                  tunnel: string[] ["RESET ENCODERS", "READ ENCODERS", "R-ACW"] -> [w417] mode=indexing
                  n235 = Enqueue Element(queue=w418, element=w417) -> (queue out=w419:refnum<queue>)  [unwired: 2 in, 2 out]
                }
              }
              frame "Start Task 4" {
                n236 = for {
                  shift-right: [w427] -> w422
                  shift-left: w423 -> [w426]
                  tunnel: string[] ["RESET YAW", "RESET ENCODERS", "RESET ARM", "RESET FLAGS", "", ""] -> [w425] mode=indexing
                  n237 = Enqueue Element(queue=w426, element=w425) -> (queue out=w427:refnum<queue>)  [unwired: 2 in, 2 out]
                }
              }
              frame "Start Task 5" {
                n238 = for {
                  shift-right: [w435] -> w430
                  shift-left: w431 -> [w434]
                  tunnel: string[] ["RESET YAW", "RESET ENCODERS", "RESET ARM", "RESET ALL SENSORS", "", ""] -> [w433] mode=indexing
                  n239 = Enqueue Element(queue=w434, element=w433) -> (queue out=w435:refnum<queue>)  [unwired: 2 in, 2 out]
                }
              }
              frame "Start Task 6" {
                n240 = for {
                  shift-right: [w443] -> w438
                  shift-left: w439 -> [w442]
                  tunnel: string[] ["OPEN LOG CAM ", "", "", "", "", ""] -> [w441] mode=indexing
                  n241 = Enqueue Element(queue=w442, element=w441) -> (queue out=w443:refnum<queue>)  [unwired: 2 in, 2 out]
                }
              }
              frame "Start Task 8 - BALL" {
                n242 = for {
                  shift-right: [w451] -> w446
                  shift-left: w447 -> [w450]
                  tunnel: string[] ["RESET YAW", "RESET ENCODERS", "RESET ARM", "RESET FLAGS"] -> [w449] mode=indexing
                  n243 = Enqueue Element(queue=w450, element=w449) -> (queue out=w451:refnum<queue>)  [unwired: 2 in, 2 out]
                }
              }
              frame "Start Task 8 - Gel" {
                n244 = for {
                  shift-right: [w459] -> w454
                  shift-left: w455 -> [w458]
                  tunnel: string[] ["RESET YAW", "RESET ENCODERS", "RESET ARM", "RESET FLAGS"] -> [w457] mode=indexing
                  n245 = Enqueue Element(queue=w458, element=w457) -> (queue out=w459:refnum<queue>)  [unwired: 2 in, 2 out]
                }
              }
              frame "Start Task 8 - Pipe" {
                n246 = for {
                  shift-right: [w467] -> w462
                  shift-left: w463 -> [w466]
                  tunnel: string[] ["RESET YAW", "RESET ENCODERS", "RESET ARM", "RESET FLAGS"] -> [w465] mode=indexing
                  n247 = Enqueue Element(queue=w466, element=w465) -> (queue out=w467:refnum<queue>)  [unwired: 2 in, 2 out]
                }
              }
              frame "Start Task 8 - Soap" {
                n248 = for {
                  shift-right: [w475] -> w469
                  shift-left: w470 -> [w474]
                  tunnel: string[] ["RESET YAW", "RESET ENCODERS", "RESET ARM", "RESET FLAGS"] -> [w473] mode=indexing
                  n249 = Enqueue Element(queue=w474, element=w473) -> (queue out=w475:refnum<queue>)  [unwired: 2 in, 2 out]
                }
              }
              frame "Start Task 9" {
                n250 = for {
                  shift-right: [w483] -> w479
                  shift-left: w478 -> [w482]
                  tunnel: string[] ["Z STEPPER BOX HEIGHT", "READ STEPPER VALUES", "", ""] -> [w481] mode=indexing
                  n251 = Enqueue Element(queue=w482, element=w481) -> (queue out=w483:refnum<queue>)  [unwired: 2 in, 2 out]
                }
              }
              frame "None", Default {
              }
              frame "Exit" {
                n252 = for {
                  shift-right: [w494] -> w489
                  shift-left: w490 -> [w493]
                  tunnel: string[] ["STOP", "RESET ENCODERS", "RESET YAW", "EXIT"] -> [w492] mode=indexing
                  n253 = Enqueue Element(queue=w493, element=w492) -> (queue out=w494:refnum<queue>)  [unwired: 2 in, 2 out]
                }
              }
            }
          }
          frame "Shutdown" {
            # ">> Item Selection Bias >>"
            # ">>> yStepper command>>>"
            n254 = for {
              shift-right: [w505] -> w499
              shift-left: w501 -> [w504]
              tunnel: string[] ["INIT", "RESET ENCODERS", "RESET FLAGS", "CAM CLOSE", "DISPOSE BUFFERS", "EXIT", ""] -> [w503] mode=indexing
              n255 = Enqueue Element(queue=w504, element=w503) -> (queue out=w505:refnum<queue>)  [unwired: 2 in, 2 out]
            }
          }
          frame "Task 1A" {
            # ">>> Motor control cluster >>>"
            # ">> Line detection >>"
            # ">> Checks if 1 metre moved >>"
            # ">>> yStepper command>>>"
            # "Use 250"
            n256 = Greater?(x=w515, y=265.0) -> (0:w509:bool)
            n257 = Dequeue Element(queue=w522, timeout in ms (-1)=w521, error in (no error)=w520) -> (element=w519:T10)  [unwired: 3 out]
            n258 = And(x=w508, y=w509) -> (x .and. y?=w506:bool)
            n259 = case shown="\"Start Task 1\", Default" w519 {
              tunnel: w507 -> [w523 _]
              tunnel: [w533 State_Type_Definitions,_for_0.26g_versions_and_later_3."True Stop" ("Enum")] -> w518
              tunnel: w517 -> [w531 w548]
              tunnel: [w530 w547] -> w516
              tunnel: [State_Type_Definitions,_for_0.26g_versions_and_later_3."Idle" ("Enum") State_Type_Definitions,_for_0.26g_versions_and_later_3."Shutdown" ("Enum")] -> w513
              tunnel: w506 -> [w524 _]
              frame "Start Task 1", Default {
                n260 = Or(x=w524, y=w523) -> (x .or. y?=w525:bool)
                n261 = case shown="True" w525 {
                  tunnel: w531 -> [w536 w542]
                  tunnel: [w535 w540] -> w530
                  frame False {
                    n262 = for {
                      shift-right: [w538] -> w535
                      shift-left: w536 -> [w539]
                      tunnel: string[] ["READ ENCODERS", "READ NAVX", "FORWARD", "READ LINE SENSOR"] ("element") -> [w537] mode=indexing
                      n263 = Enqueue Element(queue=w539, element=w537) -> (queue out=w538:refnum<queue>)  [unwired: 2 in, 2 out]
                    }
                  }
                  frame True {
                    n264 = for {
                      shift-right: [w544] -> w540
                      shift-left: w542 -> [w545]
                      tunnel: string[] ["RESET YAW", "RESET ENCODERS", "STOP", ""] -> [w543] mode=indexing
                      n265 = Enqueue Element(queue=w545, element=w543) -> (queue out=w544:refnum<queue>)  [unwired: 2 in, 2 out]
                    }
                  }
                }
                n266 = Select(t=State_Type_Definitions,_for_0.26g_versions_and_later_3."True Stop" ("Enum"), s=w523, f=State_Type_Definitions,_for_0.26g_versions_and_later_3."Task 1B" ("Enum")) -> (s? t:f=w528:T18)
                n267 = Select(t=w528, s=w524, f=State_Type_Definitions,_for_0.26g_versions_and_later_3."Task 1A" ("Enum")) -> (s? t:f=w533:T18)
              }
              frame "Exit" {
                n268 = for {
                  shift-right: [w552] -> w547
                  shift-left: w548 -> [w553]
                  tunnel: string[] ["STOP", "RESET ENCODERS", "RESET YAW", ""] -> [w551] mode=indexing
                  n269 = Enqueue Element(queue=w553, element=w551) -> (queue out=w552:refnum<queue>)  [unwired: 2 in, 2 out]
                }
              }
            }
          }
          frame "Task 1B" {
            # ">>> Motor control cluster >>>"
            # ">> Line detection >>"
            # ">> Adds small distance overhead after 1M >>"
            # ">>> yStepper command>>>"
            n270 = Greater?(x=w560, y=50.0) -> (0:w554:bool)
            n271 = Dequeue Element(queue=w569, timeout in ms (-1)=w568, error in (no error)=w567) -> (element=w566:T10)  [unwired: 3 out]
            n272 = Or(x=w554, y=w561) -> (x .or. y?=w565:bool)
            n273 = case shown="\"Start Task 1\", Default" w566 {
              tunnel: w565 -> [w572 _]
              tunnel: [w576 State_Type_Definitions,_for_0.26g_versions_and_later_3."True Stop" ("Enum")] -> w564
              tunnel: w563 -> [w573 w591]
              tunnel: [w571 w590] -> w562
              tunnel: [State_Type_Definitions,_for_0.26g_versions_and_later_3."Idle" ("Enum") State_Type_Definitions,_for_0.26g_versions_and_later_3."Shutdown" ("Enum")] -> w558
              frame "Start Task 1", Default {
                n274 = case shown="True" w572 {
                  tunnel: w573 -> [w579 w585]
                  tunnel: [w578 w583] -> w571
                  frame False {
                    n275 = for {
                      shift-right: [w581] -> w578
                      shift-left: w579 -> [w582]
                      tunnel: string[] ["READ ENCODERS", "READ NAVX", "FORWARD", "READ LINE SENSOR"] ("element") -> [w580] mode=indexing
                      n276 = Enqueue Element(queue=w582, element=w580) -> (queue out=w581:refnum<queue>)  [unwired: 2 in, 2 out]
                    }
                  }
                  frame True {
                    n277 = for {
                      shift-right: [w587] -> w583
                      shift-left: w585 -> [w588]
                      tunnel: string[] ["RESET YAW", "RESET ENCODERS", "STOP", ""] -> [w586] mode=indexing
                      n278 = Enqueue Element(queue=w588, element=w586) -> (queue out=w587:refnum<queue>)  [unwired: 2 in, 2 out]
                    }
                  }
                }
                n279 = Select(t=State_Type_Definitions,_for_0.26g_versions_and_later_3."True Stop" ("Enum"), s=w572, f=State_Type_Definitions,_for_0.26g_versions_and_later_3."Task 1B" ("Enum")) -> (s? t:f=w576:T18)
              }
              frame "Exit" {
                n280 = for {
                  shift-right: [w595] -> w590
                  shift-left: w591 -> [w596]
                  tunnel: string[] ["STOP", "RESET ENCODERS", "RESET YAW", ""] -> [w594] mode=indexing
                  n281 = Enqueue Element(queue=w596, element=w594) -> (queue out=w595:refnum<queue>)  [unwired: 2 in, 2 out]
                }
              }
            }
          }
          frame "Task 2:Raise Arm" {
            # ">> Stepper height reeached >>"
            # ">>> yStepper command>>>"
            # ">> Manual override >>"
            n282 = Dequeue Element(queue=w603, timeout in ms (-1)=w602, error in (no error)=w601) -> (element=w611:T10)  [unwired: 3 out]
            n283 = Equal?(x=w605, y=u8 60) -> (x = y?=w597:bool)
            n284 = case shown="\"Start Task 1\", Default" w611 {
              tunnel: [w622 State_Type_Definitions,_for_0.26g_versions_and_later_3."True Stop" ("Enum")] -> w607
              tunnel: [w620 w637] -> w600
              tunnel: w609 -> [w619 _]
              tunnel: w608 -> [w613 _]
              tunnel: [State_Type_Definitions,_for_0.26g_versions_and_later_3."Idle" ("Enum") State_Type_Definitions,_for_0.26g_versions_and_later_3."Shutdown" ("Enum")] -> w606
              tunnel: w597 -> [w612 _]
              frame "Start Task 1", Default {
                # ">> WIill proceed to part ii if not manual override >>"
                # ">>If ENABLE or Trigger is set to true>>"
                n285 = Or(x=w612, y=w613) -> (x .or. y?=w614:bool)
                n286 = case shown="True" w612 {
                  tunnel: [w625 w631] -> w620
                  tunnel: w619 -> [w624 w630]
                  frame False {
                    n287 = for {
                      shift-right: [w627] -> w625
                      shift-left: w624 -> [w628]
                      tunnel: string[] ["Z STEPPER CAM HEIGHT", "READ STEPPER VALUES"] ("element") -> [w626] mode=indexing
                      n288 = Enqueue Element(queue=w628, element=w626) -> (queue out=w627:refnum<queue>)  [unwired: 2 in, 2 out]
                    }
                  }
                  frame True {
                    n289 = for {
                      shift-right: [w633] -> w631
                      shift-left: w630 -> [w634]
                      tunnel: string[] ["ARDUINO - ULTRASONIC", "READ ULTRASONIC", "", "", "", ""] -> [w632] mode=indexing
                      n290 = Enqueue Element(queue=w634, element=w632) -> (queue out=w633:refnum<queue>)  [unwired: 2 in, 2 out]
                    }
                  }
                }
                n291 = Select(t=State_Type_Definitions,_for_0.26g_versions_and_later_3."True Stop" ("Enum"), s=w613, f=State_Type_Definitions,_for_0.26g_versions_and_later_3."Task 2:Sensor Mode" ("Enum")) -> (s? t:f=w616:T18)
                n292 = Select(t=w616, s=w614, f=State_Type_Definitions,_for_0.26g_versions_and_later_3."Task 2:Raise Arm" ("Enum")) -> (s? t:f=w622:T18)
              }
              frame "Exit" {
                n293 = for {
                  shift-right: [w640] -> w637
                  shift-left: _ -> [w641]
                  tunnel: string[] ["STOP", "RESET ENCODERS", "RESET YAW", ""] -> [w639] mode=indexing
                  n294 = Enqueue Element(queue=w641, element=w639) -> (queue out=w640:refnum<queue>)  [unwired: 2 in, 2 out]
                }
              }
            }
          }
          frame "Task 2:Sensor Mode" {
            w658 = u8 20 ("y")
            # ">>> yStepper command>>>"
            # ">>Object detected>>"
            n295 = Dequeue Element(queue=w651, timeout in ms (-1)=w650, error in (no error)=w649) -> (element=w659:T10)  [unwired: 3 out]
            n296 = Less?(x=w647, y=w658) -> (x < y?=w657:bool)
            n297 = Less?(x=w646, y=w658) -> (x < y?=w656:bool)
            n298 = Or(x=w657, y=w656) -> (x .or. y?=w642:bool)
            n299 = case shown="\"Start Task 1\", Default" w659 {
              tunnel: w642 -> [w662 _]
              tunnel: [w669 State_Type_Definitions,_for_0.26g_versions_and_later_3."True Stop" ("Enum")] -> w655
              tunnel: w648 -> [w661 _]
              tunnel: w652 -> [w668 w685]
              tunnel: [w667 w686] -> w654
              tunnel: [State_Type_Definitions,_for_0.26g_versions_and_later_3."Idle" ("Enum") State_Type_Definitions,_for_0.26g_versions_and_later_3."Shutdown" ("Enum")] -> w653
              frame "Start Task 1", Default {
                n300 = case shown="False" w662 {
                  tunnel: w668 -> [w672 w679]
                  tunnel: [w673 w678] -> w667
                  frame False {
                    n301 = for {
                      tunnel: string[] ["READ ULTRASONIC", "STOP"] ("element") -> [w674] mode=indexing
                      shift-right: [w676] -> w673
                      shift-left: w672 -> [w675]
                      n302 = Enqueue Element(queue=w675, element=w674) -> (queue out=w676:refnum<queue>)  [unwired: 2 in, 2 out]
                    }
                  }
                  frame True {
                    n303 = for {
                      shift-right: [w681] -> w678
                      shift-left: w679 -> [w682]
                      tunnel: string[] ["RESET ENCODERS", "READ NAVX", "READ ENCODERS"] -> [w680] mode=indexing
                      n304 = Enqueue Element(queue=w682, element=w680) -> (queue out=w681:refnum<queue>)  [unwired: 2 in, 2 out]
                    }
                  }
                }
                n305 = Or(x=w662, y=w661) -> (x .or. y?=w660:bool)
                n306 = Select(t=State_Type_Definitions,_for_0.26g_versions_and_later_3."True Stop" ("Enum"), s=w661, f=State_Type_Definitions,_for_0.26g_versions_and_later_3."Task 2:Reverse Mode" ("Enum")) -> (s? t:f=w663:T18)
                n307 = Select(t=w663, s=w660, f=State_Type_Definitions,_for_0.26g_versions_and_later_3."Task 2:Sensor Mode" ("Enum")) -> (s? t:f=w669:T18)
              }
              frame "Exit" {
                n308 = for {
                  shift-right: [w689] -> w686
                  shift-left: w685 -> [w690]
                  tunnel: string[] ["STOP", "RESET ENCODERS", "RESET YAW", "ARDUINO MODE 0"] -> [w688] mode=indexing
                  n309 = Enqueue Element(queue=w690, element=w688) -> (queue out=w689:refnum<queue>)  [unwired: 2 in, 2 out]
                }
              }
            }
          }
          frame "Task 2:Reverse Mode" {
            # ">>> yStepper command>>>"
            n310 = Dequeue Element(queue=w701, timeout in ms (-1)=w702, error in (no error)=w703) -> (element=w705:T10)  [unwired: 3 out]
            n311 = Less?(x=w695, y=-30.0) -> (x < y?=w691:bool)
            n312 = case shown="\"Start Task 1\", Default" w705 {
              tunnel: [w715 State_Type_Definitions,_for_0.26g_versions_and_later_3."True Stop" ("Enum")] -> w697
              tunnel: w704 -> [w708 _]
              tunnel: w700 -> [w714 w731]
              tunnel: [w713 w732] -> w696
              tunnel: [State_Type_Definitions,_for_0.26g_versions_and_later_3."Idle" ("Enum") State_Type_Definitions,_for_0.26g_versions_and_later_3."Shutdown" ("Enum")] -> w698
              tunnel: w691 -> [w706 _]
              frame "Start Task 1", Default {
                n313 = case shown="True" w706 {
                  tunnel: w714 -> [w718 w725]
                  tunnel: [w719 w724] -> w713
                  frame False {
                    n314 = for {
                      tunnel: string[] ["READ ENCODERS", "REVERSE", "READ NAVX"] ("element") -> [w720] mode=indexing
                      shift-right: [w722] -> w719
                      shift-left: w718 -> [w721]
                      n315 = Enqueue Element(queue=w721, element=w720) -> (queue out=w722:refnum<queue>)  [unwired: 2 in, 2 out]
                    }
                  }
                  frame True {
                    n316 = for {
                      shift-right: [w727] -> w724
                      shift-left: w725 -> [w728]
                      tunnel: string[] ["STOP", "ARDUINO - ULTRASONIC", "READ ULTRASONIC", "RESET ENCODERS"] -> [w726] mode=indexing
                      n317 = Enqueue Element(queue=w728, element=w726) -> (queue out=w727:refnum<queue>)  [unwired: 2 in, 2 out]
                    }
                  }
                }
                n318 = Or(x=w706, y=w708) -> (x .or. y?=w707:bool)
                n319 = Select(t=State_Type_Definitions,_for_0.26g_versions_and_later_3."True Stop" ("Enum"), s=w708, f=State_Type_Definitions,_for_0.26g_versions_and_later_3."Task 2:Sensor Mode" ("Enum")) -> (s? t:f=w709:T18)
                n320 = Select(t=w709, s=w707, f=State_Type_Definitions,_for_0.26g_versions_and_later_3."Task 2:Reverse Mode" ("Enum")) -> (s? t:f=w715:T18)
              }
              frame "Exit" {
                n321 = for {
                  shift-right: [w735] -> w732
                  shift-left: w731 -> [w736]
                  tunnel: string[] ["STOP", "RESET ENCODERS", "RESET YAW", "ARDUINO MODE 0"] -> [w734] mode=indexing
                  n322 = Enqueue Element(queue=w736, element=w734) -> (queue out=w735:refnum<queue>)  [unwired: 2 in, 2 out]
                }
              }
            }
          }
          frame "Task 3" {
            # ">>> Motor control cluster >>>"
            # ">>> yStepper command>>>"
            n323 = Dequeue Element(queue=w752, timeout in ms (-1)=w751, error in (no error)=w750) -> (element=w742:T10)  [unwired: 3 out]
            n324 = Less?(x=w749, y=-160.0) -> (x < y?=w737:bool)
            n325 = Or(x=w737, y=w747) -> (x .or. y?=w743:bool)
            n326 = case shown="\"Start Task 1\", Default" w742 {
              tunnel: w743 -> [w755 _]
              tunnel: [w759 State_Type_Definitions,_for_0.26g_versions_and_later_3."True Stop" ("Enum")] -> w744
              tunnel: w746 -> [w756 w775]
              tunnel: [w754 w774] -> w745
              tunnel: [State_Type_Definitions,_for_0.26g_versions_and_later_3."Idle" ("Enum") State_Type_Definitions,_for_0.26g_versions_and_later_3."Shutdown" ("Enum")] -> w741
              frame "Start Task 1", Default {
                n327 = case shown="False" w755 {
                  tunnel: w756 -> [w762 w768]
                  tunnel: [w761 w766] -> w754
                  frame False {
                    n328 = for {
                      shift-right: [w764] -> w761
                      shift-left: w762 -> [w765]
                      tunnel: string[] ["READ ENCODERS", "R-CW"] ("element") -> [w763] mode=indexing
                      n329 = Enqueue Element(queue=w765, element=w763) -> (queue out=w764:refnum<queue>)  [unwired: 2 in, 2 out]
                    }
                  }
                  frame True {
                    n330 = for {
                      shift-right: [w770] -> w766
                      shift-left: w768 -> [w771]
                      tunnel: string[] ["RESET YAW", "RESET ENCODERS", "STOP", "ARDUINO MODE 0"] -> [w769] mode=indexing
                      n331 = Enqueue Element(queue=w771, element=w769) -> (queue out=w770:refnum<queue>)  [unwired: 2 in, 2 out]
                    }
                  }
                }
                n332 = Select(t=State_Type_Definitions,_for_0.26g_versions_and_later_3."True Stop" ("Enum"), s=w755, f=State_Type_Definitions,_for_0.26g_versions_and_later_3."Task 3" ("Enum")) -> (s? t:f=w759:T18)
              }
              frame "Exit" {
                n333 = for {
                  shift-right: [w778] -> w774
                  shift-left: w775 -> [w779]
                  tunnel: string[] ["STOP", "RESET ENCODERS", "RESET YAW", ""] -> [w777] mode=indexing
                  n334 = Enqueue Element(queue=w779, element=w777) -> (queue out=w778:refnum<queue>)  [unwired: 2 in, 2 out]
                }
              }
            }
          }
          frame "Task 4_A" {
            # ">> Stepper height reeached >>"
            # ">>> yStepper command>>>"
            # ">> Manual override >>"
            n335 = Dequeue Element(queue=w793, timeout in ms (-1)=w792, error in (no error)=w791) -> (element=w790:T10)  [unwired: 3 out]
            n336 = Equal?(x=w784, y=u8 60) -> (x = y?=w780:bool)
            n337 = case shown="\"Start Task 1\", Default" w790 {
              tunnel: [w805 State_Type_Definitions,_for_0.26g_versions_and_later_3."True Stop" ("Enum")] -> w789
              tunnel: [w803 w821] -> w788
              tunnel: w794 -> [w802 w818]
              tunnel: w787 -> [w796 _]
              tunnel: [State_Type_Definitions,_for_0.26g_versions_and_later_3."Idle" ("Enum") State_Type_Definitions,_for_0.26g_versions_and_later_3."Shutdown" ("Enum")] -> w786
              tunnel: w780 -> [w795 _]
              frame "Start Task 1", Default {
                # ">> WIill proceed to part ii if not manual override >>"
                # ">>If ENABLE or Trigger is set to true>>"
                n338 = Or(x=w795, y=w796) -> (x .or. y?=w797:bool)
                n339 = case shown="False" w795 {
                  tunnel: [w808 w814] -> w803
                  tunnel: w802 -> [w807 w813]
                  frame False {
                    n340 = for {
                      shift-right: [w810] -> w808
                      shift-left: w807 -> [w811]
                      tunnel: string[] ["Z STEPPER CAM HEIGHT", "READ STEPPER VALUES"] ("element") -> [w809] mode=indexing
                      n341 = Enqueue Element(queue=w811, element=w809) -> (queue out=w810:refnum<queue>)  [unwired: 2 in, 2 out]
                    }
                  }
                  frame True {
                    n342 = for {
                      shift-right: [w816] -> w814
                      shift-left: w813 -> [w817]
                      tunnel: string[] ["ARDUINO - ULTRASONIC", "READ ULTRASONIC", "FORWARD", "", "", ""] -> [w815] mode=indexing
                      n343 = Enqueue Element(queue=w817, element=w815) -> (queue out=w816:refnum<queue>)  [unwired: 2 in, 2 out]
                    }
                  }
                }
                n344 = Select(t=State_Type_Definitions,_for_0.26g_versions_and_later_3."True Stop" ("Enum"), s=w796, f=State_Type_Definitions,_for_0.26g_versions_and_later_3."Task 4_B" ("Enum")) -> (s? t:f=w799:T18)
                n345 = Select(t=w799, s=w797, f=State_Type_Definitions,_for_0.26g_versions_and_later_3."Task 4_A" ("Enum")) -> (s? t:f=w805:T18)
              }
              frame "Exit" {
                n346 = for {
                  shift-right: [w824] -> w821
                  shift-left: w818 -> [w825]
                  tunnel: string[] ["STOP", "RESET ENCODERS", "RESET YAW", ""] -> [w823] mode=indexing
                  n347 = Enqueue Element(queue=w825, element=w823) -> (queue out=w824:refnum<queue>)  [unwired: 2 in, 2 out]
                }
              }
            }
          }
          frame "Task 4_B" {
            w831 = u8 20
            # ">> Path blocked >>"
            # ">>> yStepper command>>>"
            # ">> Manual override >>"
            n348 = Dequeue Element(queue=w840, timeout in ms (-1)=w839, error in (no error)=w838) -> (element=w837:T10)  [unwired: 3 out]
            n349 = Less?(x=w833, y=w831) -> (x < y?=w828:bool)
            n350 = Less?(x=w832, y=w831) -> (x < y?=w829:bool)
            n351 = And(x=w829, y=w828) -> (x .and. y?=w830:bool)
            n352 = case shown="\"Start Task 1\", Default" w837 {
              tunnel: [w854 State_Type_Definitions,_for_0.26g_versions_and_later_3."True Stop" ("Enum")] -> w842
              tunnel: [w852 w869] -> w843
              tunnel: w836 -> [w851 _]
              tunnel: w841 -> [w845 _]
              tunnel: [State_Type_Definitions,_for_0.26g_versions_and_later_3."Idle" ("Enum") State_Type_Definitions,_for_0.26g_versions_and_later_3."Shutdown" ("Enum")] -> w835
              tunnel: w830 -> [w844 _]
              frame "Start Task 1", Default {
                # ">> Manual override forces program to true stop >>"
                # ">>If ENABLE or Trigger is set to true>>"
                n353 = Or(x=w844, y=w845) -> (x .or. y?=w850:bool)
                n354 = case shown="False" w844 {
                  tunnel: [w857 w862] -> w852
                  tunnel: w851 -> [w856 w861]
                  frame False {
                    n355 = for {
                      shift-right: [w859] -> w857
                      shift-left: w856 -> [w860]
                      tunnel: string[] ["FORWARD", "READ ULTRASONIC", "READ NAVX"] ("element") -> [w858] mode=indexing
                      n356 = Enqueue Element(queue=w860, element=w858) -> (queue out=w859:refnum<queue>)  [unwired: 2 in, 2 out]
                    }
                  }
                  frame True {
                    n357 = for {
                      shift-right: [w865] -> w862
                      shift-left: w861 -> [w866]
                      tunnel: string[] ["STOP", "RESET YAW", "RESET ENCODERS", "RESET FLAGS"] -> [w864] mode=indexing
                      n358 = Enqueue Element(queue=w866, element=w864) -> (queue out=w865:refnum<queue>)  [unwired: 2 in, 2 out]
                    }
                  }
                }
                n359 = Select(t=State_Type_Definitions,_for_0.26g_versions_and_later_3."True Stop" ("Enum"), s=w845, f=State_Type_Definitions,_for_0.26g_versions_and_later_3."Task 4_C" ("Enum")) -> (s? t:f=w847:T18)
                n360 = Select(t=w847, s=w850, f=State_Type_Definitions,_for_0.26g_versions_and_later_3."Task 4_B" ("Enum")) -> (s? t:f=w854:T18)
              }
              frame "Exit" {
                n361 = for {
                  shift-right: [w872] -> w869
                  shift-left: _ -> [w873]
                  tunnel: string[] ["STOP", "RESET ENCODERS", "RESET YAW", ""] -> [w871] mode=indexing
                  n362 = Enqueue Element(queue=w873, element=w871) -> (queue out=w872:refnum<queue>)  [unwired: 2 in, 2 out]
                }
              }
            }
          }
          frame "Task 4_C" {
            w885 = u8 20
            # ">> xDistance travelled>>"
            # ">> Path NOT blocked >>"
            # ">>> yStepper command>>>"
            # ">> Manual override >>"
            n363 = Dequeue Element(queue=w895, timeout in ms (-1)=w888, error in (no error)=w887) -> (element=w889:T10)  [unwired: 3 out]
            n364 = Greater?(x=w877, y=w885) -> (0:w883:bool)
            n365 = Greater?(x=w882, y=80.0) -> (0:w880:bool)
            n366 = Greater?(x=w876, y=w885) -> (0:w884:bool)
            n367 = And(x=w884, y=w883) -> (x .and. y?=w879:bool)
            n368 = And(x=w880, y=w879) -> (x .and. y?=w878:bool)
            n369 = case shown="\"Start Task 1\", Default" w889 {
              tunnel: [w906 State_Type_Definitions,_for_0.26g_versions_and_later_3."True Stop" ("Enum")] -> w892
              tunnel: [w904 w922] -> w891
              tunnel: w894 -> [w903 w919]
              tunnel: w893 -> [w897 _]
              tunnel: [State_Type_Definitions,_for_0.26g_versions_and_later_3."Idle" ("t") State_Type_Definitions,_for_0.26g_versions_and_later_3."Shutdown" ("Enum")] -> w890
              tunnel: w878 -> [w896 _]
              frame "Start Task 1", Default {
                # ">> Manual override forces program to true stop >>"
                # ">>If ENABLE or Trigger is set to true>>"
                n370 = Or(x=w896, y=w897) -> (x .or. y?=w902:bool)
                n371 = case shown="False" w896 {
                  tunnel: [w909 w914] -> w904
                  tunnel: w903 -> [w907 w913]
                  frame False {
                    n372 = for {
                      shift-right: [w911] -> w909
                      shift-left: w907 -> [w912]
                      tunnel: string[] ["RIGHT", "READ NAVX", "READ ENCODERS", "READ ULTRASONIC"] ("element") -> [w910] mode=indexing
                      n373 = Enqueue Element(queue=w912, element=w910) -> (queue out=w911:refnum<queue>)  [unwired: 2 in, 2 out]
                    }
                  }
                  frame True {
                    n374 = for {
                      shift-right: [w917] -> w914
                      shift-left: w913 -> [w918]
                      tunnel: string[] ["STOP", "RESET YAW", "RESET ENCODERS", "ARDUINO - ULTRASONIC"] -> [w916] mode=indexing
                      n375 = Enqueue Element(queue=w918, element=w916) -> (queue out=w917:refnum<queue>)  [unwired: 2 in, 2 out]
                    }
                  }
                }
                n376 = Select(t=State_Type_Definitions,_for_0.26g_versions_and_later_3."True Stop" ("Enum"), s=w897, f=State_Type_Definitions,_for_0.26g_versions_and_later_3."Task 4_D" ("Enum")) -> (s? t:f=w898:T18)
                n377 = Select(t=w898, s=w902, f=State_Type_Definitions,_for_0.26g_versions_and_later_3."Task 4_C" ("Enum")) -> (s? t:f=w906:T18)
              }
              frame "Exit" {
                n378 = for {
                  shift-right: [w925] -> w922
                  shift-left: w919 -> [w926]
                  tunnel: string[] ["STOP", "RESET ENCODERS", "RESET YAW", ""] -> [w924] mode=indexing
                  n379 = Enqueue Element(queue=w926, element=w924) -> (queue out=w925:refnum<queue>)  [unwired: 2 in, 2 out]
                }
              }
            }
          }
          frame "Task 4_D" {
            w949 = u8 20
            # ">>> Motor control cluster >>>"
            # ">> Line detected >>"
            # ">> yDistance travelled>>"
            # ">> Path blocked >>"
            # ">>> yStepper command>>>"
            # ">> Manual override >>"
            n380 = Less?(x=w934, y=w949) -> (x < y?=w947:bool)
            n381 = Greater?(x=w938, y=200.0) -> (0:w945:bool)
            n382 = Less?(x=w933, y=w949) -> (x < y?=w948:bool)
            n383 = And(x=w948, y=w947) -> (x .and. y?=w944:bool)
            n384 = Dequeue Element(queue=w941, timeout in ms (-1)=w940, error in (no error)=w939) -> (element=w950:T10)  [unwired: 3 out]
            n385 = Or(x=w945, y=w944) -> (x .or. y?=w928:bool)
            n386 = And(x=w929, y=w928) -> (x .and. y?=w927:bool)
            n387 = case shown="\"Start Task 1\", Default" w950 {
              tunnel: [w961 State_Type_Definitions,_for_0.26g_versions_and_later_3."True Stop" ("Enum")] -> w937
              tunnel: [w959 w977] -> w935
              tunnel: w942 -> [w958 w974]
              tunnel: w943 -> [w952 _]
              tunnel: [State_Type_Definitions,_for_0.26g_versions_and_later_3."Idle" ("t") State_Type_Definitions,_for_0.26g_versions_and_later_3."Shutdown" ("Enum")] -> w936
              tunnel: w927 -> [w951 _]
              frame "Start Task 1", Default {
                # ">> Manual override forces program to true stop >>"
                # ">>If ENABLE or Trigger is set to true>>"
                n388 = Or(x=w951, y=w952) -> (x .or. y?=w957:bool)
                n389 = case shown="False" w951 {
                  tunnel: [w964 w969] -> w959
                  tunnel: w958 -> [w962 w968]
                  frame False {
                    n390 = for {
                      shift-right: [w966] -> w964
                      shift-left: w962 -> [w967]
                      tunnel: string[] ["FORWARD", "READ NAVX", "READ ENCODERS", "READ ULTRASONIC", "READ LINE SENSOR"] ("element") -> [w965] mode=indexing
                      n391 = Enqueue Element(queue=w967, element=w965) -> (queue out=w966:refnum<queue>)  [unwired: 2 in, 2 out]
                    }
                  }
                  frame True {
                    n392 = for {
                      shift-right: [w972] -> w969
                      shift-left: w968 -> [w973]
                      tunnel: string[] ["STOP", "RESET YAW", "RESET ENCODERS", "RESET FLAGS"] -> [w971] mode=indexing
                      n393 = Enqueue Element(queue=w973, element=w971) -> (queue out=w972:refnum<queue>)  [unwired: 2 in, 2 out]
                    }
                  }
                }
                n394 = Select(t=State_Type_Definitions,_for_0.26g_versions_and_later_3."True Stop" ("Enum"), s=w952, f=State_Type_Definitions,_for_0.26g_versions_and_later_3."True Stop" ("Enum")) -> (s? t:f=w953:T18)
                n395 = Select(t=w953, s=w957, f=State_Type_Definitions,_for_0.26g_versions_and_later_3."Task 4_D" ("Enum")) -> (s? t:f=w961:T18)
              }
              frame "Exit" {
                n396 = for {
                  shift-right: [w980] -> w977
                  shift-left: w974 -> [w981]
                  tunnel: string[] ["STOP", "RESET ENCODERS", "RESET YAW", ""] -> [w979] mode=indexing
                  n397 = Enqueue Element(queue=w981, element=w979) -> (queue out=w980:refnum<queue>)  [unwired: 2 in, 2 out]
                }
              }
            }
          }
          frame "Task 5A: RAISING ARM" {
            # "Stays in Task 5_A until stepper reaches desired \nheight"
            # ">>> Motor control cluster >>>"
            # ">>> yStepper command>>>"
            # ">> Manual override >>"
            n398 = Dequeue Element(queue=w992, timeout in ms (-1)=w991, error in (no error)=w993) -> (element=w990:T10)  [unwired: 3 out]
            n399 = Equal?(x=w989, y=u8 60) -> (x = y?=w987:bool)
            n400 = case shown="\"Start Task 1\", Default" w990 {
              tunnel: [w1003 State_Type_Definitions,_for_0.26g_versions_and_later_3."True Stop" ("Enum")] -> w994
              tunnel: [w1006 w1023] -> w995
              tunnel: [State_Type_Definitions,_for_0.26g_versions_and_later_3."Idle" ("Enum") State_Type_Definitions,_for_0.26g_versions_and_later_3."Shutdown" ("Enum")] -> w996
              tunnel: w987 -> [w1002 _]
              tunnel: w986 -> [w1001 _]
              tunnel: w985 -> [w997 w1020]
              frame "Start Task 1", Default {
                # "T: Go back to idle, F: Continue with task\""
                # ">> Manual override >>"
                n401 = case shown="True" w1002 {
                  tunnel: [w1010 w1016] -> w1006
                  tunnel: w997 -> [w1008 w1014]
                  frame False {
                    n402 = for {
                      tunnel: string[] ["Z STEPPER GRAB HEIGHT", "READ STEPPER VALUES"] ("element") -> [w1011] mode=indexing
                      shift-right: [w1013] -> w1010
                      shift-left: w1008 -> [w1012]
                      n403 = Enqueue Element(queue=w1012, element=w1011) -> (queue out=w1013:refnum<queue>)  [unwired: 2 in, 2 out]
                    }
                  }
                  frame True {
                    n404 = for {
                      shift-right: [w1018] -> w1016
                      shift-left: w1014 -> [w1019]
                      tunnel: string[] ["", "", ""] -> [w1017] mode=indexing
                      n405 = Enqueue Element(queue=w1019, element=w1017) -> (queue out=w1018:refnum<queue>)  [unwired: 2 in, 2 out]
                    }
                  }
                }
                n406 = Or(x=w1002, y=w1001) -> (x .or. y?=w1004:bool)
                n407 = Select(t=State_Type_Definitions,_for_0.26g_versions_and_later_3."True Stop" ("Enum"), s=w1001, f=State_Type_Definitions,_for_0.26g_versions_and_later_3."Task 5B: STILL WAITING" ("Enum")) -> (s? t:f=w998:T18)
                n408 = Select(t=w998, s=w1004, f=State_Type_Definitions,_for_0.26g_versions_and_later_3."Task 5A: RAISING ARM" ("Enum")) -> (s? t:f=w1003:T18)
              }
              frame "Exit" {
                n409 = for {
                  shift-right: [w1026] -> w1023
                  shift-left: w1020 -> [w1027]
                  tunnel: string[] ["STOP", "RESET ENCODERS", "RESET YAW", "ARDUINO MODE 0"] -> [w1025] mode=indexing
                  n410 = Enqueue Element(queue=w1027, element=w1025) -> (queue out=w1026:refnum<queue>)  [unwired: 2 in, 2 out]
                }
              }
            }
          }
          frame "Task 5B: STILL WAITING" {
            # ">>> yStepper command>>>"
            n411 = Dequeue Element(queue=w1034, timeout in ms (-1)=w1033, error in (no error)=w1035) -> (element=w1032:T10)  [unwired: 3 out]
            n412 = local read "Rising Edge"() -> (w1028:bool)
            n413 = case shown="\"Start Task 1\", Default" w1032 {
              tunnel: [w1047 State_Type_Definitions,_for_0.26g_versions_and_later_3."True Stop" ("Enum")] -> w1037
              tunnel: [w1050 w1067] -> w1036
              tunnel: [State_Type_Definitions,_for_0.26g_versions_and_later_3."Idle" ("Enum") State_Type_Definitions,_for_0.26g_versions_and_later_3."Shutdown" ("Enum")] -> w1038
              tunnel: w1040 -> [w1046 _]
              tunnel: w1039 -> [w1042 w1064]
              tunnel: w1028 -> [w1041 _]
              frame "Start Task 1", Default {
                # "T: Go back to idle, F: Continue with task\""
                # ">> Manual override >>"
                n414 = case shown="True" w1041 {
                  tunnel: [w1054 w1060] -> w1050
                  tunnel: w1042 -> [w1052 w1058]
                  frame False {
                    n415 = for {
                      tunnel: string[] ["CLOSE CLAW", "START TIMER", ""] ("element") -> [w1055] mode=indexing
                      shift-right: [w1057] -> w1054
                      shift-left: w1052 -> [w1056]
                      n416 = Enqueue Element(queue=w1056, element=w1055) -> (queue out=w1057:refnum<queue>)  [unwired: 2 in, 2 out]
                    }
                  }
                  frame True {
                    n417 = for {
                      shift-right: [w1062] -> w1060
                      shift-left: w1058 -> [w1063]
                      tunnel: string[] ["STOP", "", "", ""] -> [w1061] mode=indexing
                      n418 = Enqueue Element(queue=w1063, element=w1061) -> (queue out=w1062:refnum<queue>)  [unwired: 2 in, 2 out]
                    }
                  }
                }
                n419 = Or(x=w1041, y=w1046) -> (x .or. y?=w1048:bool)
                n420 = Select(t=State_Type_Definitions,_for_0.26g_versions_and_later_3."True Stop" ("Enum"), s=w1046, f=State_Type_Definitions,_for_0.26g_versions_and_later_3."Task 5C: GOING DOWN" ("Enum")) -> (s? t:f=w1043:T18)
                n421 = Select(t=w1043, s=w1048, f=State_Type_Definitions,_for_0.26g_versions_and_later_3."Task 5B: STILL WAITING" ("Enum")) -> (s? t:f=w1047:T18)
              }
              frame "Exit" {
                n422 = for {
                  shift-right: [w1070] -> w1067
                  shift-left: w1064 -> [w1071]
                  tunnel: string[] ["STOP", "RESET ENCODERS", "RESET YAW", "ARDUINO MODE 0"] -> [w1069] mode=indexing
                  n423 = Enqueue Element(queue=w1071, element=w1069) -> (queue out=w1070:refnum<queue>)  [unwired: 2 in, 2 out]
                }
              }
            }
          }
          frame "Task 5C: GOING DOWN" {
            # ">>> Motor control cluster >>>"
            # ">>> yStepper command>>>"
            # ">> Manual override >>"
            n424 = Equal?(x=w1074, y=u8 1) -> (x = y?=w1072:bool)
            n425 = Dequeue Element(queue=w1084, timeout in ms (-1)=w1083, error in (no error)=w1082) -> (element=w1081:T10)  [unwired: 3 out]
            n426 = case shown="\"Start Task 1\", Default" w1081 {
              tunnel: [w1093 State_Type_Definitions,_for_0.26g_versions_and_later_3."True Stop" ("Enum")] -> w1086
              tunnel: [w1096 w1113] -> w1079
              tunnel: [State_Type_Definitions,_for_0.26g_versions_and_later_3."Idle" ("Enum") State_Type_Definitions,_for_0.26g_versions_and_later_3."Shutdown" ("Enum")] -> w1078
              tunnel: w1080 -> [w1087 _]
              tunnel: w1085 -> [w1092 w1110]
              tunnel: w1072 -> [w1091 _]
              frame "Start Task 1", Default {
                # ">> Is time up? >>"
                # "Determines if object is in range to pick up"
                # ">> Manual override >>"
                n427 = case shown="False" w1091 {
                  tunnel: [w1100 w1106] -> w1096
                  tunnel: w1092 -> [w1099 w1104]
                  frame False {
                    n428 = for {
                      tunnel: string[] ["Z STEPPER GRAB HEIGHT", "READ STEPPER VALUES", "", ""] -> [w1101] mode=indexing
                      shift-right: [w1103] -> w1100
                      shift-left: w1099 -> [w1102]
                      n429 = Enqueue Element(queue=w1102, element=w1101) -> (queue out=w1103:refnum<queue>)  [unwired: 2 in, 2 out]
                    }
                  }
                  frame True {
                    n430 = for {
                      shift-right: [w1108] -> w1106
                      shift-left: w1104 -> [w1109]
                      tunnel: string[] ["SET TIMER 5", "", ""] -> [w1107] mode=indexing
                      n431 = Enqueue Element(queue=w1109, element=w1107) -> (queue out=w1108:refnum<queue>)  [unwired: 2 in, 2 out]
                    }
                  }
                }
                n432 = Or(x=w1091, y=w1087) -> (x .or. y?=w1094:bool)
                n433 = Select(t=State_Type_Definitions,_for_0.26g_versions_and_later_3."True Stop" ("Enum"), s=w1087, f=State_Type_Definitions,_for_0.26g_versions_and_later_3."Task 5D: GRAB" ("Enum")) -> (s? t:f=w1089:T18)
                n434 = Select(t=w1089, s=w1094, f=State_Type_Definitions,_for_0.26g_versions_and_later_3."Task 5C: GOING DOWN" ("Enum")) -> (s? t:f=w1093:T18)
              }
              frame "Exit" {
                n435 = for {
                  shift-right: [w1116] -> w1113
                  shift-left: w1110 -> [w1117]
                  tunnel: string[] ["STOP", "RESET ENCODERS", "RESET YAW", "ARDUINO MODE 0"] -> [w1115] mode=indexing
                  n436 = Enqueue Element(queue=w1117, element=w1115) -> (queue out=w1116:refnum<queue>)  [unwired: 2 in, 2 out]
                }
              }
            }
          }
          frame "Task 5D: GRAB" {
            # ">>> Motor control cluster >>>"
            # ">>> yStepper command>>>"
            n437 = Dequeue Element(queue=w1125, timeout in ms (-1)=w1124, error in (no error)=w1123) -> (element=w1122:T10)  [unwired: 3 out]
            n438 = case shown="\"Start Task 1\", Default" w1122 {
              tunnel: [w1137 State_Type_Definitions,_for_0.26g_versions_and_later_3."True Stop" ("Enum")] -> w1129
              tunnel: [w1140 w1157] -> w1128
              tunnel: [State_Type_Definitions,_for_0.26g_versions_and_later_3."Idle" ("Enum") State_Type_Definitions,_for_0.26g_versions_and_later_3."Shutdown" ("Enum")] -> w1130
              tunnel: w1126 -> [w1136 _]
              tunnel: w1127 -> [w1132 w1154]
              tunnel: w1120 -> [w1131 _]
              frame "Start Task 1", Default {
                # ">> T: Breaks out of state loop; F: Stays in loop>>"
                # ">> Manual override >>"
                # ">> Checks if time is up>>"
                # "Stays in Task 5D until the object is detected"
                # "T: Go back to idle, F: Continue with task\""
                # ">> Manual override >>"
                n439 = case shown="False" w1131 {
                  tunnel: [w1144 w1150] -> w1140
                  tunnel: w1132 -> [w1142 w1148]
                  frame False {
                    n440 = for {
                      tunnel: string[] ["START TIMER", "OPEN CLAW", ""] ("element") -> [w1145] mode=indexing
                      shift-right: [w1147] -> w1144
                      shift-left: w1142 -> [w1146]
                      n441 = Enqueue Element(queue=w1146, element=w1145) -> (queue out=w1147:refnum<queue>)  [unwired: 2 in, 2 out]
                    }
                  }
                  frame True {
                    n442 = for {
                      shift-right: [w1152] -> w1150
                      shift-left: w1148 -> [w1153]
                      tunnel: string[] ["CAM CLOSE", "", ""] -> [w1151] mode=indexing
                      n443 = Enqueue Element(queue=w1153, element=w1151) -> (queue out=w1152:refnum<queue>)  [unwired: 2 in, 2 out]
                    }
                  }
                }
                n444 = Or(x=w1131, y=w1136) -> (x .or. y?=w1138:bool)
                n445 = Select(t=State_Type_Definitions,_for_0.26g_versions_and_later_3."True Stop" ("Enum"), s=w1136, f=State_Type_Definitions,_for_0.26g_versions_and_later_3."Task 5E: GOING UP" ("Enum")) -> (s? t:f=w1133:T18)
                n446 = Select(t=w1133, s=w1138, f=State_Type_Definitions,_for_0.26g_versions_and_later_3."Task 5D: GRAB" ("Enum")) -> (s? t:f=w1137:T18)
              }
              frame "Exit" {
                n447 = for {
                  shift-right: [w1160] -> w1157
                  shift-left: w1154 -> [w1161]
                  tunnel: string[] ["STOP", "RESET ENCODERS", "RESET YAW", "ARDUINO MODE 0"] -> [w1159] mode=indexing
                  n448 = Enqueue Element(queue=w1161, element=w1159) -> (queue out=w1160:refnum<queue>)  [unwired: 2 in, 2 out]
                }
              }
            }
          }
          frame "Task 5E: GOING UP" {
            # ">>> yStepper command>>>"
            n449 = Dequeue Element(queue=w1175, timeout in ms (-1)=w1176, error in (no error)=w1177) -> (element=w1179:T10)  [unwired: 3 out]
            n450 = formula code="if (pos < 100)\ny = 41;\n\nelse if (pos >= 100 && pos <= 140)\ny = 30;\n\nelse if (pos >= 141 && pos <= 170)\ny = 25;\n\nelse if (pos >= 171 &&pos <= 180) \ny = 20;\n\nelse if (pos >= 181&& pos <= 200)\ny = 15;\n\nelse if (pos >= 201 && pos <= 230)\ny = 10;\n\nelse if (pos >= 231 && pos <= 320)\ny = 8;\n\nelse if (pos > 320)\ny = 0;"("pos"=w1167) -> ("y"=w1170:dbl)
            n451 = To Unsigned Byte Integer(number=w1170) -> (unsigned 8bit integer=w1165:u8)
            n452 = Equal?(x=w1166, y=w1165) -> (x = y?=w1164:bool)
            n453 = case shown="\"Start Task 1\", Default" w1179 {
              tunnel: [w1186 State_Type_Definitions,_for_0.26g_versions_and_later_3."True Stop" ("Enum")] -> w1173
              tunnel: [w1189 w1206] -> w1171
              tunnel: [State_Type_Definitions,_for_0.26g_versions_and_later_3."Idle" ("Enum") State_Type_Definitions,_for_0.26g_versions_and_later_3."Shutdown" ("Enum")] -> w1172
              tunnel: w1178 -> [w1185 _]
              tunnel: w1174 -> [w1181 w1203]
              tunnel: w1164 -> [w1180 _]
              frame "Start Task 1", Default {
                # ">> T: Breaks out of state loop; F: Stays in loop>>"
                # ">> Manual override >>"
                # ">> Checks if time is up>>"
                # "Stays in Task 5D until the object is detected"
                # "T: Go back to idle, F: Continue with task\""
                # ">> Manual override >>"
                n454 = case shown="False" w1180 {
                  tunnel: [w1193 w1199] -> w1189
                  tunnel: w1181 -> [w1191 w1197]
                  frame False {
                    n455 = for {
                      tunnel: string[] ["READ STEPPER VALUES", "Y STEPPER CONTROL", ""] ("element") -> [w1194] mode=indexing
                      shift-right: [w1196] -> w1193
                      shift-left: w1191 -> [w1195]
                      n456 = Enqueue Element(queue=w1195, element=w1194) -> (queue out=w1196:refnum<queue>)  [unwired: 2 in, 2 out]
                    }
                  }
                  frame True {
                    n457 = for {
                      shift-right: [w1201] -> w1199
                      shift-left: w1197 -> [w1202]
                      tunnel: string[] ["CAM CLOSE", "DISPOSE BUFFERS", ""] -> [w1200] mode=indexing
                      n458 = Enqueue Element(queue=w1202, element=w1200) -> (queue out=w1201:refnum<queue>)  [unwired: 2 in, 2 out]
                    }
                  }
                }
                n459 = Or(x=w1180, y=w1185) -> (x .or. y?=w1187:bool)
                n460 = Select(t=State_Type_Definitions,_for_0.26g_versions_and_later_3."True Stop" ("Enum"), s=w1185, f=State_Type_Definitions,_for_0.26g_versions_and_later_3."Task 5F: ARM GRAB HEIGHT" ("Enum")) -> (s? t:f=w1182:T18)
                n461 = Select(t=w1182, s=w1187, f=State_Type_Definitions,_for_0.26g_versions_and_later_3."Task 5E: GOING UP" ("Enum")) -> (s? t:f=w1186:T18)
              }
              frame "Exit" {
                n462 = for {
                  shift-right: [w1209] -> w1206
                  shift-left: w1203 -> [w1210]
                  tunnel: string[] ["STOP", "RESET ENCODERS", "RESET YAW", "ARDUINO MODE 0"] -> [w1208] mode=indexing
                  n463 = Enqueue Element(queue=w1210, element=w1208) -> (queue out=w1209:refnum<queue>)  [unwired: 2 in, 2 out]
                }
              }
            }
            n464 = Bundle By Name(cluster=w1169, "yStepper desired"=w1165) -> (w1168:T20)
          }
          frame "Task 5F: ARM GRAB HEIGHT" {
            # ">>> Motor control cluster >>>"
            # ">>> yStepper command>>>"
            # ">> Manual override >>"
            n465 = Dequeue Element(queue=w1221, timeout in ms (-1)=w1220, error in (no error)=w1222) -> (element=w1219:T10)  [unwired: 3 out]
            n466 = Equal?(x=w1218, y=u8 1) -> (x = y?=w1216:bool)
            n467 = case shown="\"Start Task 1\", Default" w1219 {
              tunnel: [w1232 State_Type_Definitions,_for_0.26g_versions_and_later_3."True Stop" ("Enum")] -> w1223
              tunnel: [w1235 w1252] -> w1224
              tunnel: [State_Type_Definitions,_for_0.26g_versions_and_later_3."Idle" ("Enum") State_Type_Definitions,_for_0.26g_versions_and_later_3."Shutdown" ("Enum")] -> w1225
              tunnel: w1216 -> [w1231 _]
              tunnel: w1215 -> [w1230 _]
              tunnel: w1214 -> [w1226 w1249]
              frame "Start Task 1", Default {
                # "Stays in Task 5F until stepper reaches desired \nheight"
                # "T: Go back to idle, F: Continue with task\""
                # ">> Manual override >>"
                n468 = case shown="True" w1231 {
                  tunnel: [w1239 w1245] -> w1235
                  tunnel: w1226 -> [w1237 w1243]
                  frame False {
                    n469 = for {
                      tunnel: string[] ["Z STEPPER GRAB HEIGHT", "READ STEPPER VALUES"] ("element") -> [w1240] mode=indexing
                      shift-right: [w1242] -> w1239
                      shift-left: w1237 -> [w1241]
                      n470 = Enqueue Element(queue=w1241, element=w1240) -> (queue out=w1242:refnum<queue>)  [unwired: 2 in, 2 out]
                    }
                  }
                  frame True {
                    n471 = for {
                      shift-right: [w1247] -> w1245
                      shift-left: w1243 -> [w1248]
                      tunnel: string[] ["SET TIMER 5", "CLOSE CLAW", ""] -> [w1246] mode=indexing
                      n472 = Enqueue Element(queue=w1248, element=w1246) -> (queue out=w1247:refnum<queue>)  [unwired: 2 in, 2 out]
                    }
                  }
                }
                n473 = Or(x=w1231, y=w1230) -> (x .or. y?=w1233:bool)
                n474 = Select(t=State_Type_Definitions,_for_0.26g_versions_and_later_3."True Stop" ("Enum"), s=w1230, f=State_Type_Definitions,_for_0.26g_versions_and_later_3."Task 5G: CLOSE CLAW" ("Enum")) -> (s? t:f=w1227:T18)
                n475 = Select(t=w1227, s=w1233, f=State_Type_Definitions,_for_0.26g_versions_and_later_3."Task 5F: ARM GRAB HEIGHT" ("Enum")) -> (s? t:f=w1232:T18)
              }
              frame "Exit" {
                n476 = for {
                  shift-right: [w1255] -> w1252
                  shift-left: w1249 -> [w1256]
                  tunnel: string[] ["STOP", "RESET ENCODERS", "RESET YAW", "ARDUINO MODE 0"] -> [w1254] mode=indexing
                  n477 = Enqueue Element(queue=w1256, element=w1254) -> (queue out=w1255:refnum<queue>)  [unwired: 2 in, 2 out]
                }
              }
            }
          }
          frame "Task 5G: CLOSE CLAW" {
            # ">>> yStepper command>>>"
            # ">> Manual override >>"
            n478 = Dequeue Element(queue=w1267, timeout in ms (-1)=w1266, error in (no error)=w1265) -> (element=w1264:T10)  [unwired: 3 out]
            n479 = case shown="\"Start Task 1\", Default" w1264 {
              tunnel: [w1276 State_Type_Definitions,_for_0.26g_versions_and_later_3."True Stop" ("Enum")] -> w1269
              tunnel: [w1279 w1296] -> w1262
              tunnel: [State_Type_Definitions,_for_0.26g_versions_and_later_3."Idle" ("Enum") State_Type_Definitions,_for_0.26g_versions_and_later_3."Shutdown" ("Enum")] -> w1261
              tunnel: w1263 -> [w1270 _]
              tunnel: w1268 -> [w1275 w1293]
              tunnel: w1259 -> [w1274 _]
              frame "Start Task 1", Default {
                # ">> Is time up? >>"
                # "Determines if object is in range to pick up"
                # ">> Manual override >>"
                n480 = case shown="True" w1274 {
                  tunnel: [w1283 w1289] -> w1279
                  tunnel: w1275 -> [w1281 w1287]
                  frame False {
                    n481 = for {
                      tunnel: string[] ["CLOSE CLAW", "START TIMER"] ("element") -> [w1284] mode=indexing
                      shift-right: [w1286] -> w1283
                      shift-left: w1281 -> [w1285]
                      n482 = Enqueue Element(queue=w1285, element=w1284) -> (queue out=w1286:refnum<queue>)  [unwired: 2 in, 2 out]
                    }
                  }
                  frame True {
                    n483 = for {
                      shift-right: [w1291] -> w1289
                      shift-left: w1287 -> [w1292]
                      tunnel: string[] ["READ STEPPER VALUES", "", ""] -> [w1290] mode=indexing
                      n484 = Enqueue Element(queue=w1292, element=w1290) -> (queue out=w1291:refnum<queue>)  [unwired: 2 in, 2 out]
                    }
                  }
                }
                n485 = Or(x=w1274, y=w1270) -> (x .or. y?=w1277:bool)
                n486 = Select(t=State_Type_Definitions,_for_0.26g_versions_and_later_3."True Stop" ("Enum"), s=w1270, f=State_Type_Definitions,_for_0.26g_versions_and_later_3."Task 5H: RAISE ARM" ("Enum")) -> (s? t:f=w1272:T18)
                n487 = Select(t=w1272, s=w1277, f=State_Type_Definitions,_for_0.26g_versions_and_later_3."Task 5G: CLOSE CLAW" ("Enum")) -> (s? t:f=w1276:T18)
              }
              frame "Exit" {
                n488 = for {
                  shift-right: [w1299] -> w1296
                  shift-left: w1293 -> [w1300]
                  tunnel: string[] ["STOP", "RESET ENCODERS", "RESET YAW", "ARDUINO MODE 0"] -> [w1298] mode=indexing
                  n489 = Enqueue Element(queue=w1300, element=w1298) -> (queue out=w1299:refnum<queue>)  [unwired: 2 in, 2 out]
                }
              }
            }
          }
          frame "Task 5H: RAISE ARM" {
            # ">>> yStepper command>>>"
            # ">> Manual override >>"
            n490 = Dequeue Element(queue=w1311, timeout in ms (-1)=w1310, error in (no error)=w1312) -> (element=w1309:T10)  [unwired: 3 out]
            n491 = Equal?(x=w1308, y=u8 60) -> (x = y?=w1306:bool)
            n492 = case shown="\"Start Task 1\", Default" w1309 {
              tunnel: [w1322 State_Type_Definitions,_for_0.26g_versions_and_later_3."True Stop" ("Enum")] -> w1313
              tunnel: [w1325 w1342] -> w1314
              tunnel: [State_Type_Definitions,_for_0.26g_versions_and_later_3."Idle" ("Enum") State_Type_Definitions,_for_0.26g_versions_and_later_3."Shutdown" ("Enum")] -> w1315
              tunnel: w1306 -> [w1321 _]
              tunnel: w1305 -> [w1320 _]
              tunnel: w1304 -> [w1316 w1339]
              frame "Start Task 1", Default {
                # "Stays in Task 5_A until stepper reaches desired \nheight"
                # "T: Go back to idle, F: Continue with task\""
                # ">> Manual override >>"
                n493 = case shown="False" w1321 {
                  tunnel: [w1329 w1335] -> w1325
                  tunnel: w1316 -> [w1327 w1333]
                  frame False {
                    n494 = for {
                      tunnel: string[] ["Z STEPPER CAM HEIGHT", "READ STEPPER VALUES"] ("element") -> [w1330] mode=indexing
                      shift-right: [w1332] -> w1329
                      shift-left: w1327 -> [w1331]
                      n495 = Enqueue Element(queue=w1331, element=w1330) -> (queue out=w1332:refnum<queue>)  [unwired: 2 in, 2 out]
                    }
                  }
                  frame True {
                    n496 = for {
                      shift-right: [w1337] -> w1335
                      shift-left: w1333 -> [w1338]
                      tunnel: string[] ["ARDUINO - ULTRASONIC", "READ ULTRASONIC", ""] -> [w1336] mode=indexing
                      n497 = Enqueue Element(queue=w1338, element=w1336) -> (queue out=w1337:refnum<queue>)  [unwired: 2 in, 2 out]
                    }
                  }
                }
                n498 = Or(x=w1321, y=w1320) -> (x .or. y?=w1323:bool)
                n499 = Select(t=State_Type_Definitions,_for_0.26g_versions_and_later_3."True Stop" ("Enum"), s=w1320, f=State_Type_Definitions,_for_0.26g_versions_and_later_3."True Stop" ("Enum")) -> (s? t:f=w1317:T18)
                n500 = Select(t=w1317, s=w1323, f=State_Type_Definitions,_for_0.26g_versions_and_later_3."Task 5H: RAISE ARM" ("Enum")) -> (s? t:f=w1322:T18)
              }
              frame "Exit" {
                n501 = for {
                  shift-right: [w1345] -> w1342
                  shift-left: w1339 -> [w1346]
                  tunnel: string[] ["STOP", "RESET ENCODERS", "RESET YAW", "ARDUINO MODE 0"] -> [w1344] mode=indexing
                  n502 = Enqueue Element(queue=w1346, element=w1344) -> (queue out=w1345:refnum<queue>)  [unwired: 2 in, 2 out]
                }
              }
            }
          }
          frame "Task 6A: RAISE ARM" {
            # ">>> Motor control cluster >>>"
            # ">>> yStepper command>>>"
            n503 = Equal?(x=w1354, y=u8 60) -> (x = y?=w1348:bool)
            n504 = Dequeue Element(queue=w1358, timeout in ms (-1)=w1357, error in (no error)=w1356) -> (element=w1363:T10)  [unwired: 3 out]
            n505 = local read "Rising Edge"() -> (w1349:bool)
            n506 = And(x=w1349, y=w1348) -> (x .and. y?=w1347:bool)
            n507 = case shown="\"Start Task 1\", Default" w1363 {
              tunnel: [w1373 State_Type_Definitions,_for_0.26g_versions_and_later_3."True Stop" ("Enum")] -> w1361
              tunnel: [w1372 w1389] -> w1360
              tunnel: [State_Type_Definitions,_for_0.26g_versions_and_later_3."Idle" ("Enum") State_Type_Definitions,_for_0.26g_versions_and_later_3."Shutdown" ("Enum")] -> w1362
              tunnel: w1359 -> [w1369 _]
              tunnel: w1355 -> [w1370 _]
              tunnel: w1347 -> [w1367 _]
              frame "Start Task 1", Default {
                n508 = Or(x=w1367, y=w1369) -> (x .or. y?=w1364:bool)
                n509 = case shown="False" w1364 {
                  tunnel: [w1377 w1383] -> w1372
                  tunnel: w1370 -> [w1375 w1382]
                  frame False {
                    n510 = for {
                      tunnel: string[] ["Z STEPPER CAM HEIGHT", "READ STEPPER VALUES"] ("element") -> [w1378] mode=indexing
                      shift-right: [w1380] -> w1377
                      shift-left: w1375 -> [w1379]
                      n511 = Enqueue Element(queue=w1379, element=w1378) -> (queue out=w1380:refnum<queue>)  [unwired: 2 in, 2 out]
                    }
                  }
                  frame True {
                    n512 = for {
                      shift-right: [w1385] -> w1383
                      shift-left: w1382 -> [w1386]
                      tunnel: string[] ["OPEN LOG CAM", "SET TIMER 2", "OPEN IMAQ REF", "", ""] -> [w1384] mode=indexing
                      n513 = Enqueue Element(queue=w1386, element=w1384) -> (queue out=w1385:refnum<queue>)  [unwired: 2 in, 2 out]
                    }
                  }
                }
                n514 = Select(t=State_Type_Definitions,_for_0.26g_versions_and_later_3."Task 6B: CAM BURST" ("Enum"), s=w1367, f=State_Type_Definitions,_for_0.26g_versions_and_later_3."True Stop" ("Enum")) -> (s? t:f=w1365:T18)
                n515 = Select(t=w1365, s=w1364, f=State_Type_Definitions,_for_0.26g_versions_and_later_3."Task 6A: RAISE ARM" ("Enum")) -> (s? t:f=w1373:T18)
              }
              frame "Exit" {
                n516 = for {
                  shift-right: [w1392] -> w1389
                  shift-left: _ -> [w1393]
                  tunnel: string[] ["STOP", "RESET ENCODERS", "RESET YAW", "ARDUINO MODE 0"] -> [w1391] mode=indexing
                  n517 = Enqueue Element(queue=w1393, element=w1391) -> (queue out=w1392:refnum<queue>)  [unwired: 2 in, 2 out]
                }
              }
            }
          }
          frame "Task 6B: CAM BURST" {
            # ">> Manual override >>"
            # ">>> Motor control cluster >>>"
            # ">>> yStepper command>>>"
            n518 = Dequeue Element(queue=w1405, timeout in ms (-1)=w1403, error in (no error)=w1404) -> (element=w1402:T10)  [unwired: 3 out]
            n519 = case shown="\"Start Task 1\", Default" w1402 {
              tunnel: [w1413 State_Type_Definitions,_for_0.26g_versions_and_later_3."True Stop" ("Enum")] -> w1399
              tunnel: [w1411 w1431] -> w1406
              tunnel: [State_Type_Definitions,_for_0.26g_versions_and_later_3."Idle" ("Enum") State_Type_Definitions,_for_0.26g_versions_and_later_3."Shutdown" ("Enum")] -> w1400
              tunnel: w1401 -> [w1409 _]
              tunnel: w1398 -> [w1410 w1428]
              tunnel: w1394 -> [w1407 _]
              frame "Start Task 1", Default {
                n520 = Or(x=w1407, y=w1409) -> (x .or. y?=w1408:bool)
                n521 = case shown="True" w1408 {
                  tunnel: [w1418 w1424] -> w1411
                  tunnel: w1410 -> [w1416 w1422]
                  frame False {
                    n522 = for {
                      tunnel: string[] ["CAM ACQ", "START TIMER"] ("element") -> [w1419] mode=indexing
                      shift-right: [w1421] -> w1418
                      shift-left: w1416 -> [w1420]
                      n523 = Enqueue Element(queue=w1420, element=w1419) -> (queue out=w1421:refnum<queue>)  [unwired: 2 in, 2 out]
                    }
                  }
                  frame True {
                    n524 = for {
                      shift-right: [w1426] -> w1424
                      shift-left: w1422 -> [w1427]
                      tunnel: string[] ["CAM CLOSE", "PROCESS IMAGE", "SET TIMER 2", "RESET ENCODERS"] -> [w1425] mode=indexing
                      n525 = Enqueue Element(queue=w1427, element=w1425) -> (queue out=w1426:refnum<queue>)  [unwired: 2 in, 2 out]
                    }
                  }
                }
                n526 = Select(t=State_Type_Definitions,_for_0.26g_versions_and_later_3."Task 6C: PROCESS IMAGE" ("Enum"), s=w1408, f=State_Type_Definitions,_for_0.26g_versions_and_later_3."Task 6B: CAM BURST" ("Enum")) -> (s? t:f=w1413:T18)
              }
              frame "Exit" {
                # ">> State after true stop >>"
                # ">> Goes to true stop >>"
                n527 = for {
                  shift-right: [w1434] -> w1431
                  shift-left: w1428 -> [w1435]
                  tunnel: string[] ["STOP", "RESET ENCODERS", "RESET YAW", ""] -> [w1433] mode=indexing
                  n528 = Enqueue Element(queue=w1435, element=w1433) -> (queue out=w1434:refnum<queue>)  [unwired: 2 in, 2 out]
                }
              }
            }
          }
          frame "Task 6C: PROCESS IMAGE" {
            # "Ball > Soap > Gel > Pipe"
            # ">>> Motor control cluster >>>"
            # ">>> yStepper command>>>"
            n529 = Dequeue Element(queue=w1444, timeout in ms (-1)=w1443, error in (no error)=w1442) -> (element=w1441:T10)  [unwired: 3 out]
            n530 = case shown="\"Start Task 1\", Default" w1441 {
              tunnel: [w1460 State_Type_Definitions,_for_0.26g_versions_and_later_3."True Stop" ("Enum")] -> w1448
              tunnel: [w1462 w1479] -> w1447
              tunnel: [State_Type_Definitions,_for_0.26g_versions_and_later_3."Idle" ("Enum") State_Type_Definitions,_for_0.26g_versions_and_later_3."Shutdown" ("Enum")] -> w1449
              tunnel: w1445 -> [w1451 _]
              tunnel: w1446 -> [w1457 w1476]
              tunnel: w1437 -> [w1455 _]
              tunnel: w1436 -> [w1456 _]
              frame "Start Task 1", Default {
                # "Stays in Task 5D until the object is detected"
                n531 = Or(x=w1455, y=w1451) -> (x .or. y?=w1454:bool)
                n532 = case shown="True" w1454 {
                  tunnel: [w1466 w1472] -> w1462
                  tunnel: w1457 -> [w1464 w1470]
                  frame False {
                    n533 = for {
                      tunnel: string[] ["START TIMER", "PROCESS IMAGE", ""] ("element") -> [w1467] mode=indexing
                      shift-right: [w1469] -> w1466
                      shift-left: w1464 -> [w1468]
                      n534 = Enqueue Element(queue=w1468, element=w1467) -> (queue out=w1469:refnum<queue>)  [unwired: 2 in, 2 out]
                    }
                  }
                  frame True {
                    n535 = for {
                      shift-right: [w1474] -> w1472
                      shift-left: w1470 -> [w1475]
                      tunnel: string[] ["RESET ENCODERS", "RESET YAW", ""] -> [w1473] mode=indexing
                      n536 = Enqueue Element(queue=w1475, element=w1473) -> (queue out=w1474:refnum<queue>)  [unwired: 2 in, 2 out]
                    }
                  }
                }
                n537 = Select(t=State_Type_Definitions,_for_0.26g_versions_and_later_3."Task 6D: BALL BUSTER" ("Enum"), s=w1456, f=State_Type_Definitions,_for_0.26g_versions_and_later_3."Task 6F: CAM BURST 2" ("Enum")) -> (s? t:f=w1452:T18)
                n538 = Select(t=State_Type_Definitions,_for_0.26g_versions_and_later_3."True Stop" ("Enum"), s=w1451, f=w1452) -> (s? t:f=w1458:T18)
                n539 = Select(t=w1458, s=w1454, f=State_Type_Definitions,_for_0.26g_versions_and_later_3."Task 6C: PROCESS IMAGE" ("Enum")) -> (s? t:f=w1460:T18)
              }
              frame "Exit" {
                n540 = for {
                  shift-right: [w1482] -> w1479
                  shift-left: w1476 -> [w1483]
                  tunnel: string[] ["STOP", "RESET ENCODERS", "RESET YAW", "ARDUINO MODE 0"] -> [w1481] mode=indexing
                  n541 = Enqueue Element(queue=w1483, element=w1481) -> (queue out=w1482:refnum<queue>)  [unwired: 2 in, 2 out]
                }
              }
            }
          }
          frame "Task 6D: BALL BUSTER" {
            # "Ball > Soap > Gel > Pipe"
            # ">>> Motor control cluster >>>"
            # ">>> yStepper command>>>"
            n542 = Greater Or Equal?(x=w1484, y=20.0) -> (x >= y?=w1485:bool)
            n543 = Dequeue Element(queue=w1493, timeout in ms (-1)=w1492, error in (no error)=w1491) -> (element=w1490:T10)  [unwired: 3 out]
            n544 = case shown="\"Start Task 1\", Default" w1490 {
              tunnel: [w1506 State_Type_Definitions,_for_0.26g_versions_and_later_3."True Stop" ("Enum")] -> w1497
              tunnel: [w1508 w1525] -> w1496
              tunnel: [State_Type_Definitions,_for_0.26g_versions_and_later_3."Idle" ("Enum") State_Type_Definitions,_for_0.26g_versions_and_later_3."Shutdown" ("Enum")] -> w1498
              tunnel: w1494 -> [w1501 _]
              tunnel: w1495 -> [w1503 w1522]
              tunnel: w1485 -> [w1500 _]
              frame "Start Task 1", Default {
                # "Stays in Task 5D until the object is detected"
                n545 = Or(x=w1500, y=w1501) -> (x .or. y?=w1502:bool)
                n546 = case shown="False" w1502 {
                  tunnel: [w1512 w1518] -> w1508
                  tunnel: w1503 -> [w1510 w1516]
                  frame False {
                    n547 = for {
                      tunnel: string[] ["RIGHT", "READ NAVX", "READ ENCODERS"] ("element") -> [w1513] mode=indexing
                      shift-right: [w1515] -> w1512
                      shift-left: w1510 -> [w1514]
                      n548 = Enqueue Element(queue=w1514, element=w1513) -> (queue out=w1515:refnum<queue>)  [unwired: 2 in, 2 out]
                    }
                  }
                  frame True {
                    n549 = for {
                      shift-right: [w1520] -> w1518
                      shift-left: w1516 -> [w1521]
                      tunnel: string[] ["RESET ENCODERS", "RESET YAW", "RESET FLAGS"] -> [w1519] mode=indexing
                      n550 = Enqueue Element(queue=w1521, element=w1519) -> (queue out=w1520:refnum<queue>)  [unwired: 2 in, 2 out]
                    }
                  }
                }
                n551 = Select(t=State_Type_Definitions,_for_0.26g_versions_and_later_3."True Stop" ("Enum"), s=w1501, f=State_Type_Definitions,_for_0.26g_versions_and_later_3."Task 6E: STILL WAITING" ("Enum")) -> (s? t:f=w1504:T18)
                n552 = Select(t=w1504, s=w1502, f=State_Type_Definitions,_for_0.26g_versions_and_later_3."Task 6D: BALL BUSTER" ("Enum")) -> (s? t:f=w1506:T18)
              }
              frame "Exit" {
                n553 = for {
                  shift-right: [w1528] -> w1525
                  shift-left: w1522 -> [w1529]
                  tunnel: string[] ["STOP", "RESET ENCODERS", "RESET YAW", "ARDUINO MODE 0"] -> [w1527] mode=indexing
                  n554 = Enqueue Element(queue=w1529, element=w1527) -> (queue out=w1528:refnum<queue>)  [unwired: 2 in, 2 out]
                }
              }
            }
          }
          frame "Task 6E: STILL WAITING" {
            # "Ball > Soap > Gel > Pipe"
            # ">>> Motor control cluster >>>"
            # ">>> yStepper command>>>"
            n555 = local read "Rising Edge"() -> (w1531:bool)
            n556 = Dequeue Element(queue=w1537, timeout in ms (-1)=w1536, error in (no error)=w1535) -> (element=w1534:T10)  [unwired: 3 out]
            n557 = case shown="\"Start Task 1\", Default" w1534 {
              tunnel: [w1551 State_Type_Definitions,_for_0.26g_versions_and_later_3."True Stop" ("Enum")] -> w1541
              tunnel: [w1544 w1569] -> w1540
              tunnel: [State_Type_Definitions,_for_0.26g_versions_and_later_3."Idle" ("Enum") State_Type_Definitions,_for_0.26g_versions_and_later_3."Shutdown" ("Enum")] -> w1542
              tunnel: w1538 -> [w1548 _]
              tunnel: w1539 -> [w1545 w1566]
              tunnel: w1531 -> [w1546 _]
              frame "Start Task 1", Default {
                # "Stays in Task 5D until the object is detected"
                n558 = Or(x=w1546, y=w1548) -> (x .or. y?=w1543:bool)
                n559 = case shown="False" w1543 {
                  tunnel: [w1556 w1562] -> w1544
                  tunnel: w1545 -> [w1554 w1561]
                  frame False {
                    n560 = for {
                      tunnel: string[] ["Z STEPPER CAM HEIGHT", "READ STEPPER VALUES"] ("element") -> [w1557] mode=indexing
                      shift-right: [w1559] -> w1556
                      shift-left: w1554 -> [w1558]
                      n561 = Enqueue Element(queue=w1558, element=w1557) -> (queue out=w1559:refnum<queue>)  [unwired: 2 in, 2 out]
                    }
                  }
                  frame True {
                    n562 = for {
                      shift-right: [w1564] -> w1562
                      shift-left: w1561 -> [w1565]
                      tunnel: string[] ["OPEN LOG CAM", "SET TIMER 2", "OPEN IMAQ REF", "", ""] -> [w1563] mode=indexing
                      n563 = Enqueue Element(queue=w1565, element=w1563) -> (queue out=w1564:refnum<queue>)  [unwired: 2 in, 2 out]
                    }
                  }
                }
                n564 = Select(t=State_Type_Definitions,_for_0.26g_versions_and_later_3."True Stop" ("Enum"), s=w1548, f=State_Type_Definitions,_for_0.26g_versions_and_later_3."Task 6F: CAM BURST 2" ("Enum")) -> (s? t:f=w1549:T18)
                n565 = Select(t=w1549, s=w1543, f=State_Type_Definitions,_for_0.26g_versions_and_later_3."Task 6E: STILL WAITING" ("Enum")) -> (s? t:f=w1551:T18)
              }
              frame "Exit" {
                n566 = for {
                  shift-right: [w1572] -> w1569
                  shift-left: w1566 -> [w1573]
                  tunnel: string[] ["STOP", "RESET ENCODERS", "RESET YAW", "ARDUINO MODE 0"] -> [w1571] mode=indexing
                  n567 = Enqueue Element(queue=w1573, element=w1571) -> (queue out=w1572:refnum<queue>)  [unwired: 2 in, 2 out]
                }
              }
            }
          }
          frame "Task 6F: CAM BURST 2" {
            # ">> Manual override >>"
            # ">>> Motor control cluster >>>"
            # ">>> yStepper command>>>"
            n568 = Dequeue Element(queue=w1585, timeout in ms (-1)=w1583, error in (no error)=w1584) -> (element=w1582:T10)  [unwired: 3 out]
            n569 = case shown="\"Start Task 1\", Default" w1582 {
              tunnel: [w1593 State_Type_Definitions,_for_0.26g_versions_and_later_3."True Stop" ("Enum")] -> w1579
              tunnel: [w1591 w1611] -> w1586
              tunnel: [State_Type_Definitions,_for_0.26g_versions_and_later_3."Idle" ("Enum") State_Type_Definitions,_for_0.26g_versions_and_later_3."Shutdown" ("Enum")] -> w1580
              tunnel: w1581 -> [w1589 _]
              tunnel: w1578 -> [w1590 w1608]
              tunnel: w1574 -> [w1587 _]
              frame "Start Task 1", Default {
                n570 = Or(x=w1587, y=w1589) -> (x .or. y?=w1588:bool)
                n571 = case shown="True" w1588 {
                  tunnel: [w1598 w1604] -> w1591
                  tunnel: w1590 -> [w1596 w1602]
                  frame False {
                    n572 = for {
                      tunnel: string[] ["CAM ACQ", "START TIMER"] ("element") -> [w1599] mode=indexing
                      shift-right: [w1601] -> w1598
                      shift-left: w1596 -> [w1600]
                      n573 = Enqueue Element(queue=w1600, element=w1599) -> (queue out=w1601:refnum<queue>)  [unwired: 2 in, 2 out]
                    }
                  }
                  frame True {
                    n574 = for {
                      shift-right: [w1606] -> w1604
                      shift-left: w1602 -> [w1607]
                      tunnel: string[] ["CAM CLOSE", "PROCESS IMAGE", "SET TIMER 2", "RESET ENCODERS"] -> [w1605] mode=indexing
                      n575 = Enqueue Element(queue=w1607, element=w1605) -> (queue out=w1606:refnum<queue>)  [unwired: 2 in, 2 out]
                    }
                  }
                }
                n576 = Select(t=State_Type_Definitions,_for_0.26g_versions_and_later_3."Task 6G: PROCESS IMAGE 2" ("Enum"), s=w1588, f=State_Type_Definitions,_for_0.26g_versions_and_later_3."Task 6F: CAM BURST 2" ("Enum")) -> (s? t:f=w1593:T18)
              }
              frame "Exit" {
                # ">> State after true stop >>"
                # ">> Goes to true stop >>"
                n577 = for {
                  shift-right: [w1614] -> w1611
                  shift-left: w1608 -> [w1615]
                  tunnel: string[] ["STOP", "RESET ENCODERS", "RESET YAW", ""] -> [w1613] mode=indexing
                  n578 = Enqueue Element(queue=w1615, element=w1613) -> (queue out=w1614:refnum<queue>)  [unwired: 2 in, 2 out]
                }
              }
            }
          }
          frame "Task 6G: PROCESS IMAGE 2" {
            # "Ball > Soap > Gel > Pipe"
            # ">>> Motor control cluster >>>"
            # ">>> yStepper command>>>"
            n579 = Dequeue Element(queue=w1624, timeout in ms (-1)=w1623, error in (no error)=w1622) -> (element=w1621:T10)  [unwired: 3 out]
            n580 = case shown="\"Start Task 1\", Default" w1621 {
              tunnel: [w1640 State_Type_Definitions,_for_0.26g_versions_and_later_3."True Stop" ("Enum")] -> w1628
              tunnel: [w1642 w1659] -> w1627
              tunnel: [State_Type_Definitions,_for_0.26g_versions_and_later_3."Idle" ("Enum") State_Type_Definitions,_for_0.26g_versions_and_later_3."Shutdown" ("Enum")] -> w1629
              tunnel: w1625 -> [w1631 _]
              tunnel: w1626 -> [w1637 w1656]
              tunnel: w1617 -> [w1635 _]
              tunnel: w1616 -> [w1636 _]
              frame "Start Task 1", Default {
                # "Stays in Task 5D until the object is detected"
                n581 = Or(x=w1635, y=w1631) -> (x .or. y?=w1634:bool)
                n582 = case shown="True" w1634 {
                  tunnel: [w1646 w1652] -> w1642
                  tunnel: w1637 -> [w1644 w1650]
                  frame False {
                    n583 = for {
                      tunnel: string[] ["START TIMER", "PROCESS IMAGE", ""] ("element") -> [w1647] mode=indexing
                      shift-right: [w1649] -> w1646
                      shift-left: w1644 -> [w1648]
                      n584 = Enqueue Element(queue=w1648, element=w1647) -> (queue out=w1649:refnum<queue>)  [unwired: 2 in, 2 out]
                    }
                  }
                  frame True {
                    n585 = for {
                      shift-right: [w1654] -> w1652
                      shift-left: w1650 -> [w1655]
                      tunnel: string[] ["RESET ENCODERS", "RESET YAW", ""] -> [w1653] mode=indexing
                      n586 = Enqueue Element(queue=w1655, element=w1653) -> (queue out=w1654:refnum<queue>)  [unwired: 2 in, 2 out]
                    }
                  }
                }
                n587 = Select(t=State_Type_Definitions,_for_0.26g_versions_and_later_3."Task 6H: SKADI SOAPS" ("Enum"), s=w1636, f=State_Type_Definitions,_for_0.26g_versions_and_later_3."Task 6J: CAM BURST 3" ("Enum")) -> (s? t:f=w1632:T18)
                n588 = Select(t=State_Type_Definitions,_for_0.26g_versions_and_later_3."True Stop" ("Enum"), s=w1631, f=w1632) -> (s? t:f=w1638:T18)
                n589 = Select(t=w1638, s=w1634, f=State_Type_Definitions,_for_0.26g_versions_and_later_3."Task 6G: PROCESS IMAGE 2" ("Enum")) -> (s? t:f=w1640:T18)
              }
              frame "Exit" {
                n590 = for {
                  shift-right: [w1662] -> w1659
                  shift-left: w1656 -> [w1663]
                  tunnel: string[] ["STOP", "RESET ENCODERS", "RESET YAW", "ARDUINO MODE 0"] -> [w1661] mode=indexing
                  n591 = Enqueue Element(queue=w1663, element=w1661) -> (queue out=w1662:refnum<queue>)  [unwired: 2 in, 2 out]
                }
              }
            }
          }
          frame "Task 6H: SKADI SOAPS" {
            # "Ball > Soap > Gel > Pipe"
            # ">>> Motor control cluster >>>"
            # ">>> yStepper command>>>"
            n592 = Less Or Equal?(x=w1664, y=-20.0) -> (x <= y?=w1665:bool)
            n593 = Dequeue Element(queue=w1673, timeout in ms (-1)=w1672, error in (no error)=w1671) -> (element=w1670:T10)  [unwired: 3 out]
            n594 = case shown="\"Start Task 1\", Default" w1670 {
              tunnel: [w1686 State_Type_Definitions,_for_0.26g_versions_and_later_3."True Stop" ("Enum")] -> w1677
              tunnel: [w1688 w1705] -> w1676
              tunnel: [State_Type_Definitions,_for_0.26g_versions_and_later_3."Idle" ("Enum") State_Type_Definitions,_for_0.26g_versions_and_later_3."Shutdown" ("Enum")] -> w1678
              tunnel: w1674 -> [w1681 _]
              tunnel: w1675 -> [w1683 w1702]
              tunnel: w1665 -> [w1680 _]
              frame "Start Task 1", Default {
                # "Stays in Task 5D until the object is detected"
                n595 = Or(x=w1680, y=w1681) -> (x .or. y?=w1682:bool)
                n596 = case shown="False" w1682 {
                  tunnel: [w1692 w1698] -> w1688
                  tunnel: w1683 -> [w1690 w1696]
                  frame False {
                    n597 = for {
                      tunnel: string[] ["LEFT", "READ NAVX", "READ ENCODERS"] ("element") -> [w1693] mode=indexing
                      shift-right: [w1695] -> w1692
                      shift-left: w1690 -> [w1694]
                      n598 = Enqueue Element(queue=w1694, element=w1693) -> (queue out=w1695:refnum<queue>)  [unwired: 2 in, 2 out]
                    }
                  }
                  frame True {
                    n599 = for {
                      shift-right: [w1700] -> w1698
                      shift-left: w1696 -> [w1701]
                      tunnel: string[] ["RESET ENCODERS", "RESET YAW", "RESET FLAGS"] -> [w1699] mode=indexing
                      n600 = Enqueue Element(queue=w1701, element=w1699) -> (queue out=w1700:refnum<queue>)  [unwired: 2 in, 2 out]
                    }
                  }
                }
                n601 = Select(t=State_Type_Definitions,_for_0.26g_versions_and_later_3."True Stop" ("Enum"), s=w1681, f=State_Type_Definitions,_for_0.26g_versions_and_later_3."Task 6I: STILL WAITING 2" ("Enum")) -> (s? t:f=w1684:T18)
                n602 = Select(t=w1684, s=w1682, f=State_Type_Definitions,_for_0.26g_versions_and_later_3."Task 6H: SKADI SOAPS" ("Enum")) -> (s? t:f=w1686:T18)
              }
              frame "Exit" {
                n603 = for {
                  shift-right: [w1708] -> w1705
                  shift-left: w1702 -> [w1709]
                  tunnel: string[] ["STOP", "RESET ENCODERS", "RESET YAW", "ARDUINO MODE 0"] -> [w1707] mode=indexing
                  n604 = Enqueue Element(queue=w1709, element=w1707) -> (queue out=w1708:refnum<queue>)  [unwired: 2 in, 2 out]
                }
              }
            }
          }
          frame "Task 6I: STILL WAITING 2" {
            # "Ball > Soap > Gel > Pipe"
            # ">>> Motor control cluster >>>"
            # ">>> yStepper command>>>"
            n605 = local read "Rising Edge"() -> (w1711:bool)
            n606 = Dequeue Element(queue=w1717, timeout in ms (-1)=w1716, error in (no error)=w1715) -> (element=w1714:T10)  [unwired: 3 out]
            n607 = case shown="\"Start Task 1\", Default" w1714 {
              tunnel: [w1731 State_Type_Definitions,_for_0.26g_versions_and_later_3."True Stop" ("Enum")] -> w1721
              tunnel: [w1724 w1749] -> w1720
              tunnel: [State_Type_Definitions,_for_0.26g_versions_and_later_3."Idle" ("Enum") State_Type_Definitions,_for_0.26g_versions_and_later_3."Shutdown" ("Enum")] -> w1722
              tunnel: w1718 -> [w1728 _]
              tunnel: w1719 -> [w1725 w1746]
              tunnel: w1711 -> [w1726 _]
              frame "Start Task 1", Default {
                # "Stays in Task 5D until the object is detected"
                n608 = Or(x=w1726, y=w1728) -> (x .or. y?=w1723:bool)
                n609 = case shown="False" w1723 {
                  tunnel: [w1736 w1742] -> w1724
                  tunnel: w1725 -> [w1734 w1741]
                  frame False {
                    n610 = for {
                      tunnel: string[] ["Z STEPPER CAM HEIGHT", "READ STEPPER VALUES"] ("element") -> [w1737] mode=indexing
                      shift-right: [w1739] -> w1736
                      shift-left: w1734 -> [w1738]
                      n611 = Enqueue Element(queue=w1738, element=w1737) -> (queue out=w1739:refnum<queue>)  [unwired: 2 in, 2 out]
                    }
                  }
                  frame True {
                    n612 = for {
                      shift-right: [w1744] -> w1742
                      shift-left: w1741 -> [w1745]
                      tunnel: string[] ["OPEN LOG CAM", "SET TIMER 2", "OPEN IMAQ REF", "", ""] -> [w1743] mode=indexing
                      n613 = Enqueue Element(queue=w1745, element=w1743) -> (queue out=w1744:refnum<queue>)  [unwired: 2 in, 2 out]
                    }
                  }
                }
                n614 = Select(t=State_Type_Definitions,_for_0.26g_versions_and_later_3."True Stop" ("Enum"), s=w1728, f=State_Type_Definitions,_for_0.26g_versions_and_later_3."Task 6J: CAM BURST 3" ("Enum")) -> (s? t:f=w1729:T18)
                n615 = Select(t=w1729, s=w1723, f=State_Type_Definitions,_for_0.26g_versions_and_later_3."Task 6I: STILL WAITING 2" ("Enum")) -> (s? t:f=w1731:T18)
              }
              frame "Exit" {
                n616 = for {
                  shift-right: [w1752] -> w1749
                  shift-left: w1746 -> [w1753]
                  tunnel: string[] ["STOP", "RESET ENCODERS", "RESET YAW", "ARDUINO MODE 0"] -> [w1751] mode=indexing
                  n617 = Enqueue Element(queue=w1753, element=w1751) -> (queue out=w1752:refnum<queue>)  [unwired: 2 in, 2 out]
                }
              }
            }
          }
          frame "Task 6J: CAM BURST 3" {
            # ">> Manual override >>"
            # ">>> Motor control cluster >>>"
            # ">>> yStepper command>>>"
            n618 = Dequeue Element(queue=w1765, timeout in ms (-1)=w1763, error in (no error)=w1764) -> (element=w1762:T10)  [unwired: 3 out]
            n619 = case shown="\"Start Task 1\", Default" w1762 {
              tunnel: [w1773 State_Type_Definitions,_for_0.26g_versions_and_later_3."True Stop" ("Enum")] -> w1759
              tunnel: [w1771 w1791] -> w1766
              tunnel: [State_Type_Definitions,_for_0.26g_versions_and_later_3."Idle" ("Enum") State_Type_Definitions,_for_0.26g_versions_and_later_3."Shutdown" ("Enum")] -> w1760
              tunnel: w1761 -> [w1769 _]
              tunnel: w1758 -> [w1770 w1788]
              tunnel: w1754 -> [w1767 _]
              frame "Start Task 1", Default {
                n620 = Or(x=w1767, y=w1769) -> (x .or. y?=w1768:bool)
                n621 = case shown="True" w1768 {
                  tunnel: [w1778 w1784] -> w1771
                  tunnel: w1770 -> [w1776 w1782]
                  frame False {
                    n622 = for {
                      tunnel: string[] ["CAM ACQ", "START TIMER"] ("element") -> [w1779] mode=indexing
                      shift-right: [w1781] -> w1778
                      shift-left: w1776 -> [w1780]
                      n623 = Enqueue Element(queue=w1780, element=w1779) -> (queue out=w1781:refnum<queue>)  [unwired: 2 in, 2 out]
                    }
                  }
                  frame True {
                    n624 = for {
                      shift-right: [w1786] -> w1784
                      shift-left: w1782 -> [w1787]
                      tunnel: string[] ["CAM CLOSE", "PROCESS IMAGE", "SET TIMER 2", "RESET ENCODERS"] -> [w1785] mode=indexing
                      n625 = Enqueue Element(queue=w1787, element=w1785) -> (queue out=w1786:refnum<queue>)  [unwired: 2 in, 2 out]
                    }
                  }
                }
                n626 = Select(t=State_Type_Definitions,_for_0.26g_versions_and_later_3."Task 6K: PROCESS IMAGE 3" ("Enum"), s=w1768, f=State_Type_Definitions,_for_0.26g_versions_and_later_3."Task 6J: CAM BURST 3" ("Enum")) -> (s? t:f=w1773:T18)
              }
              frame "Exit" {
                # ">> State after true stop >>"
                # ">> Goes to true stop >>"
                n627 = for {
                  shift-right: [w1794] -> w1791
                  shift-left: w1788 -> [w1795]
                  tunnel: string[] ["STOP", "RESET ENCODERS", "RESET YAW", ""] -> [w1793] mode=indexing
                  n628 = Enqueue Element(queue=w1795, element=w1793) -> (queue out=w1794:refnum<queue>)  [unwired: 2 in, 2 out]
                }
              }
            }
          }
          frame "Task 6K: PROCESS IMAGE 3" {
            # "Ball > Soap > Gel > Pipe"
            # ">>> Motor control cluster >>>"
            # ">>> yStepper command>>>"
            n629 = Dequeue Element(queue=w1804, timeout in ms (-1)=w1803, error in (no error)=w1802) -> (element=w1801:T10)  [unwired: 3 out]
            n630 = case shown="\"Start Task 1\", Default" w1801 {
              tunnel: [w1820 State_Type_Definitions,_for_0.26g_versions_and_later_3."True Stop" ("Enum")] -> w1808
              tunnel: [w1822 w1839] -> w1807
              tunnel: [State_Type_Definitions,_for_0.26g_versions_and_later_3."Idle" ("Enum") State_Type_Definitions,_for_0.26g_versions_and_later_3."Shutdown" ("Enum")] -> w1809
              tunnel: w1805 -> [w1811 _]
              tunnel: w1806 -> [w1817 w1836]
              tunnel: w1797 -> [w1815 _]
              tunnel: w1796 -> [w1816 _]
              frame "Start Task 1", Default {
                # "Stays in Task 5D until the object is detected"
                n631 = Or(x=w1815, y=w1811) -> (x .or. y?=w1814:bool)
                n632 = case shown="True" w1814 {
                  tunnel: [w1826 w1832] -> w1822
                  tunnel: w1817 -> [w1824 w1830]
                  frame False {
                    n633 = for {
                      tunnel: string[] ["START TIMER", "PROCESS IMAGE", ""] ("element") -> [w1827] mode=indexing
                      shift-right: [w1829] -> w1826
                      shift-left: w1824 -> [w1828]
                      n634 = Enqueue Element(queue=w1828, element=w1827) -> (queue out=w1829:refnum<queue>)  [unwired: 2 in, 2 out]
                    }
                  }
                  frame True {
                    n635 = for {
                      shift-right: [w1834] -> w1832
                      shift-left: w1830 -> [w1835]
                      tunnel: string[] ["RESET ENCODERS", "RESET YAW", ""] -> [w1833] mode=indexing
                      n636 = Enqueue Element(queue=w1835, element=w1833) -> (queue out=w1834:refnum<queue>)  [unwired: 2 in, 2 out]
                    }
                  }
                }
                n637 = Select(t=State_Type_Definitions,_for_0.26g_versions_and_later_3."Task 6L: JAM IT IN" ("Enum"), s=w1816, f=State_Type_Definitions,_for_0.26g_versions_and_later_3."Task 6N: CAM BURST 4" ("Enum")) -> (s? t:f=w1812:T18)
                n638 = Select(t=State_Type_Definitions,_for_0.26g_versions_and_later_3."True Stop" ("Enum"), s=w1811, f=w1812) -> (s? t:f=w1818:T18)
                n639 = Select(t=w1818, s=w1814, f=State_Type_Definitions,_for_0.26g_versions_and_later_3."Task 6K: PROCESS IMAGE 3" ("Enum")) -> (s? t:f=w1820:T18)
              }
              frame "Exit" {
                n640 = for {
                  shift-right: [w1842] -> w1839
                  shift-left: w1836 -> [w1843]
                  tunnel: string[] ["STOP", "RESET ENCODERS", "RESET YAW", "ARDUINO MODE 0"] -> [w1841] mode=indexing
                  n641 = Enqueue Element(queue=w1843, element=w1841) -> (queue out=w1842:refnum<queue>)  [unwired: 2 in, 2 out]
                }
              }
            }
          }
          frame "Task 6L: JAM IT IN" {
            # "Ball > Soap > Gel > Pipe"
            # ">>> Motor control cluster >>>"
            # ">>> yStepper command>>>"
            n642 = Less Or Equal?(x=w1844, y=-20.0) -> (x <= y?=w1845:bool)
            n643 = Dequeue Element(queue=w1853, timeout in ms (-1)=w1852, error in (no error)=w1851) -> (element=w1850:T10)  [unwired: 3 out]
            n644 = case shown="\"Start Task 1\", Default" w1850 {
              tunnel: [w1866 State_Type_Definitions,_for_0.26g_versions_and_later_3."True Stop" ("Enum")] -> w1857
              tunnel: [w1868 w1885] -> w1856
              tunnel: [State_Type_Definitions,_for_0.26g_versions_and_later_3."Idle" ("Enum") State_Type_Definitions,_for_0.26g_versions_and_later_3."Shutdown" ("Enum")] -> w1858
              tunnel: w1854 -> [w1861 _]
              tunnel: w1855 -> [w1863 w1882]
              tunnel: w1845 -> [w1860 _]
              frame "Start Task 1", Default {
                # "Stays in Task 5D until the object is detected"
                n645 = Or(x=w1860, y=w1861) -> (x .or. y?=w1862:bool)
                n646 = case shown="False" w1862 {
                  tunnel: [w1872 w1878] -> w1868
                  tunnel: w1863 -> [w1870 w1876]
                  frame False {
                    n647 = for {
                      tunnel: string[] ["REVERSE", "READ NAVX", "READ ENCODERS"] ("element") -> [w1873] mode=indexing
                      shift-right: [w1875] -> w1872
                      shift-left: w1870 -> [w1874]
                      n648 = Enqueue Element(queue=w1874, element=w1873) -> (queue out=w1875:refnum<queue>)  [unwired: 2 in, 2 out]
                    }
                  }
                  frame True {
                    n649 = for {
                      shift-right: [w1880] -> w1878
                      shift-left: w1876 -> [w1881]
                      tunnel: string[] ["RESET ENCODERS", "RESET YAW", "RESET FLAGS"] -> [w1879] mode=indexing
                      n650 = Enqueue Element(queue=w1881, element=w1879) -> (queue out=w1880:refnum<queue>)  [unwired: 2 in, 2 out]
                    }
                  }
                }
                n651 = Select(t=State_Type_Definitions,_for_0.26g_versions_and_later_3."True Stop" ("Enum"), s=w1861, f=State_Type_Definitions,_for_0.26g_versions_and_later_3."Task 6M: STILL WAITING 3" ("Enum")) -> (s? t:f=w1864:T18)
                n652 = Select(t=w1864, s=w1862, f=State_Type_Definitions,_for_0.26g_versions_and_later_3."Task 6L: JAM IT IN" ("Enum")) -> (s? t:f=w1866:T18)
              }
              frame "Exit" {
                n653 = for {
                  shift-right: [w1888] -> w1885
                  shift-left: w1882 -> [w1889]
                  tunnel: string[] ["STOP", "RESET ENCODERS", "RESET YAW", "ARDUINO MODE 0"] -> [w1887] mode=indexing
                  n654 = Enqueue Element(queue=w1889, element=w1887) -> (queue out=w1888:refnum<queue>)  [unwired: 2 in, 2 out]
                }
              }
            }
          }
          frame "Task 6M: STILL WAITING 3" {
            # "Ball > Soap > Gel > Pipe"
            # ">>> Motor control cluster >>>"
            # ">>> yStepper command>>>"
            n655 = local read "Rising Edge"() -> (w1891:bool)
            n656 = Dequeue Element(queue=w1897, timeout in ms (-1)=w1896, error in (no error)=w1895) -> (element=w1894:T10)  [unwired: 3 out]
            n657 = case shown="\"Start Task 1\", Default" w1894 {
              tunnel: [w1911 State_Type_Definitions,_for_0.26g_versions_and_later_3."True Stop" ("Enum")] -> w1901
              tunnel: [w1904 w1929] -> w1900
              tunnel: [State_Type_Definitions,_for_0.26g_versions_and_later_3."Idle" ("Enum") State_Type_Definitions,_for_0.26g_versions_and_later_3."Shutdown" ("Enum")] -> w1902
              tunnel: w1898 -> [w1908 _]
              tunnel: w1899 -> [w1905 w1926]
              tunnel: w1891 -> [w1906 _]
              frame "Start Task 1", Default {
                # "Stays in Task 5D until the object is detected"
                n658 = Or(x=w1906, y=w1908) -> (x .or. y?=w1903:bool)
                n659 = case shown="False" w1903 {
                  tunnel: [w1916 w1922] -> w1904
                  tunnel: w1905 -> [w1914 w1921]
                  frame False {
                    n660 = for {
                      tunnel: string[] ["Z STEPPER CAM HEIGHT", "READ STEPPER VALUES"] ("element") -> [w1917] mode=indexing
                      shift-right: [w1919] -> w1916
                      shift-left: w1914 -> [w1918]
                      n661 = Enqueue Element(queue=w1918, element=w1917) -> (queue out=w1919:refnum<queue>)  [unwired: 2 in, 2 out]
                    }
                  }
                  frame True {
                    n662 = for {
                      shift-right: [w1924] -> w1922
                      shift-left: w1921 -> [w1925]
                      tunnel: string[] ["OPEN LOG CAM", "SET TIMER 2", "OPEN IMAQ REF", "", ""] -> [w1923] mode=indexing
                      n663 = Enqueue Element(queue=w1925, element=w1923) -> (queue out=w1924:refnum<queue>)  [unwired: 2 in, 2 out]
                    }
                  }
                }
                n664 = Select(t=State_Type_Definitions,_for_0.26g_versions_and_later_3."True Stop" ("Enum"), s=w1908, f=State_Type_Definitions,_for_0.26g_versions_and_later_3."Task 6N: CAM BURST 4" ("Enum")) -> (s? t:f=w1909:T18)
                n665 = Select(t=w1909, s=w1903, f=State_Type_Definitions,_for_0.26g_versions_and_later_3."Task 6M: STILL WAITING 3" ("Enum")) -> (s? t:f=w1911:T18)
              }
              frame "Exit" {
                n666 = for {
                  shift-right: [w1932] -> w1929
                  shift-left: w1926 -> [w1933]
                  tunnel: string[] ["STOP", "RESET ENCODERS", "RESET YAW", "ARDUINO MODE 0"] -> [w1931] mode=indexing
                  n667 = Enqueue Element(queue=w1933, element=w1931) -> (queue out=w1932:refnum<queue>)  [unwired: 2 in, 2 out]
                }
              }
            }
          }
          frame "Task 6N: CAM BURST 4" {
            # ">> Manual override >>"
            # ">>> Motor control cluster >>>"
            # ">>> yStepper command>>>"
            n668 = Dequeue Element(queue=w1945, timeout in ms (-1)=w1943, error in (no error)=w1944) -> (element=w1942:T10)  [unwired: 3 out]
            n669 = case shown="\"Start Task 1\", Default" w1942 {
              tunnel: [w1953 State_Type_Definitions,_for_0.26g_versions_and_later_3."True Stop" ("Enum")] -> w1939
              tunnel: [w1951 w1971] -> w1946
              tunnel: [State_Type_Definitions,_for_0.26g_versions_and_later_3."Idle" ("Enum") State_Type_Definitions,_for_0.26g_versions_and_later_3."Shutdown" ("Enum")] -> w1940
              tunnel: w1941 -> [w1949 _]
              tunnel: w1938 -> [w1950 w1968]
              tunnel: w1934 -> [w1947 _]
              frame "Start Task 1", Default {
                n670 = Or(x=w1947, y=w1949) -> (x .or. y?=w1948:bool)
                n671 = case shown="True" w1948 {
                  tunnel: [w1958 w1964] -> w1951
                  tunnel: w1950 -> [w1956 w1962]
                  frame False {
                    n672 = for {
                      tunnel: string[] ["CAM ACQ", "START TIMER"] ("element") -> [w1959] mode=indexing
                      shift-right: [w1961] -> w1958
                      shift-left: w1956 -> [w1960]
                      n673 = Enqueue Element(queue=w1960, element=w1959) -> (queue out=w1961:refnum<queue>)  [unwired: 2 in, 2 out]
                    }
                  }
                  frame True {
                    n674 = for {
                      shift-right: [w1966] -> w1964
                      shift-left: w1962 -> [w1967]
                      tunnel: string[] ["CAM CLOSE", "PROCESS IMAGE", "SET TIMER 2", "RESET ENCODERS"] -> [w1965] mode=indexing
                      n675 = Enqueue Element(queue=w1967, element=w1965) -> (queue out=w1966:refnum<queue>)  [unwired: 2 in, 2 out]
                    }
                  }
                }
                n676 = Select(t=State_Type_Definitions,_for_0.26g_versions_and_later_3."Task 6O: PROCESS IMAGE 4" ("Enum"), s=w1948, f=State_Type_Definitions,_for_0.26g_versions_and_later_3."Task 6N: CAM BURST 4" ("Enum")) -> (s? t:f=w1953:T18)
              }
              frame "Exit" {
                # ">> State after true stop >>"
                # ">> Goes to true stop >>"
                n677 = for {
                  shift-right: [w1974] -> w1971
                  shift-left: w1968 -> [w1975]
                  tunnel: string[] ["STOP", "RESET ENCODERS", "RESET YAW", ""] -> [w1973] mode=indexing
                  n678 = Enqueue Element(queue=w1975, element=w1973) -> (queue out=w1974:refnum<queue>)  [unwired: 2 in, 2 out]
                }
              }
            }
          }
          frame "Task 6O: PROCESS IMAGE 4" {
            # "Ball > Soap > Gel > Pipe"
            # ">>> Motor control cluster >>>"
            # ">>> yStepper command>>>"
            n679 = Dequeue Element(queue=w1984, timeout in ms (-1)=w1983, error in (no error)=w1982) -> (element=w1981:T10)  [unwired: 3 out]
            n680 = case shown="\"Start Task 1\", Default" w1981 {
              tunnel: [w2000 State_Type_Definitions,_for_0.26g_versions_and_later_3."True Stop" ("Enum")] -> w1988
              tunnel: [w2002 w2019] -> w1987
              tunnel: [State_Type_Definitions,_for_0.26g_versions_and_later_3."Idle" ("Enum") State_Type_Definitions,_for_0.26g_versions_and_later_3."Shutdown" ("Enum")] -> w1989
              tunnel: w1985 -> [w1991 _]
              tunnel: w1986 -> [w1997 w2016]
              tunnel: w1977 -> [w1995 _]
              tunnel: w1976 -> [w1996 _]
              frame "Start Task 1", Default {
                # "Stays in Task 5D until the object is detected"
                n681 = Or(x=w1995, y=w1991) -> (x .or. y?=w1994:bool)
                n682 = case shown="True" w1994 {
                  tunnel: [w2006 w2012] -> w2002
                  tunnel: w1997 -> [w2004 w2010]
                  frame False {
                    n683 = for {
                      tunnel: string[] ["START TIMER", "PROCESS IMAGE", ""] ("element") -> [w2007] mode=indexing
                      shift-right: [w2009] -> w2006
                      shift-left: w2004 -> [w2008]
                      n684 = Enqueue Element(queue=w2008, element=w2007) -> (queue out=w2009:refnum<queue>)  [unwired: 2 in, 2 out]
                    }
                  }
                  frame True {
                    n685 = for {
                      shift-right: [w2014] -> w2012
                      shift-left: w2010 -> [w2015]
                      tunnel: string[] ["RESET ENCODERS", "RESET YAW", ""] -> [w2013] mode=indexing
                      n686 = Enqueue Element(queue=w2015, element=w2013) -> (queue out=w2014:refnum<queue>)  [unwired: 2 in, 2 out]
                    }
                  }
                }
                n687 = Select(t=State_Type_Definitions,_for_0.26g_versions_and_later_3."Task 6P: PIPE BOMB" ("Enum"), s=w1996, f=State_Type_Definitions,_for_0.26g_versions_and_later_3."Task 6B: CAM BURST" ("Enum")) -> (s? t:f=w1992:T18)
                n688 = Select(t=State_Type_Definitions,_for_0.26g_versions_and_later_3."True Stop" ("Enum"), s=w1991, f=w1992) -> (s? t:f=w1998:T18)
                n689 = Select(t=w1998, s=w1994, f=State_Type_Definitions,_for_0.26g_versions_and_later_3."Task 6O: PROCESS IMAGE 4" ("Enum")) -> (s? t:f=w2000:T18)
              }
              frame "Exit" {
                n690 = for {
                  shift-right: [w2022] -> w2019
                  shift-left: w2016 -> [w2023]
                  tunnel: string[] ["STOP", "RESET ENCODERS", "RESET YAW", "ARDUINO MODE 0"] -> [w2021] mode=indexing
                  n691 = Enqueue Element(queue=w2023, element=w2021) -> (queue out=w2022:refnum<queue>)  [unwired: 2 in, 2 out]
                }
              }
            }
          }
          frame "Task 6P: PIPE BOMB" {
            # "Ball > Soap > Gel > Pipe"
            # ">>> Motor control cluster >>>"
            # ">>> yStepper command>>>"
            n692 = Greater Or Equal?(x=w2024, y=20.0) -> (x >= y?=w2025:bool)
            n693 = Dequeue Element(queue=w2033, timeout in ms (-1)=w2032, error in (no error)=w2031) -> (element=w2030:T10)  [unwired: 3 out]
            n694 = case shown="\"Start Task 1\", Default" w2030 {
              tunnel: [w2046 State_Type_Definitions,_for_0.26g_versions_and_later_3."True Stop" ("Enum")] -> w2037
              tunnel: [w2048 w2065] -> w2036
              tunnel: [State_Type_Definitions,_for_0.26g_versions_and_later_3."Idle" ("Enum") State_Type_Definitions,_for_0.26g_versions_and_later_3."Shutdown" ("Enum")] -> w2038
              tunnel: w2034 -> [w2041 _]
              tunnel: w2035 -> [w2043 w2062]
              tunnel: w2025 -> [w2040 _]
              frame "Start Task 1", Default {
                # "Stays in Task 5D until the object is detected"
                n695 = Or(x=w2040, y=w2041) -> (x .or. y?=w2042:bool)
                n696 = case shown="False" w2042 {
                  tunnel: [w2052 w2058] -> w2048
                  tunnel: w2043 -> [w2050 w2056]
                  frame False {
                    n697 = for {
                      tunnel: string[] ["FORWARD", "READ NAVX", "READ ENCODERS"] ("element") -> [w2053] mode=indexing
                      shift-right: [w2055] -> w2052
                      shift-left: w2050 -> [w2054]
                      n698 = Enqueue Element(queue=w2054, element=w2053) -> (queue out=w2055:refnum<queue>)  [unwired: 2 in, 2 out]
                    }
                  }
                  frame True {
                    n699 = for {
                      shift-right: [w2060] -> w2058
                      shift-left: w2056 -> [w2061]
                      tunnel: string[] ["RESET ENCODERS", "RESET YAW", "RESET FLAGS"] -> [w2059] mode=indexing
                      n700 = Enqueue Element(queue=w2061, element=w2059) -> (queue out=w2060:refnum<queue>)  [unwired: 2 in, 2 out]
                    }
                  }
                }
                n701 = Select(t=State_Type_Definitions,_for_0.26g_versions_and_later_3."True Stop" ("Enum"), s=w2041, f=State_Type_Definitions,_for_0.26g_versions_and_later_3."Task 5F: ARM GRAB HEIGHT" ("Enum")) -> (s? t:f=w2044:T18)
                n702 = Select(t=w2044, s=w2042, f=State_Type_Definitions,_for_0.26g_versions_and_later_3."Task 6P: PIPE BOMB" ("Enum")) -> (s? t:f=w2046:T18)
              }
              frame "Exit" {
                n703 = for {
                  shift-right: [w2068] -> w2065
                  shift-left: w2062 -> [w2069]
                  tunnel: string[] ["STOP", "RESET ENCODERS", "RESET YAW", "ARDUINO MODE 0"] -> [w2067] mode=indexing
                  n704 = Enqueue Element(queue=w2069, element=w2067) -> (queue out=w2068:refnum<queue>)  [unwired: 2 in, 2 out]
                }
              }
            }
          }
          frame "Task 7" {
          }
          frame "Task 8A: RAISE ARM" {
            # ">>> Motor control cluster >>>"
            # ">>> yStepper command>>>"
            # ">> Manual override >>"
            n705 = Dequeue Element(queue=w2086, timeout in ms (-1)=w2085, error in (no error)=w2087) -> (element=w2084:T10)  [unwired: 3 out]
            n706 = Equal?(x=w2083, y=u8 60) -> (x = y?=w2081:bool)
            n707 = case shown="\"Start Task 1\", Default" w2084 {
              tunnel: [w2097 State_Type_Definitions,_for_0.26g_versions_and_later_3."True Stop" ("Enum")] -> w2088
              tunnel: [w2100 w2117] -> w2089
              tunnel: [State_Type_Definitions,_for_0.26g_versions_and_later_3."Idle" ("Enum") State_Type_Definitions,_for_0.26g_versions_and_later_3."Shutdown" ("Enum")] -> w2090
              tunnel: w2081 -> [w2096 _]
              tunnel: w2080 -> [w2095 _]
              tunnel: w2079 -> [w2091 w2114]
              frame "Start Task 1", Default {
                # "Stays in Task 5_A until stepper reaches desired \nheight"
                # "T: Go back to idle, F: Continue with task\""
                # ">> Manual override >>"
                n708 = case shown="False" w2096 {
                  tunnel: [w2104 w2110] -> w2100
                  tunnel: w2091 -> [w2102 w2108]
                  frame False {
                    n709 = for {
                      tunnel: string[] ["Z STEPPER CAM HEIGHT", "READ STEPPER VALUES", "READ IR"] ("element") -> [w2105] mode=indexing
                      shift-right: [w2107] -> w2104
                      shift-left: w2102 -> [w2106]
                      n710 = Enqueue Element(queue=w2106, element=w2105) -> (queue out=w2107:refnum<queue>)  [unwired: 2 in, 2 out]
                    }
                  }
                  frame True {
                    n711 = for {
                      shift-right: [w2112] -> w2110
                      shift-left: w2108 -> [w2113]
                      tunnel: string[] ["RESET YAW", "RESET ENCODERS", "READ IR"] -> [w2111] mode=indexing
                      n712 = Enqueue Element(queue=w2113, element=w2111) -> (queue out=w2112:refnum<queue>)  [unwired: 2 in, 2 out]
                    }
                  }
                }
                n713 = Or(x=w2096, y=w2095) -> (x .or. y?=w2098:bool)
                n714 = Select(t=State_Type_Definitions,_for_0.26g_versions_and_later_3."True Stop" ("Enum"), s=w2095, f=State_Type_Definitions,_for_0.26g_versions_and_later_3."Task 8B: MOVE TO BOX" ("Enum")) -> (s? t:f=w2092:T18)
                n715 = Select(t=w2092, s=w2098, f=State_Type_Definitions,_for_0.26g_versions_and_later_3."Task 8A: RAISE ARM" ("Enum")) -> (s? t:f=w2097:T18)
              }
              frame "Exit" {
                n716 = for {
                  shift-right: [w2120] -> w2117
                  shift-left: w2114 -> [w2121]
                  tunnel: string[] ["STOP", "RESET ENCODERS", "RESET YAW", "ARDUINO MODE 0"] -> [w2119] mode=indexing
                  n717 = Enqueue Element(queue=w2121, element=w2119) -> (queue out=w2120:refnum<queue>)  [unwired: 2 in, 2 out]
                }
              }
            }
          }
          frame "Task 8B: MOVE TO BOX" {
            w2131 = u8 15 ("y")
            # "High voltage: 70"
            # ">>> yStepper command>>>"
            n718 = Less?(x=w2128, y=w2131) -> (x < y?=w2129:bool)
            n719 = Less?(x=w2127, y=w2131) -> (x < y?=w2130:bool)
            n720 = And(x=w2130, y=w2129) -> ()  [unwired: 1 out]
            n721 = Dequeue Element(queue=w2135, timeout in ms (-1)=w2134, error in (no error)=w2136) -> (element=w2133:T10)  [unwired: 3 out]
            n722 = Less?(x=w2124, y=40.0) -> (x < y?=w2122:bool)
            n723 = case shown="\"Start Task 1\", Default" w2133 {
              tunnel: [w2148 State_Type_Definitions,_for_0.26g_versions_and_later_3."True Stop" ("Enum")] -> w2138
              tunnel: [w2151 w2168] -> w2137
              tunnel: [State_Type_Definitions,_for_0.26g_versions_and_later_3."Idle" ("Enum") State_Type_Definitions,_for_0.26g_versions_and_later_3."Shutdown" ("Enum")] -> w2139
              tunnel: w2141 -> [w2147 _]
              tunnel: w2140 -> [w2143 w2165]
              tunnel: w2122 -> [w2142 _]
              frame "Start Task 1", Default {
                # "Stays in Task 5_B to capture image over 5 seconds"
                # "T: Go back to idle, F: Continue with task\""
                # ">> Manual override >>"
                n724 = case shown="True" w2142 {
                  tunnel: [w2155 w2161] -> w2151
                  tunnel: w2143 -> [w2153 w2159]
                  frame False {
                    n725 = for {
                      tunnel: string[] ["FORWARD", "READ IR", "READ NAVX"] ("element") -> [w2156] mode=indexing
                      shift-right: [w2158] -> w2155
                      shift-left: w2153 -> [w2157]
                      n726 = Enqueue Element(queue=w2157, element=w2156) -> (queue out=w2158:refnum<queue>)  [unwired: 2 in, 2 out]
                    }
                  }
                  frame True {
                    n727 = for {
                      shift-right: [w2163] -> w2161
                      shift-left: w2159 -> [w2164]
                      tunnel: string[] ["STOP", "RESET ENCODERS", "OPEN LOG CAM", "SET TIMER 2", "OPEN IMAQ REF"] -> [w2162] mode=indexing
                      n728 = Enqueue Element(queue=w2164, element=w2162) -> (queue out=w2163:refnum<queue>)  [unwired: 2 in, 2 out]
                    }
                  }
                }
                n729 = Or(x=w2142, y=w2147) -> (x .or. y?=w2149:bool)
                n730 = Select(t=State_Type_Definitions,_for_0.26g_versions_and_later_3."True Stop" ("Enum"), s=w2147, f=State_Type_Definitions,_for_0.26g_versions_and_later_3."Task 8C: CAM BURST" ("Enum")) -> (s? t:f=w2144:T18)
                n731 = Select(t=w2144, s=w2149, f=State_Type_Definitions,_for_0.26g_versions_and_later_3."Task 8B: MOVE TO BOX" ("Enum")) -> (s? t:f=w2148:T18)
              }
              frame "Exit" {
                n732 = for {
                  shift-right: [w2171] -> w2168
                  shift-left: w2165 -> [w2172]
                  tunnel: string[] ["STOP", "RESET ENCODERS", "RESET YAW", "ARDUINO MODE 0"] -> [w2170] mode=indexing
                  n733 = Enqueue Element(queue=w2172, element=w2170) -> (queue out=w2171:refnum<queue>)  [unwired: 2 in, 2 out]
                }
              }
            }
          }
          frame "Task 8C: CAM BURST" {
            # ">>> Motor control cluster >>>"
            # ">>> yStepper command>>>"
            # ">> Manual override >>"
            n734 = Dequeue Element(queue=w2183, timeout in ms (-1)=w2182, error in (no error)=w2181) -> (element=w2180:T10)  [unwired: 3 out]
            n735 = case shown="\"Start Task 1\", Default" w2180 {
              tunnel: [w2192 State_Type_Definitions,_for_0.26g_versions_and_later_3."True Stop" ("Enum")] -> w2185
              tunnel: [w2195 w2212] -> w2178
              tunnel: [State_Type_Definitions,_for_0.26g_versions_and_later_3."Idle" ("Enum") State_Type_Definitions,_for_0.26g_versions_and_later_3."Shutdown" ("Enum")] -> w2177
              tunnel: w2179 -> [w2186 _]
              tunnel: w2184 -> [w2191 w2209]
              tunnel: w2175 -> [w2190 _]
              frame "Start Task 1", Default {
                # ">> Is time up? >>"
                # "Determines if object is in range to pick up"
                # ">> Manual override >>"
                n736 = case shown="True" w2190 {
                  tunnel: [w2199 w2205] -> w2195
                  tunnel: w2191 -> [w2197 w2203]
                  frame False {
                    n737 = for {
                      tunnel: string[] ["CAM ACQ", "START TIMER"] ("element") -> [w2200] mode=indexing
                      shift-right: [w2202] -> w2199
                      shift-left: w2197 -> [w2201]
                      n738 = Enqueue Element(queue=w2201, element=w2200) -> (queue out=w2202:refnum<queue>)  [unwired: 2 in, 2 out]
                    }
                  }
                  frame True {
                    n739 = for {
                      shift-right: [w2207] -> w2205
                      shift-left: w2203 -> [w2208]
                      tunnel: string[] ["CAM CLOSE", "PROCESS IMAGE", "SET TIMER 2"] -> [w2206] mode=indexing
                      n740 = Enqueue Element(queue=w2208, element=w2206) -> (queue out=w2207:refnum<queue>)  [unwired: 2 in, 2 out]
                    }
                  }
                }
                n741 = Or(x=w2190, y=w2186) -> (x .or. y?=w2193:bool)
                n742 = Select(t=State_Type_Definitions,_for_0.26g_versions_and_later_3."True Stop" ("Enum"), s=w2186, f=State_Type_Definitions,_for_0.26g_versions_and_later_3."Task 8D: PROCESS IMAGE" ("Enum")) -> (s? t:f=w2188:T18)
                n743 = Select(t=w2188, s=w2193, f=State_Type_Definitions,_for_0.26g_versions_and_later_3."Task 8C: CAM BURST" ("Enum")) -> (s? t:f=w2192:T18)
              }
              frame "Exit" {
                n744 = for {
                  shift-right: [w2215] -> w2212
                  shift-left: w2209 -> [w2216]
                  tunnel: string[] ["STOP", "RESET ENCODERS", "RESET YAW", "ARDUINO MODE 0"] -> [w2214] mode=indexing
                  n745 = Enqueue Element(queue=w2216, element=w2214) -> (queue out=w2215:refnum<queue>)  [unwired: 2 in, 2 out]
                }
              }
            }
          }
          frame "Task 8D: PROCESS IMAGE" {
            # ">>> Motor control cluster >>>"
            # ">>> yStepper command>>>"
            n746 = Dequeue Element(queue=w2225, timeout in ms (-1)=w2224, error in (no error)=w2223) -> (element=w2222:T10)  [unwired: 3 out]
            n747 = case shown="\"Start Task 1\", Default" w2222 {
              tunnel: [w2240 State_Type_Definitions,_for_0.26g_versions_and_later_3."True Stop" ("Enum")] -> w2229
              tunnel: [w2243 w2260] -> w2228
              tunnel: [State_Type_Definitions,_for_0.26g_versions_and_later_3."Idle" ("Enum") State_Type_Definitions,_for_0.26g_versions_and_later_3."Shutdown" ("Enum")] -> w2230
              tunnel: w2226 -> [w2239 _]
              tunnel: w2227 -> [w2236 w2257]
              tunnel: w2217 -> [w2235 _]
              tunnel: w2218 -> [w2234 _]
              frame "Start Task 1", Default {
                # ">> T: Breaks out of state loop; F: Stays in loop>>"
                # ">> Manual override >>"
                # ">> Checks if time is up>>"
                # "Stays in Task 5D until the object is detected"
                # "T: Go back to idle, F: Continue with task\""
                # ">> Manual override >>"
                n748 = case shown="False" w2235 {
                  tunnel: [w2247 w2253] -> w2243
                  tunnel: w2236 -> [w2245 w2251]
                  frame False {
                    n749 = for {
                      tunnel: string[] ["START TIMER", "PROCESS IMAGE", ""] ("element") -> [w2248] mode=indexing
                      shift-right: [w2250] -> w2247
                      shift-left: w2245 -> [w2249]
                      n750 = Enqueue Element(queue=w2249, element=w2248) -> (queue out=w2250:refnum<queue>)  [unwired: 2 in, 2 out]
                    }
                  }
                  frame True {
                    n751 = for {
                      shift-right: [w2255] -> w2253
                      shift-left: w2251 -> [w2256]
                      tunnel: string[] ["RESET ENCODERS", "", ""] -> [w2254] mode=indexing
                      n752 = Enqueue Element(queue=w2256, element=w2254) -> (queue out=w2255:refnum<queue>)  [unwired: 2 in, 2 out]
                    }
                  }
                }
                n753 = Or(x=w2235, y=w2239) -> (x .or. y?=w2241:bool)
                n754 = Select(t=State_Type_Definitions,_for_0.26g_versions_and_later_3."Task 8E: ROBOT ADJUST" ("Enum"), s=w2234, f=State_Type_Definitions,_for_0.26g_versions_and_later_3."True Stop" ("Enum")) -> (s? t:f=w2231:T18)
                n755 = Select(t=State_Type_Definitions,_for_0.26g_versions_and_later_3."True Stop" ("Enum"), s=w2239, f=w2231) -> (s? t:f=w2237:T18)
                n756 = Select(t=w2237, s=w2241, f=State_Type_Definitions,_for_0.26g_versions_and_later_3."Task 8D: PROCESS IMAGE" ("Enum")) -> (s? t:f=w2240:T18)
              }
              frame "Exit" {
                n757 = for {
                  shift-right: [w2263] -> w2260
                  shift-left: w2257 -> [w2264]
                  tunnel: string[] ["STOP", "RESET ENCODERS", "RESET YAW", "ARDUINO MODE 0"] -> [w2262] mode=indexing
                  n758 = Enqueue Element(queue=w2264, element=w2262) -> (queue out=w2263:refnum<queue>)  [unwired: 2 in, 2 out]
                }
              }
            }
          }
          frame "Task 8E: ROBOT ADJUST" {
            # ">>> Motor control cluster >>>"
            # ">>> yStepper command>>>"
            n759 = Dequeue Element(queue=w2281, timeout in ms (-1)=w2280, error in (no error)=w2279) -> (element=w2278:T10)  [unwired: 3 out]
            n760 = Subtract(x=w2276, y=150.0) -> (x-y=w2274:dbl)
            n761 = formula code="if (error >= -100 && error < -80){\n    distance = -25;\n    xSpeed = -30;\n}\n\nelse if (error >= -80 && error < -60){\n    distance = -20;\n    xSpeed = -30;\n}\n\nelse if (error >= -60 && error < -40){\n    distance = -15;\n    xSpeed = -30;\n}\n\nelse if (error >= -40 && error < -20){\n    distance = -10;\n    xSpeed = -30;\n}\n\nelse if (error >= -20 && error < -10){\n    distance = 5;\n    xSpeed = -30;\n}\n\nelse if (error >= -10 && error <= 10){\n    distance = 0;\n    xSpeed = 0;\n}\n\nelse if (error >= 20 && error < 40){\n    distance = 5;\n    xSpeed = 30;\n}\n\nelse if (error >= 40 && error < 60){\n    distance = 10;\n    xSpeed = 30;\n}\n\nelse if (error >= 60 && error < 80){\n    distance = 15;\n    xSpeed = 30;\n}\n\nelse if (error >= 80 && error < 100){\n    distance = 20;\n    xSpeed = 30;\n}\n\nelse if (error >= 100){\n    distance = 25;\n    xSpeed = 30;\n}\n\nelse {\n    distance = 0;\n    xSpeed = 0;\n}"("error"=w2274) -> ("distance"=w2269:dbl, "xSpeed"=w2271:dbl)
            "Distance to move" <- w2269
            n762 = formula code="if (target > 0){\nif (current  >= target)\noutput = 1;\n\nelse if (current != target)\noutput = 0;\n}\n\nelse if (target == 0){\nif (current == target)\noutput = 1;\n\nelse if (current != target)\noutput = 0;\n}\n\nelse if (target < 0){\nif (current <= target)\noutput = 1;\n\nelse if (current != target)\noutput = 0;\n}\n\nelse if (current != target)\noutput = 0;"("target"=w2269, "current"=w2270) -> ("output"=w2268:dbl)
            n763 = Bundle By Name(cluster=w2273, "xSpeed"=w2271) -> (w2272:T19)
            n764 = Equal?(x=w2268, y=1.0) -> (x = y?=w2265:bool)
            n765 = case shown="\"Start Task 1\", Default" w2278 {
              tunnel: [w2293 State_Type_Definitions,_for_0.26g_versions_and_later_3."True Stop" ("Enum")] -> w2285
              tunnel: [w2296 w2313] -> w2284
              tunnel: [State_Type_Definitions,_for_0.26g_versions_and_later_3."Idle" ("Enum") State_Type_Definitions,_for_0.26g_versions_and_later_3."Shutdown" ("Enum")] -> w2286
              tunnel: w2282 -> [w2292 _]
              tunnel: w2283 -> [w2288 w2310]
              tunnel: w2265 -> [w2287 _]
              frame "Start Task 1", Default {
                # ">> T: Breaks out of state loop; F: Stays in loop>>"
                # ">> Manual override >>"
                # ">> Checks if time is up>>"
                # "Stays in Task 5D until the object is detected"
                # "T: Go back to idle, F: Continue with task\""
                # ">> Manual override >>"
                n766 = case shown="True" w2287 {
                  tunnel: [w2300 w2306] -> w2296
                  tunnel: w2288 -> [w2298 w2304]
                  frame False {
                    n767 = for {
                      tunnel: string[] ["X AXIS - SLOW", "READ ENCODERS", "READ NAVX"] ("element") -> [w2301] mode=indexing
                      shift-right: [w2303] -> w2300
                      shift-left: w2298 -> [w2302]
                      n768 = Enqueue Element(queue=w2302, element=w2301) -> (queue out=w2303:refnum<queue>)  [unwired: 2 in, 2 out]
                    }
                  }
                  frame True {
                    n769 = for {
                      shift-right: [w2308] -> w2306
                      shift-left: w2304 -> [w2309]
                      tunnel: string[] ["SET TIMER 2", "STOP", "READ STEPPER VALUES", ""] -> [w2307] mode=indexing
                      n770 = Enqueue Element(queue=w2309, element=w2307) -> (queue out=w2308:refnum<queue>)  [unwired: 2 in, 2 out]
                    }
                  }
                }
                n771 = Or(x=w2287, y=w2292) -> (x .or. y?=w2294:bool)
                n772 = Select(t=State_Type_Definitions,_for_0.26g_versions_and_later_3."True Stop" ("Enum"), s=w2292, f=State_Type_Definitions,_for_0.26g_versions_and_later_3."Task 8H: ARM ADJUST" ("Enum")) -> (s? t:f=w2289:T18)
                n773 = Select(t=w2289, s=w2294, f=State_Type_Definitions,_for_0.26g_versions_and_later_3."Task 8E: ROBOT ADJUST" ("Enum")) -> (s? t:f=w2293:T18)
              }
              frame "Exit" {
                n774 = for {
                  shift-right: [w2316] -> w2313
                  shift-left: w2310 -> [w2317]
                  tunnel: string[] ["STOP", "RESET ENCODERS", "RESET YAW", "ARDUINO MODE 0"] -> [w2315] mode=indexing
                  n775 = Enqueue Element(queue=w2317, element=w2315) -> (queue out=w2316:refnum<queue>)  [unwired: 2 in, 2 out]
                }
              }
            }
          }
          frame "Task 8F: CAM BURST 2" {
            # ">>> Motor control cluster >>>"
            # ">>> yStepper command>>>"
            # ">> Manual override >>"
            n776 = Dequeue Element(queue=w2328, timeout in ms (-1)=w2327, error in (no error)=w2326) -> (element=w2325:T10)  [unwired: 3 out]
            n777 = case shown="\"Start Task 1\", Default" w2325 {
              tunnel: [w2337 State_Type_Definitions,_for_0.26g_versions_and_later_3."True Stop" ("Enum")] -> w2330
              tunnel: [w2340 w2357] -> w2323
              tunnel: [State_Type_Definitions,_for_0.26g_versions_and_later_3."Idle" ("Enum") State_Type_Definitions,_for_0.26g_versions_and_later_3."Shutdown" ("Enum")] -> w2322
              tunnel: w2324 -> [w2331 _]
              tunnel: w2329 -> [w2336 w2354]
              tunnel: w2320 -> [w2335 _]
              frame "Start Task 1", Default {
                # ">> Is time up? >>"
                # "Determines if object is in range to pick up"
                # ">> Manual override >>"
                n778 = case shown="False" w2335 {
                  tunnel: [w2344 w2350] -> w2340
                  tunnel: w2336 -> [w2342 w2348]
                  frame False {
                    n779 = for {
                      tunnel: string[] ["CAM ACQ", "START TIMER"] ("element") -> [w2345] mode=indexing
                      shift-right: [w2347] -> w2344
                      shift-left: w2342 -> [w2346]
                      n780 = Enqueue Element(queue=w2346, element=w2345) -> (queue out=w2347:refnum<queue>)  [unwired: 2 in, 2 out]
                    }
                  }
                  frame True {
                    n781 = for {
                      shift-right: [w2352] -> w2350
                      shift-left: w2348 -> [w2353]
                      tunnel: string[] ["CAM CLOSE", "PROCESS IMAGE", "SET TIMER 3"] -> [w2351] mode=indexing
                      n782 = Enqueue Element(queue=w2353, element=w2351) -> (queue out=w2352:refnum<queue>)  [unwired: 2 in, 2 out]
                    }
                  }
                }
                n783 = Or(x=w2335, y=w2331) -> (x .or. y?=w2338:bool)
                n784 = Select(t=State_Type_Definitions,_for_0.26g_versions_and_later_3."True Stop" ("Enum"), s=w2331, f=State_Type_Definitions,_for_0.26g_versions_and_later_3."Task 8G: PROCESS IMAGE 2" ("Enum")) -> (s? t:f=w2333:T18)
                n785 = Select(t=w2333, s=w2338, f=State_Type_Definitions,_for_0.26g_versions_and_later_3."Task 8F: CAM BURST 2" ("Enum")) -> (s? t:f=w2337:T18)
              }
              frame "Exit" {
                n786 = for {
                  shift-right: [w2360] -> w2357
                  shift-left: w2354 -> [w2361]
                  tunnel: string[] ["STOP", "RESET ENCODERS", "RESET YAW", "ARDUINO MODE 0"] -> [w2359] mode=indexing
                  n787 = Enqueue Element(queue=w2361, element=w2359) -> (queue out=w2360:refnum<queue>)  [unwired: 2 in, 2 out]
                }
              }
            }
          }
          frame "Task 8G: PROCESS IMAGE 2" {
            # ">>> yStepper command>>>"
            n788 = Dequeue Element(queue=w2369, timeout in ms (-1)=w2368, error in (no error)=w2367) -> (element=w2366:T10)  [unwired: 3 out]
            n789 = case shown="\"Start Task 1\", Default" w2366 {
              tunnel: [w2381 State_Type_Definitions,_for_0.26g_versions_and_later_3."True Stop" ("Enum")] -> w2373
              tunnel: [w2384 w2401] -> w2372
              tunnel: [State_Type_Definitions,_for_0.26g_versions_and_later_3."Idle" ("Enum") State_Type_Definitions,_for_0.26g_versions_and_later_3."Shutdown" ("Enum")] -> w2374
              tunnel: w2370 -> [w2380 _]
              tunnel: w2371 -> [w2376 w2398]
              tunnel: w2364 -> [w2375 _]
              frame "Start Task 1", Default {
                # ">> T: Breaks out of state loop; F: Stays in loop>>"
                # ">> Manual override >>"
                # ">> Checks if time is up>>"
                # "Stays in Task 5D until the object is detected"
                # "T: Go back to idle, F: Continue with task\""
                # ">> Manual override >>"
                n790 = case shown="False" w2375 {
                  tunnel: [w2388 w2394] -> w2384
                  tunnel: w2376 -> [w2386 w2392]
                  frame False {
                    n791 = for {
                      tunnel: string[] ["START TIMER", "PROCESS IMAGE", ""] ("element") -> [w2389] mode=indexing
                      shift-right: [w2391] -> w2388
                      shift-left: w2386 -> [w2390]
                      n792 = Enqueue Element(queue=w2390, element=w2389) -> (queue out=w2391:refnum<queue>)  [unwired: 2 in, 2 out]
                    }
                  }
                  frame True {
                    n793 = for {
                      shift-right: [w2396] -> w2394
                      shift-left: w2392 -> [w2397]
                      tunnel: string[] ["READ STEPPER VALUES", "Y STEPPER CONTROL", ""] -> [w2395] mode=indexing
                      n794 = Enqueue Element(queue=w2397, element=w2395) -> (queue out=w2396:refnum<queue>)  [unwired: 2 in, 2 out]
                    }
                  }
                }
                n795 = Or(x=w2375, y=w2380) -> (x .or. y?=w2382:bool)
                n796 = Select(t=State_Type_Definitions,_for_0.26g_versions_and_later_3."True Stop" ("Enum"), s=w2380, f=State_Type_Definitions,_for_0.26g_versions_and_later_3."Task 8H: ARM ADJUST" ("Enum")) -> (s? t:f=w2377:T18)
                n797 = Select(t=w2377, s=w2382, f=State_Type_Definitions,_for_0.26g_versions_and_later_3."Task 8G: PROCESS IMAGE 2" ("Enum")) -> (s? t:f=w2381:T18)
              }
              frame "Exit" {
                n798 = for {
                  shift-right: [w2404] -> w2401
                  shift-left: w2398 -> [w2405]
                  tunnel: string[] ["STOP", "RESET ENCODERS", "RESET YAW", "ARDUINO MODE 0"] -> [w2403] mode=indexing
                  n799 = Enqueue Element(queue=w2405, element=w2403) -> (queue out=w2404:refnum<queue>)  [unwired: 2 in, 2 out]
                }
              }
            }
          }
          frame "Task 8H: ARM ADJUST" {
            # ">>> yStepper command>>>"
            n800 = Dequeue Element(queue=w2419, timeout in ms (-1)=w2420, error in (no error)=w2421) -> (element=w2423:T10)  [unwired: 3 out]
            n801 = formula code="if (pos >= 50 && pos < 80)\ny = 40;\n\nelse if (pos >= 80 && pos < 100)\ny = 35;\n\nelse if (pos >= 100 && pos < 120)\ny = 20;\n\nelse if (pos >= 120 && pos < 140)\ny = 15;\n\nelse if (pos >= 140 && pos < 150)\ny = 10;\n\nelse if (pos >= 150 && 170)\ny = 5;\n\nelse \ny = 0;"("pos"=w2411) -> ("y"=w2414:dbl)
            n802 = To Unsigned Byte Integer(number=w2414) -> (unsigned 8bit integer=w2409:u8)
            n803 = Equal?(x=w2410, y=w2409) -> (x = y?=w2408:bool)
            n804 = case shown="\"Start Task 1\", Default" w2423 {
              tunnel: [w2430 State_Type_Definitions,_for_0.26g_versions_and_later_3."True Stop" ("Enum")] -> w2417
              tunnel: [w2433 w2450] -> w2415
              tunnel: [State_Type_Definitions,_for_0.26g_versions_and_later_3."Idle" ("Enum") State_Type_Definitions,_for_0.26g_versions_and_later_3."Shutdown" ("Enum")] -> w2416
              tunnel: w2422 -> [w2429 _]
              tunnel: w2418 -> [w2425 w2447]
              tunnel: w2408 -> [w2424 _]
              frame "Start Task 1", Default {
                # ">> T: Breaks out of state loop; F: Stays in loop>>"
                # ">> Manual override >>"
                # ">> Checks if time is up>>"
                # "Stays in Task 5D until the object is detected"
                # "T: Go back to idle, F: Continue with task\""
                # ">> Manual override >>"
                n805 = case shown="False" w2424 {
                  tunnel: [w2437 w2443] -> w2433
                  tunnel: w2425 -> [w2435 w2441]
                  frame False {
                    n806 = for {
                      tunnel: string[] ["READ STEPPER VALUES", "Y STEPPER CONTROL", ""] ("element") -> [w2438] mode=indexing
                      shift-right: [w2440] -> w2437
                      shift-left: w2435 -> [w2439]
                      n807 = Enqueue Element(queue=w2439, element=w2438) -> (queue out=w2440:refnum<queue>)  [unwired: 2 in, 2 out]
                    }
                  }
                  frame True {
                    n808 = for {
                      shift-right: [w2445] -> w2443
                      shift-left: w2441 -> [w2446]
                      tunnel: string[] ["DISPOSE BUFFERS", "READ STEPPER VALUES", ""] -> [w2444] mode=indexing
                      n809 = Enqueue Element(queue=w2446, element=w2444) -> (queue out=w2445:refnum<queue>)  [unwired: 2 in, 2 out]
                    }
                  }
                }
                n810 = Or(x=w2424, y=w2429) -> (x .or. y?=w2431:bool)
                n811 = Select(t=State_Type_Definitions,_for_0.26g_versions_and_later_3."True Stop" ("Enum"), s=w2429, f=State_Type_Definitions,_for_0.26g_versions_and_later_3."Task 8I: ARM GRAB HEIGHT" ("Enum")) -> (s? t:f=w2426:T18)
                n812 = Select(t=w2426, s=w2431, f=State_Type_Definitions,_for_0.26g_versions_and_later_3."Task 8H: ARM ADJUST" ("Enum")) -> (s? t:f=w2430:T18)
              }
              frame "Exit" {
                n813 = for {
                  shift-right: [w2453] -> w2450
                  shift-left: w2447 -> [w2454]
                  tunnel: string[] ["STOP", "RESET ENCODERS", "RESET YAW", "ARDUINO MODE 0"] -> [w2452] mode=indexing
                  n814 = Enqueue Element(queue=w2454, element=w2452) -> (queue out=w2453:refnum<queue>)  [unwired: 2 in, 2 out]
                }
              }
            }
            n815 = Bundle By Name(cluster=w2413, "yStepper desired"=w2409) -> (w2412:T20)
          }
          frame "Task 8I: ARM GRAB HEIGHT" {
            # ">>> Motor control cluster >>>"
            # ">>> yStepper command>>>"
            # ">> Manual override >>"
            n816 = Dequeue Element(queue=w2465, timeout in ms (-1)=w2464, error in (no error)=w2466) -> (element=w2463:T10)  [unwired: 3 out]
            n817 = Equal?(x=w2462, y=u8 1) -> (x = y?=w2460:bool)
            n818 = case shown="\"Start Task 1\", Default" w2463 {
              tunnel: [w2476 State_Type_Definitions,_for_0.26g_versions_and_later_3."True Stop" ("Enum")] -> w2467
              tunnel: [w2479 w2496] -> w2468
              tunnel: [State_Type_Definitions,_for_0.26g_versions_and_later_3."Idle" ("Enum") State_Type_Definitions,_for_0.26g_versions_and_later_3."Shutdown" ("Enum")] -> w2469
              tunnel: w2460 -> [w2475 _]
              tunnel: w2459 -> [w2474 _]
              tunnel: w2458 -> [w2470 w2493]
              frame "Start Task 1", Default {
                # "Stays in Task 5F until stepper reaches desired \nheight"
                # "T: Go back to idle, F: Continue with task\""
                # ">> Manual override >>"
                n819 = case shown="True" w2475 {
                  tunnel: [w2483 w2489] -> w2479
                  tunnel: w2470 -> [w2481 w2487]
                  frame False {
                    n820 = for {
                      tunnel: string[] ["Z STEPPER GRAB HEIGHT", "READ STEPPER VALUES"] ("element") -> [w2484] mode=indexing
                      shift-right: [w2486] -> w2483
                      shift-left: w2481 -> [w2485]
                      n821 = Enqueue Element(queue=w2485, element=w2484) -> (queue out=w2486:refnum<queue>)  [unwired: 2 in, 2 out]
                    }
                  }
                  frame True {
                    n822 = for {
                      shift-right: [w2491] -> w2489
                      shift-left: w2487 -> [w2492]
                      tunnel: string[] ["SET TIMER 2", "CLOSE CLAW", ""] -> [w2490] mode=indexing
                      n823 = Enqueue Element(queue=w2492, element=w2490) -> (queue out=w2491:refnum<queue>)  [unwired: 2 in, 2 out]
                    }
                  }
                }
                n824 = Or(x=w2475, y=w2474) -> (x .or. y?=w2477:bool)
                n825 = Select(t=State_Type_Definitions,_for_0.26g_versions_and_later_3."True Stop" ("Enum"), s=w2474, f=State_Type_Definitions,_for_0.26g_versions_and_later_3."Task 8J: CLOSE CLAW" ("Enum")) -> (s? t:f=w2471:T18)
                n826 = Select(t=w2471, s=w2477, f=State_Type_Definitions,_for_0.26g_versions_and_later_3."Task 8I: ARM GRAB HEIGHT" ("Enum")) -> (s? t:f=w2476:T18)
              }
              frame "Exit" {
                n827 = for {
                  shift-right: [w2499] -> w2496
                  shift-left: w2493 -> [w2500]
                  tunnel: string[] ["STOP", "RESET ENCODERS", "RESET YAW", "ARDUINO MODE 0"] -> [w2498] mode=indexing
                  n828 = Enqueue Element(queue=w2500, element=w2498) -> (queue out=w2499:refnum<queue>)  [unwired: 2 in, 2 out]
                }
              }
            }
          }
          frame "Task 8J: CLOSE CLAW" {
            # ">>> yStepper command>>>"
            # ">> Manual override >>"
            n829 = Dequeue Element(queue=w2511, timeout in ms (-1)=w2510, error in (no error)=w2509) -> (element=w2508:T10)  [unwired: 3 out]
            n830 = case shown="\"Start Task 1\", Default" w2508 {
              tunnel: [w2520 State_Type_Definitions,_for_0.26g_versions_and_later_3."True Stop" ("Enum")] -> w2513
              tunnel: [w2523 w2540] -> w2506
              tunnel: [State_Type_Definitions,_for_0.26g_versions_and_later_3."Idle" ("Enum") State_Type_Definitions,_for_0.26g_versions_and_later_3."Shutdown" ("Enum")] -> w2505
              tunnel: w2507 -> [w2514 _]
              tunnel: w2512 -> [w2519 w2537]
              tunnel: w2503 -> [w2518 _]
              frame "Start Task 1", Default {
                # ">> Is time up? >>"
                # "Determines if object is in range to pick up"
                # ">> Manual override >>"
                n831 = case shown="True" w2518 {
                  tunnel: [w2527 w2533] -> w2523
                  tunnel: w2519 -> [w2525 w2531]
                  frame False {
                    n832 = for {
                      tunnel: string[] ["CLOSE CLAW", "START TIMER"] ("element") -> [w2528] mode=indexing
                      shift-right: [w2530] -> w2527
                      shift-left: w2525 -> [w2529]
                      n833 = Enqueue Element(queue=w2529, element=w2528) -> (queue out=w2530:refnum<queue>)  [unwired: 2 in, 2 out]
                    }
                  }
                  frame True {
                    n834 = for {
                      shift-right: [w2535] -> w2533
                      shift-left: w2531 -> [w2536]
                      tunnel: string[] ["READ STEPPER VALUES", "", ""] -> [w2534] mode=indexing
                      n835 = Enqueue Element(queue=w2536, element=w2534) -> (queue out=w2535:refnum<queue>)  [unwired: 2 in, 2 out]
                    }
                  }
                }
                n836 = Or(x=w2518, y=w2514) -> (x .or. y?=w2521:bool)
                n837 = Select(t=State_Type_Definitions,_for_0.26g_versions_and_later_3."True Stop" ("Enum"), s=w2514, f=State_Type_Definitions,_for_0.26g_versions_and_later_3."Task 8K: RAISE MY SWORD" ("Enum")) -> (s? t:f=w2516:T18)
                n838 = Select(t=w2516, s=w2521, f=State_Type_Definitions,_for_0.26g_versions_and_later_3."Task 8J: CLOSE CLAW" ("Enum")) -> (s? t:f=w2520:T18)
              }
              frame "Exit" {
                n839 = for {
                  shift-right: [w2543] -> w2540
                  shift-left: w2537 -> [w2544]
                  tunnel: string[] ["STOP", "RESET ENCODERS", "RESET YAW", "ARDUINO MODE 0"] -> [w2542] mode=indexing
                  n840 = Enqueue Element(queue=w2544, element=w2542) -> (queue out=w2543:refnum<queue>)  [unwired: 2 in, 2 out]
                }
              }
            }
          }
          frame "Task 8K: RAISE MY SWORD" {
            # ">>> yStepper command>>>"
            # ">> Manual override >>"
            n841 = Dequeue Element(queue=w2555, timeout in ms (-1)=w2554, error in (no error)=w2556) -> (element=w2553:T10)  [unwired: 3 out]
            n842 = Equal?(x=w2552, y=u8 60) -> (x = y?=w2550:bool)
            n843 = case shown="\"Start Task 1\", Default" w2553 {
              tunnel: [w2566 State_Type_Definitions,_for_0.26g_versions_and_later_3."True Stop" ("Enum")] -> w2557
              tunnel: [w2569 w2586] -> w2558
              tunnel: [State_Type_Definitions,_for_0.26g_versions_and_later_3."Idle" ("Enum") State_Type_Definitions,_for_0.26g_versions_and_later_3."Shutdown" ("Enum")] -> w2559
              tunnel: w2550 -> [w2565 _]
              tunnel: w2549 -> [w2564 _]
              tunnel: w2548 -> [w2560 w2583]
              frame "Start Task 1", Default {
                # "Stays in Task 5_A until stepper reaches desired \nheight"
                # "T: Go back to idle, F: Continue with task\""
                # ">> Manual override >>"
                n844 = case shown="True" w2565 {
                  tunnel: [w2573 w2579] -> w2569
                  tunnel: w2560 -> [w2571 w2577]
                  frame False {
                    n845 = for {
                      tunnel: string[] ["Z STEPPER CAM HEIGHT", "READ STEPPER VALUES"] ("element") -> [w2574] mode=indexing
                      shift-right: [w2576] -> w2573
                      shift-left: w2571 -> [w2575]
                      n846 = Enqueue Element(queue=w2575, element=w2574) -> (queue out=w2576:refnum<queue>)  [unwired: 2 in, 2 out]
                    }
                  }
                  frame True {
                    n847 = for {
                      shift-right: [w2581] -> w2579
                      shift-left: w2577 -> [w2582]
                      tunnel: string[] ["CAM CLOSE", "DISPOSE CAM BUFFERS", "DISPOSE PROC BUFFERS", "RESET ENCODERS"] -> [w2580] mode=indexing
                      n848 = Enqueue Element(queue=w2582, element=w2580) -> (queue out=w2581:refnum<queue>)  [unwired: 2 in, 2 out]
                    }
                  }
                }
                n849 = Or(x=w2565, y=w2564) -> (x .or. y?=w2567:bool)
                n850 = Select(t=State_Type_Definitions,_for_0.26g_versions_and_later_3."True Stop" ("Enum"), s=w2564, f=State_Type_Definitions,_for_0.26g_versions_and_later_3."True Stop" ("Enum")) -> (s? t:f=w2561:T18)
                n851 = Select(t=w2561, s=w2567, f=State_Type_Definitions,_for_0.26g_versions_and_later_3."Task 8K: RAISE MY SWORD" ("Enum")) -> (s? t:f=w2566:T18)
              }
              frame "Exit" {
                n852 = for {
                  shift-right: [w2589] -> w2586
                  shift-left: w2583 -> [w2590]
                  tunnel: string[] ["STOP", "RESET ENCODERS", "RESET YAW", "ARDUINO MODE 0"] -> [w2588] mode=indexing
                  n853 = Enqueue Element(queue=w2590, element=w2588) -> (queue out=w2589:refnum<queue>)  [unwired: 2 in, 2 out]
                }
              }
            }
          }
          frame "Task 9A: Raise Arm" {
            # ">>> Motor control cluster >>>"
            # ">> Stepper height reeached >>"
            # ">>> yStepper command>>>"
            # ">> Manual override >>"
            n854 = Dequeue Element(queue=w2603, timeout in ms (-1)=w2598, error in (no error)=w2602) -> (element=w2605:T10)  [unwired: 3 out]
            n855 = Equal?(x=w2600, y=u8 50) -> (x = y?=w2591:bool)
            n856 = case shown="\"Start Task 1\", Default" w2605 {
              tunnel: [w2616 State_Type_Definitions,_for_0.26g_versions_and_later_3."True Stop" ("Enum")] -> w2596
              tunnel: [w2614 w2631] -> w2595
              tunnel: w2599 -> [w2613 _]
              tunnel: w2601 -> [w2607 _]
              tunnel: [State_Type_Definitions,_for_0.26g_versions_and_later_3."Idle" ("Enum") State_Type_Definitions,_for_0.26g_versions_and_later_3."Shutdown" ("Enum")] -> w2597
              tunnel: w2591 -> [w2606 _]
              frame "Start Task 1", Default {
                # ">> WIill proceed to part ii if not manual override >>"
                # ">>If ENABLE or Trigger is set to true>>"
                n857 = Or(x=w2606, y=w2607) -> (x .or. y?=w2608:bool)
                n858 = case shown="False" w2606 {
                  tunnel: [w2619 w2625] -> w2614
                  tunnel: w2613 -> [w2618 w2624]
                  frame False {
                    n859 = for {
                      shift-right: [w2621] -> w2619
                      shift-left: w2618 -> [w2622]
                      tunnel: string[] ["Z STEPPER BOX HEIGHT", "READ STEPPER VALUES"] ("element") -> [w2620] mode=indexing
                      n860 = Enqueue Element(queue=w2622, element=w2620) -> (queue out=w2621:refnum<queue>)  [unwired: 2 in, 2 out]
                    }
                  }
                  frame True {
                    n861 = for {
                      shift-right: [w2627] -> w2625
                      shift-left: w2624 -> [w2628]
                      tunnel: string[] ["READ NAVX", "RESET FLAGS", "RESET YAW", "", "", ""] -> [w2626] mode=indexing
                      n862 = Enqueue Element(queue=w2628, element=w2626) -> (queue out=w2627:refnum<queue>)  [unwired: 2 in, 2 out]
                    }
                  }
                }
                n863 = Select(t=State_Type_Definitions,_for_0.26g_versions_and_later_3."True Stop" ("Enum"), s=w2607, f=State_Type_Definitions,_for_0.26g_versions_and_later_3."Task 9B: Rotate to Angle" ("Enum")) -> (s? t:f=w2610:T18)
                n864 = Select(t=w2610, s=w2608, f=State_Type_Definitions,_for_0.26g_versions_and_later_3."Task 9A: Raise Arm" ("Enum")) -> (s? t:f=w2616:T18)
              }
              frame "Exit" {
                n865 = for {
                  shift-right: [w2634] -> w2631
                  shift-left: _ -> [w2635]
                  tunnel: string[] ["STOP", "RESET ENCODERS", "RESET YAW", ""] -> [w2633] mode=indexing
                  n866 = Enqueue Element(queue=w2635, element=w2633) -> (queue out=w2634:refnum<queue>)  [unwired: 2 in, 2 out]
                }
              }
            }
          }
          frame "Task 9B: Rotate to Angle" {
            # ">>> Motor control cluster >>>"
            # ">>> yStepper command>>>"
            n867 = Dequeue Element(queue=w2649, timeout in ms (-1)=w2648, error in (no error)=w2647) -> (element=w2651:T10)  [unwired: 3 out]
            n868 = In Range and Coerce(upper limit=65.0, x=w2641, lower limit=58.0) -> (In Range?=w2636:bool)  [unwired: 1 out]
            n869 = case shown="\"Start Task 1\", Default" w2651 {
              tunnel: w2642 -> [w2654 _]
              tunnel: [w2662 State_Type_Definitions,_for_0.26g_versions_and_later_3."True Stop" ("Enum")] -> w2644
              tunnel: w2650 -> [w2660 w2678]
              tunnel: [w2659 w2677] -> w2643
              tunnel: [State_Type_Definitions,_for_0.26g_versions_and_later_3."Idle" ("Enum") State_Type_Definitions,_for_0.26g_versions_and_later_3."Shutdown" ("Enum")] -> w2645
              tunnel: w2636 -> [w2652 _]
              frame "Start Task 1", Default {
                n870 = Or(x=w2652, y=w2654) -> (x .or. y?=w2653:bool)
                n871 = case shown="False" w2652 {
                  tunnel: w2660 -> [w2665 w2671]
                  tunnel: [w2664 w2669] -> w2659
                  frame False {
                    n872 = for {
                      shift-right: [w2667] -> w2664
                      shift-left: w2665 -> [w2668]
                      tunnel: string[] ["READ NAVX", "R-CW", ""] ("element") -> [w2666] mode=indexing
                      n873 = Enqueue Element(queue=w2668, element=w2666) -> (queue out=w2667:refnum<queue>)  [unwired: 2 in, 2 out]
                    }
                  }
                  frame True {
                    n874 = for {
                      shift-right: [w2673] -> w2669
                      shift-left: w2671 -> [w2674]
                      tunnel: string[] ["STOP", "RESET ENCODERS", "RESET YAW", "", ""] -> [w2672] mode=indexing
                      n875 = Enqueue Element(queue=w2674, element=w2672) -> (queue out=w2673:refnum<queue>)  [unwired: 2 in, 2 out]
                    }
                  }
                }
                n876 = Select(t=State_Type_Definitions,_for_0.26g_versions_and_later_3."True Stop" ("Enum"), s=w2654, f=State_Type_Definitions,_for_0.26g_versions_and_later_3."Task 9C: Detect Box") -> (s? t:f=w2656:T18)
                n877 = Select(t=w2656, s=w2653, f=State_Type_Definitions,_for_0.26g_versions_and_later_3."Task 9B: Rotate to Angle" ("Enum")) -> (s? t:f=w2662:T18)
              }
              frame "Exit" {
                n878 = for {
                  shift-right: [w2681] -> w2677
                  shift-left: w2678 -> [w2682]
                  tunnel: string[] ["STOP", "RESET ENCODERS", "RESET YAW", ""] -> [w2680] mode=indexing
                  n879 = Enqueue Element(queue=w2682, element=w2680) -> (queue out=w2681:refnum<queue>)  [unwired: 2 in, 2 out]
                }
              }
            }
          }
          frame "Task 9C: Detect Box" {
            # ">>> Motor control cluster >>>"
            # ">>Line Detected>>"
            # ">>Action Queue>>"
            # ">>> yStepper command>>>"
            n880 = Dequeue Element(queue=w2694, timeout in ms (-1)=w2693, error in (no error)=w2692) -> (element=w2695:T10)  [unwired: 3 out]
            n881 = case shown="\"Start Task 1\", Default" w2695 {
              tunnel: w2690 -> [w2696 _]
              tunnel: [w2706 State_Type_Definitions,_for_0.26g_versions_and_later_3."True Stop" ("Enum")] -> w2687
              tunnel: w2691 -> [w2704 w2722]
              tunnel: [w2703 w2721] -> w2686
              tunnel: [State_Type_Definitions,_for_0.26g_versions_and_later_3."Idle" ("Enum") State_Type_Definitions,_for_0.26g_versions_and_later_3."Shutdown" ("Enum")] -> w2689
              tunnel: w2683 -> [w2697 _]
              frame "Start Task 1", Default {
                n882 = Or(x=w2696, y=w2697) -> (x .or. y?=w2698:bool)
                n883 = case shown="False" w2697 {
                  tunnel: w2704 -> [w2709 w2715]
                  tunnel: [w2708 w2713] -> w2703
                  frame False {
                    n884 = for {
                      shift-right: [w2711] -> w2708
                      shift-left: w2709 -> [w2712]
                      tunnel: string[] ["READ IR", "READ LINE SENSOR", "FORWARD - IR ASSIST"] ("element") -> [w2710] mode=indexing
                      n885 = Enqueue Element(queue=w2712, element=w2710) -> (queue out=w2711:refnum<queue>)  [unwired: 2 in, 2 out]
                    }
                  }
                  frame True {
                    n886 = for {
                      shift-right: [w2717] -> w2713
                      shift-left: w2715 -> [w2718]
                      tunnel: string[] ["STOP", "RESET ENCODERS", "RESET YAW", "RESET FLAGS"] -> [w2716] mode=indexing
                      n887 = Enqueue Element(queue=w2718, element=w2716) -> (queue out=w2717:refnum<queue>)  [unwired: 2 in, 2 out]
                    }
                  }
                }
                n888 = Select(t=State_Type_Definitions,_for_0.26g_versions_and_later_3."True Stop" ("Enum"), s=w2696, f=State_Type_Definitions,_for_0.26g_versions_and_later_3."Task 9D: MOVE FORWARD") -> (s? t:f=w2700:T18)
                n889 = Select(t=w2700, s=w2698, f=State_Type_Definitions,_for_0.26g_versions_and_later_3."Task 9C: Detect Box" ("Enum")) -> (s? t:f=w2706:T18)
              }
              frame "Exit" {
                n890 = for {
                  shift-right: [w2725] -> w2721
                  shift-left: w2722 -> [w2726]
                  tunnel: string[] ["STOP", "RESET ENCODERS", "RESET YAW", ""] -> [w2724] mode=indexing
                  n891 = Enqueue Element(queue=w2726, element=w2724) -> (queue out=w2725:refnum<queue>)  [unwired: 2 in, 2 out]
                }
              }
            }
          }
          frame "Task 9D: MOVE FORWARD" {
            (unwired) 50.0 ("y")
            # ">> Item Selection Bias >>"
            # ">> Wall detected >>"
            # ">> Manual override >>"
            # ">>Table Detected>>"
            # ">>> Motor control cluster >>>"
            # ">>Table or wall detectected>>"
            # ">>Action Queue>>"
            # ">>> yStepper command>>>"
            n892 = Dequeue Element(queue=w2744, timeout in ms (-1)=w2743, error in (no error)=w2742) -> (element=w2745:T10)  [unwired: 3 out]
            n893 = Less Or Equal?(x=w2733, y=20.0) -> (x <= y?=w2728:bool)
            n894 = Less?(x=w2731, y=20.0) -> (x < y?=w2729:bool)
            n895 = Or(x=w2728, y=w2729) -> (x .or. y?=w2727:bool)
            n896 = case shown="\"Start Task 1\", Default" w2745 {
              tunnel: w2740 -> [w2746 _]
              tunnel: [w2756 State_Type_Definitions,_for_0.26g_versions_and_later_3."True Stop" ("Enum")] -> w2737
              tunnel: w2741 -> [w2754 w2772]
              tunnel: [w2753 w2771] -> w2736
              tunnel: [State_Type_Definitions,_for_0.26g_versions_and_later_3."Idle" ("Enum") State_Type_Definitions,_for_0.26g_versions_and_later_3."Shutdown" ("Enum")] -> w2739
              tunnel: w2727 -> [w2747 _]
              frame "Start Task 1", Default {
                n897 = Or(x=w2746, y=w2747) -> (x .or. y?=w2748:bool)
                n898 = case shown="True" w2747 {
                  tunnel: w2754 -> [w2759 w2765]
                  tunnel: [w2758 w2763] -> w2753
                  frame False {
                    n899 = for {
                      shift-right: [w2761] -> w2758
                      shift-left: w2759 -> [w2762]
                      tunnel: string[] ["READ IR", "FORWARD - IR ASSIST", ""] ("element") -> [w2760] mode=indexing
                      n900 = Enqueue Element(queue=w2762, element=w2760) -> (queue out=w2761:refnum<queue>)  [unwired: 2 in, 2 out]
                    }
                  }
                  frame True {
                    n901 = for {
                      shift-right: [w2767] -> w2763
                      shift-left: w2765 -> [w2768]
                      tunnel: string[] ["STOP", "RESET ENCODERS", "RESET YAW", "RESET FLAGS"] -> [w2766] mode=indexing
                      n902 = Enqueue Element(queue=w2768, element=w2766) -> (queue out=w2767:refnum<queue>)  [unwired: 2 in, 2 out]
                    }
                  }
                }
                n903 = Select(t=State_Type_Definitions,_for_0.26g_versions_and_later_3."True Stop" ("Enum"), s=w2746, f=State_Type_Definitions,_for_0.26g_versions_and_later_3."Task 9E: MOVE LEFT") -> (s? t:f=w2750:T18)
                n904 = Select(t=w2750, s=w2748, f=State_Type_Definitions,_for_0.26g_versions_and_later_3."Task 9D: MOVE FORWARD" ("Enum")) -> (s? t:f=w2756:T18)
              }
              frame "Exit" {
                n905 = for {
                  shift-right: [w2775] -> w2771
                  shift-left: w2772 -> [w2776]
                  tunnel: string[] ["STOP", "RESET ENCODERS", "RESET YAW", ""] -> [w2774] mode=indexing
                  n906 = Enqueue Element(queue=w2776, element=w2774) -> (queue out=w2775:refnum<queue>)  [unwired: 2 in, 2 out]
                }
              }
            }
          }
          frame "Task 9E: MOVE LEFT" {
            # ">> Item Selection Bias >>"
            # ">> Line detected? >>"
            # ">> Manual override >>"
            # ">>> Motor control cluster >>>"
            # ">>Action Queue>>"
            # ">>> yStepper command>>>"
            n907 = Dequeue Element(queue=w2788, timeout in ms (-1)=w2787, error in (no error)=w2786) -> (element=w2789:T10)  [unwired: 3 out]
            n908 = case shown="\"Start Task 1\", Default" w2789 {
              tunnel: w2784 -> [w2790 _]
              tunnel: [w2800 State_Type_Definitions,_for_0.26g_versions_and_later_3."True Stop" ("Enum")] -> w2781
              tunnel: w2785 -> [w2798 w2816]
              tunnel: [w2797 w2815] -> w2780
              tunnel: [State_Type_Definitions,_for_0.26g_versions_and_later_3."Idle" ("Enum") State_Type_Definitions,_for_0.26g_versions_and_later_3."Shutdown" ("Enum")] -> w2783
              tunnel: w2777 -> [w2791 _]
              frame "Start Task 1", Default {
                n909 = Or(x=w2790, y=w2791) -> (x .or. y?=w2792:bool)
                n910 = case shown="True" w2791 {
                  tunnel: w2798 -> [w2803 w2809]
                  tunnel: [w2802 w2807] -> w2797
                  frame False {
                    n911 = for {
                      shift-right: [w2805] -> w2802
                      shift-left: w2803 -> [w2806]
                      tunnel: string[] ["LEFT", "READ NAVX", "READ LINE SENSOR", ""] ("element") -> [w2804] mode=indexing
                      n912 = Enqueue Element(queue=w2806, element=w2804) -> (queue out=w2805:refnum<queue>)  [unwired: 2 in, 2 out]
                    }
                  }
                  frame True {
                    n913 = for {
                      shift-right: [w2811] -> w2807
                      shift-left: w2809 -> [w2812]
                      tunnel: string[] ["STOP", "RESET ENCODERS", "RESET YAW", "BOX COLOUR", "", ""] -> [w2810] mode=indexing
                      n914 = Enqueue Element(queue=w2812, element=w2810) -> (queue out=w2811:refnum<queue>)  [unwired: 2 in, 2 out]
                    }
                  }
                }
                n915 = Select(t=State_Type_Definitions,_for_0.26g_versions_and_later_3."True Stop" ("Enum"), s=w2790, f=State_Type_Definitions,_for_0.26g_versions_and_later_3."Task 9F: SCAN BOX") -> (s? t:f=w2794:T18)
                n916 = Select(t=w2794, s=w2792, f=State_Type_Definitions,_for_0.26g_versions_and_later_3."Task 9E: MOVE LEFT" ("Enum")) -> (s? t:f=w2800:T18)
              }
              frame "Exit" {
                n917 = for {
                  shift-right: [w2819] -> w2815
                  shift-left: w2816 -> [w2820]
                  tunnel: string[] ["STOP", "RESET ENCODERS", "RESET YAW", ""] -> [w2818] mode=indexing
                  n918 = Enqueue Element(queue=w2820, element=w2818) -> (queue out=w2819:refnum<queue>)  [unwired: 2 in, 2 out]
                }
              }
            }
          }
          frame "Task 9F: SCAN BOX" {
            # ">>> Motor control cluster >>>"
            # ">>Colour detection >>"
            # ">>> yStepper command>>>"
            # ">> Manual override >>"
            n919 = Dequeue Element(queue=w2837, timeout in ms (-1)=w2835, error in (no error)=w2836) -> (element=w2830:T10)  [unwired: 3 out]
            n920 = call "Box Colour FGV.vi"("Init/R/W State"=Box_Colour_FGV_States."Read") -> ("Colour to detect (output)"=w2823:T2)  [unwired: 9 in, 1 out]
            n921 = Equal?(x=w2824, y=w2823) -> (x = y?=w2822:bool)
            n922 = case shown="\"Start Task 1\", Default" w2830 {
              tunnel: [w2850 State_Type_Definitions,_for_0.26g_versions_and_later_3."True Stop" ("Enum")] -> w2827
              tunnel: [w2848 w2865] -> w2828
              tunnel: w2829 -> [w2847 _]
              tunnel: w2831 -> [w2840 _]
              tunnel: [State_Type_Definitions,_for_0.26g_versions_and_later_3."Idle" ("Enum") State_Type_Definitions,_for_0.26g_versions_and_later_3."Shutdown" ("Enum")] -> w2826
              tunnel: w2821 -> [w2841 _]
              tunnel: w2822 -> [w2839 _]
              frame "Start Task 1", Default {
                # ">> Will stop either due to manual override or is same box colour >>"
                # ">> WIill proceed to part ii if not manual override >>"
                # ">>If ENABLE or Trigger is set to true>>"
                n923 = Or(x=w2841, y=w2840) -> (x .or. y?=w2842:bool)
                n924 = case shown="True" w2841 {
                  tunnel: [w2853 w2859] -> w2848
                  tunnel: w2847 -> [w2852 w2858]
                  frame False {
                    n925 = for {
                      shift-right: [w2855] -> w2853
                      shift-left: w2852 -> [w2856]
                      tunnel: string[] ["", ""] ("element") -> [w2854] mode=indexing
                      n926 = Enqueue Element(queue=w2856, element=w2854) -> (queue out=w2855:refnum<queue>)  [unwired: 2 in, 2 out]
                    }
                  }
                  frame True {
                    n927 = for {
                      shift-right: [w2861] -> w2859
                      shift-left: w2858 -> [w2862]
                      tunnel: string[] ["RESET ENCODER", "RESET FLAGS", "RESET YAW", "", "", ""] -> [w2860] mode=indexing
                      n928 = Enqueue Element(queue=w2862, element=w2860) -> (queue out=w2861:refnum<queue>)  [unwired: 2 in, 2 out]
                    }
                  }
                }
                n929 = Or(x=w2840, y=w2839) -> (x .or. y?=w2838:bool)
                n930 = Select(t=State_Type_Definitions,_for_0.26g_versions_and_later_3."True Stop" ("Enum"), s=w2838, f=State_Type_Definitions,_for_0.26g_versions_and_later_3."Task 9G: MOVE RIGHT" ("Enum")) -> (s? t:f=w2844:T18)
                n931 = Select(t=w2844, s=w2842, f=State_Type_Definitions,_for_0.26g_versions_and_later_3."Task 9F: SCAN BOX" ("Enum")) -> (s? t:f=w2850:T18)
              }
              frame "Exit" {
                n932 = for {
                  shift-right: [w2868] -> w2865
                  shift-left: _ -> [w2869]
                  tunnel: string[] ["STOP", "RESET ENCODERS", "RESET YAW", ""] -> [w2867] mode=indexing
                  n933 = Enqueue Element(queue=w2869, element=w2867) -> (queue out=w2868:refnum<queue>)  [unwired: 2 in, 2 out]
                }
              }
            }
          }
          frame "Task 9G: MOVE RIGHT" {
            # ">>> Motor control cluster >>>"
            # ">>> yStepper command>>>"
            n934 = Dequeue Element(queue=w2881, timeout in ms (-1)=w2880, error in (no error)=w2879) -> (element=w2886:T10)  [unwired: 3 out]
            n935 = Greater?(x=w2871, y=50.0) -> (0:w2874:bool)
            n936 = And(x=w2872, y=w2874) -> (x .and. y?=w2870:bool)
            n937 = case shown="\"Start Task 1\", Default" w2886 {
              tunnel: w2870 -> [w2889 _]
              tunnel: [w2896 State_Type_Definitions,_for_0.26g_versions_and_later_3."True Stop" ("Enum")] -> w2885
              tunnel: w2878 -> [w2888 _]
              tunnel: w2882 -> [w2895 w2912]
              tunnel: [w2894 w2913] -> w2884
              tunnel: [State_Type_Definitions,_for_0.26g_versions_and_later_3."Idle" ("Enum") State_Type_Definitions,_for_0.26g_versions_and_later_3."Shutdown" ("Enum")] -> w2883
              frame "Start Task 1", Default {
                n938 = case shown="True" w2889 {
                  tunnel: w2895 -> [w2899 w2906]
                  tunnel: [w2900 w2905] -> w2894
                  frame False {
                    n939 = for {
                      tunnel: string[] ["READ LINE SENSOR", "READ NAVX", "RIGHT", "READ ENCODERS"] ("element") -> [w2901] mode=indexing
                      shift-right: [w2903] -> w2900
                      shift-left: w2899 -> [w2902]
                      n940 = Enqueue Element(queue=w2902, element=w2901) -> (queue out=w2903:refnum<queue>)  [unwired: 2 in, 2 out]
                    }
                  }
                  frame True {
                    n941 = for {
                      shift-right: [w2908] -> w2905
                      shift-left: w2906 -> [w2909]
                      tunnel: string[] ["RESET ENCODERS", "RESET YAW", "RESET FLAGS", "STOP", "BOX COLOUR"] -> [w2907] mode=indexing
                      n942 = Enqueue Element(queue=w2909, element=w2907) -> (queue out=w2908:refnum<queue>)  [unwired: 2 in, 2 out]
                    }
                  }
                }
                n943 = Or(x=w2889, y=w2888) -> (x .or. y?=w2887:bool)
                n944 = Select(t=State_Type_Definitions,_for_0.26g_versions_and_later_3."True Stop" ("Enum"), s=w2888, f=State_Type_Definitions,_for_0.26g_versions_and_later_3."Task 9H: SCAN BOX 2" ("Enum")) -> (s? t:f=w2890:T18)
                n945 = Select(t=w2890, s=w2887, f=State_Type_Definitions,_for_0.26g_versions_and_later_3."Task 9G: MOVE RIGHT" ("Enum")) -> (s? t:f=w2896:T18)
              }
              frame "Exit" {
                n946 = for {
                  shift-right: [w2916] -> w2913
                  shift-left: w2912 -> [w2917]
                  tunnel: string[] ["STOP", "RESET ENCODERS", "RESET YAW", "ARDUINO MODE 0"] -> [w2915] mode=indexing
                  n947 = Enqueue Element(queue=w2917, element=w2915) -> (queue out=w2916:refnum<queue>)  [unwired: 2 in, 2 out]
                }
              }
            }
          }
          frame "Task 9H: SCAN BOX 2" {
            # ">> Item Selection Bias >>"
            # ">>> Motor control cluster >>>"
            # ">>> yStepper command>>>"
            n948 = Dequeue Element(queue=w2927, timeout in ms (-1)=w2928, error in (no error)=w2929) -> (element=w2931:T10)  [unwired: 3 out]
            n949 = call "Box Colour FGV.vi"("Init/R/W State"=Box_Colour_FGV_States."Read") -> ("Colour to detect (output)"=w2921:T2)  [unwired: 9 in, 1 out]
            n950 = Equal?(x=w2920, y=w2921) -> (x = y?=w2919:bool)
            n951 = case shown="\"Start Task 1\", Default" w2931 {
              tunnel: w2918 -> [w2939 _]
              tunnel: [w2946 State_Type_Definitions,_for_0.26g_versions_and_later_3."True Stop" ("Enum")] -> w2924
              tunnel: w2930 -> [w2936 _]
              tunnel: w2926 -> [w2945 w2962]
              tunnel: [w2944 w2963] -> w2925
              tunnel: [State_Type_Definitions,_for_0.26g_versions_and_later_3."Idle" ("Enum") State_Type_Definitions,_for_0.26g_versions_and_later_3."Shutdown" ("Enum")] -> w2923
              tunnel: w2919 -> [w2937 _]
              frame "Start Task 1", Default {
                n952 = Or(x=w2939, y=w2936) -> (x .or. y?=w2938:bool)
                n953 = Or(x=w2937, y=w2936) -> (x .or. y?=w2935:bool)
                n954 = case shown="True" w2939 {
                  tunnel: w2945 -> [w2949 w2956]
                  tunnel: [w2950 w2955] -> w2944
                  frame False {
                    n955 = for {
                      tunnel: string[] ["", "", "", ""] ("element") -> [w2951] mode=indexing
                      shift-right: [w2953] -> w2950
                      shift-left: w2949 -> [w2952]
                      n956 = Enqueue Element(queue=w2952, element=w2951) -> (queue out=w2953:refnum<queue>)  [unwired: 2 in, 2 out]
                    }
                  }
                  frame True {
                    n957 = for {
                      shift-right: [w2958] -> w2955
                      shift-left: w2956 -> [w2959]
                      tunnel: string[] ["READ NAVX", "RESET FLAGS", "RESET ENCODERS", "", "", ""] -> [w2957] mode=indexing
                      n958 = Enqueue Element(queue=w2959, element=w2957) -> (queue out=w2958:refnum<queue>)  [unwired: 2 in, 2 out]
                    }
                  }
                }
                n959 = Select(t=State_Type_Definitions,_for_0.26g_versions_and_later_3."True Stop" ("Enum"), s=w2935, f=State_Type_Definitions,_for_0.26g_versions_and_later_3."Task 9I: ROTATE 90 CW" ("Enum")) -> (s? t:f=w2940:T18)
                n960 = Select(t=w2940, s=w2938, f=State_Type_Definitions,_for_0.26g_versions_and_later_3."Task 9H: SCAN BOX 2" ("Enum")) -> (s? t:f=w2946:T18)
              }
              frame "Exit" {
                n961 = for {
                  shift-right: [w2966] -> w2963
                  shift-left: w2962 -> [w2967]
                  tunnel: string[] ["STOP", "RESET ENCODERS", "RESET YAW", "ARDUINO MODE 0"] -> [w2965] mode=indexing
                  n962 = Enqueue Element(queue=w2967, element=w2965) -> (queue out=w2966:refnum<queue>)  [unwired: 2 in, 2 out]
                }
              }
            }
          }
          frame "Task 9I: ROTATE 90 CW" {
            # "High battery voltage: -36\nMid voltage: -38 \nLow voltage: -40"
            # ">> Item Selection Bias >>"
            n963 = Less Or Equal?(x=w2970, y=-38.0) -> (x <= y?=w2968:bool)
            n964 = Dequeue Element(queue=w2971, timeout in ms (-1)=w2972, error in (no error)=w2973) -> (element=w2979:T10)  [unwired: 3 out]
            n965 = case shown="\"Start Task 1\", Default" w2979 {
              tunnel: w2968 -> [w2985 _]
              tunnel: [w2992 State_Type_Definitions,_for_0.26g_versions_and_later_3."True Stop" ("Enum")] -> w2976
              tunnel: w2974 -> [w2984 _]
              tunnel: w2978 -> [w2991 w3008]
              tunnel: [w2990 w3009] -> w2977
              tunnel: [State_Type_Definitions,_for_0.26g_versions_and_later_3."Idle" ("Enum") State_Type_Definitions,_for_0.26g_versions_and_later_3."Shutdown" ("Enum")] -> w2975
              frame "Start Task 1", Default {
                n966 = case shown="False" w2985 {
                  tunnel: w2991 -> [w2995 w3002]
                  tunnel: [w2996 w3001] -> w2990
                  frame False {
                    n967 = for {
                      tunnel: string[] ["R-CW", "READ ENCODERS", "READ IR", "READ NAVX"] ("element") -> [w2997] mode=indexing
                      shift-right: [w2999] -> w2996
                      shift-left: w2995 -> [w2998]
                      n968 = Enqueue Element(queue=w2998, element=w2997) -> (queue out=w2999:refnum<queue>)  [unwired: 2 in, 2 out]
                    }
                  }
                  frame True {
                    n969 = for {
                      shift-right: [w3004] -> w3001
                      shift-left: w3002 -> [w3005]
                      tunnel: string[] ["STOP", "RESET ENCODERS", "RESET YAW", "RESET FLAGS", "READ IR", ""] -> [w3003] mode=indexing
                      n970 = Enqueue Element(queue=w3005, element=w3003) -> (queue out=w3004:refnum<queue>)  [unwired: 2 in, 2 out]
                    }
                  }
                }
                n971 = Or(x=w2985, y=w2984) -> (x .or. y?=w2983:bool)
                n972 = Select(t=State_Type_Definitions,_for_0.26g_versions_and_later_3."True Stop" ("Enum"), s=w2984, f=State_Type_Definitions,_for_0.26g_versions_and_later_3."Task 9J: FORWARD" ("Enum")) -> (s? t:f=w2986:T18)
                n973 = Select(t=w2986, s=w2983, f=State_Type_Definitions,_for_0.26g_versions_and_later_3."Task 9I: ROTATE 90 CW" ("Enum")) -> (s? t:f=w2992:T18)
              }
              frame "Exit" {
                n974 = for {
                  shift-right: [w3012] -> w3009
                  shift-left: w3008 -> [w3013]
                  tunnel: string[] ["STOP", "RESET ENCODERS", "RESET YAW", "ARDUINO MODE 0"] -> [w3011] mode=indexing
                  n975 = Enqueue Element(queue=w3013, element=w3011) -> (queue out=w3012:refnum<queue>)  [unwired: 2 in, 2 out]
                }
              }
            }
          }
          frame "Task 9J: FORWARD" {
            # "Tried values: 70, 150"
            # ">>Stops if either table or wall is obstructing >>"
            # ">> Item Selection Bias >>"
            n976 = Less?(x=w3016, y=150.0) -> (x < y?=w3019:bool)
            n977 = Greater Than 0?(x=w3016) -> (x > 0?=w3018:bool)
            n978 = Less Or Equal?(x=w3022, y=20.0) -> (x <= y?=w3020:bool)
            n979 = Greater Than 0?(x=w3022) -> (x > 0?=w3021:bool)
            n980 = And(x=w3018, y=w3019) -> ()  [unwired: 1 out]
            n981 = Dequeue Element(queue=w3028, timeout in ms (-1)=w3029, error in (no error)=w3030) -> (element=w3032:T10)  [unwired: 3 out]
            n982 = And(x=w3021, y=w3020) -> (x .and. y?=w3014:bool)
            n983 = Or(x=w3014, y=w3014) -> (x .or. y?=w3015:bool)
            n984 = case shown="\"Start Task 1\", Default" w3032 {
              tunnel: w3015 -> [w3038 _]
              tunnel: [w3045 State_Type_Definitions,_for_0.26g_versions_and_later_3."True Stop" ("Enum")] -> w3026
              tunnel: w3031 -> [w3037 _]
              tunnel: w3027 -> [w3044 w3061]
              tunnel: [w3043 w3062] -> w3025
              tunnel: [State_Type_Definitions,_for_0.26g_versions_and_later_3."Idle" ("Enum") State_Type_Definitions,_for_0.26g_versions_and_later_3."Shutdown" ("Enum")] -> w3024
              frame "Start Task 1", Default {
                n985 = case shown="True" w3038 {
                  tunnel: w3044 -> [w3048 w3055]
                  tunnel: [w3049 w3054] -> w3043
                  frame False {
                    n986 = for {
                      tunnel: string[] ["READ IR", "READ NAVX", "FORWARD"] ("element") -> [w3050] mode=indexing
                      shift-right: [w3052] -> w3049
                      shift-left: w3048 -> [w3051]
                      n987 = Enqueue Element(queue=w3051, element=w3050) -> (queue out=w3052:refnum<queue>)  [unwired: 2 in, 2 out]
                    }
                  }
                  frame True {
                    n988 = for {
                      shift-right: [w3057] -> w3054
                      shift-left: w3055 -> [w3058]
                      tunnel: string[] ["STOP", "RESET ENCODERS", "RESET YAW", "RESET FLAGS", "READ IR", ""] -> [w3056] mode=indexing
                      n989 = Enqueue Element(queue=w3058, element=w3056) -> (queue out=w3057:refnum<queue>)  [unwired: 2 in, 2 out]
                    }
                  }
                }
                n990 = Or(x=w3038, y=w3037) -> (x .or. y?=w3036:bool)
                n991 = Select(t=State_Type_Definitions,_for_0.26g_versions_and_later_3."True Stop" ("Enum"), s=w3037, f=State_Type_Definitions,_for_0.26g_versions_and_later_3."Task 9K: RAM WALL" ("Enum")) -> (s? t:f=w3039:T18)
                n992 = Select(t=w3039, s=w3036, f=State_Type_Definitions,_for_0.26g_versions_and_later_3."Task 9J: FORWARD" ("Enum")) -> (s? t:f=w3045:T18)
              }
              frame "Exit" {
                n993 = for {
                  shift-right: [w3065] -> w3062
                  shift-left: w3061 -> [w3066]
                  tunnel: string[] ["STOP", "RESET ENCODERS", "RESET YAW", "ARDUINO MODE 0"] -> [w3064] mode=indexing
                  n994 = Enqueue Element(queue=w3066, element=w3064) -> (queue out=w3065:refnum<queue>)  [unwired: 2 in, 2 out]
                }
              }
            }
          }
          frame "Task 9K: RAM WALL" {
            # "High battery voltage: 15"
            # ">> Item Selection Bias >>"
            # ">>Stops if either table or wall is obstructing >>"
            n995 = Less?(x=w3067, y=15.0) -> (x < y?=w3077:bool)
            n996 = Dequeue Element(queue=w3075, timeout in ms (-1)=w3074, error in (no error)=w3073) -> (element=w3079:T10)  [unwired: 3 out]
            n997 = case shown="\"Start Task 1\", Default" w3079 {
              tunnel: w3077 -> [w3084 _]
              tunnel: [w3091 State_Type_Definitions,_for_0.26g_versions_and_later_3."True Stop" ("Enum")] -> w3069
              tunnel: w3072 -> [w3083 _]
              tunnel: w3076 -> [w3090 w3107]
              tunnel: [w3089 w3108] -> w3070
              tunnel: [State_Type_Definitions,_for_0.26g_versions_and_later_3."Idle" ("Enum") State_Type_Definitions,_for_0.26g_versions_and_later_3."Shutdown" ("Enum")] -> w3068
              frame "Start Task 1", Default {
                n998 = case shown="True" w3084 {
                  tunnel: w3090 -> [w3094 w3101]
                  tunnel: [w3095 w3100] -> w3089
                  frame False {
                    n999 = for {
                      tunnel: string[] ["LEFT", "READ NAVX", "READ IR", ""] ("element") -> [w3096] mode=indexing
                      shift-right: [w3098] -> w3095
                      shift-left: w3094 -> [w3097]
                      n1000 = Enqueue Element(queue=w3097, element=w3096) -> (queue out=w3098:refnum<queue>)  [unwired: 2 in, 2 out]
                    }
                  }
                  frame True {
                    n1001 = for {
                      shift-right: [w3103] -> w3100
                      shift-left: w3101 -> [w3104]
                      tunnel: string[] ["STOP", "RESET ENCODERS", "RESET FLAGS", "RESET YAW", "READ IR", ""] -> [w3102] mode=indexing
                      n1002 = Enqueue Element(queue=w3104, element=w3102) -> (queue out=w3103:refnum<queue>)  [unwired: 2 in, 2 out]
                    }
                  }
                }
                n1003 = Or(x=w3084, y=w3083) -> (x .or. y?=w3082:bool)
                n1004 = Select(t=State_Type_Definitions,_for_0.26g_versions_and_later_3."True Stop" ("Enum"), s=w3083, f=State_Type_Definitions,_for_0.26g_versions_and_later_3."Task 9L: MOVE RIGHT" ("Enum")) -> (s? t:f=w3085:T18)
                n1005 = Select(t=w3085, s=w3082, f=State_Type_Definitions,_for_0.26g_versions_and_later_3."Task 9K: RAM WALL" ("Enum")) -> (s? t:f=w3091:T18)
              }
              frame "Exit" {
                n1006 = for {
                  shift-right: [w3111] -> w3108
                  shift-left: w3107 -> [w3112]
                  tunnel: string[] ["STOP", "RESET ENCODERS", "RESET YAW", "ARDUINO MODE 0"] -> [w3110] mode=indexing
                  n1007 = Enqueue Element(queue=w3112, element=w3110) -> (queue out=w3111:refnum<queue>)  [unwired: 2 in, 2 out]
                }
              }
            }
          }
          frame "Task 9L: MOVE RIGHT" {
            # "High battery voltage: 15"
            # ">>> Motor control cluster >>>"
            # ">>> yStepper command>>>"
            # ">> Item Selection Bias >>"
            n1008 = Dequeue Element(queue=w3120, timeout in ms (-1)=w3119, error in (no error)=w3118) -> (element=w3122:T10)  [unwired: 3 out]
            n1009 = case shown="\"Start Task 1\", Default" w3122 {
              tunnel: w3113 -> [w3128 _]
              tunnel: [w3135 State_Type_Definitions,_for_0.26g_versions_and_later_3."True Stop" ("Enum")] -> w3116
              tunnel: w3117 -> [w3127 _]
              tunnel: w3121 -> [w3134 w3151]
              tunnel: [w3133 w3152] -> w3114
              tunnel: [State_Type_Definitions,_for_0.26g_versions_and_later_3."Idle" ("Enum") State_Type_Definitions,_for_0.26g_versions_and_later_3."Shutdown" ("Enum")] -> w3115
              frame "Start Task 1", Default {
                n1010 = case shown="True" w3128 {
                  tunnel: w3134 -> [w3138 w3145]
                  tunnel: [w3139 w3144] -> w3133
                  frame False {
                    n1011 = for {
                      tunnel: string[] ["RIGHT", "READ NAVX", "READ LINE SENSOR", ""] ("element") -> [w3140] mode=indexing
                      shift-right: [w3142] -> w3139
                      shift-left: w3138 -> [w3141]
                      n1012 = Enqueue Element(queue=w3141, element=w3140) -> (queue out=w3142:refnum<queue>)  [unwired: 2 in, 2 out]
                    }
                  }
                  frame True {
                    n1013 = for {
                      shift-right: [w3147] -> w3144
                      shift-left: w3145 -> [w3148]
                      tunnel: string[] ["STOP", "RESET ENCODERS", "RESET FLAGS", "RESET YAW", "BOX COLOUR", ""] -> [w3146] mode=indexing
                      n1014 = Enqueue Element(queue=w3148, element=w3146) -> (queue out=w3147:refnum<queue>)  [unwired: 2 in, 2 out]
                    }
                  }
                }
                n1015 = Or(x=w3128, y=w3127) -> (x .or. y?=w3126:bool)
                n1016 = Select(t=State_Type_Definitions,_for_0.26g_versions_and_later_3."True Stop" ("Enum"), s=w3127, f=State_Type_Definitions,_for_0.26g_versions_and_later_3."Task 9M: SCAN BOX 3" ("Enum")) -> (s? t:f=w3129:T18)
                n1017 = Select(t=w3129, s=w3126, f=State_Type_Definitions,_for_0.26g_versions_and_later_3."Task 9L: MOVE RIGHT" ("Enum")) -> (s? t:f=w3135:T18)
              }
              frame "Exit" {
                n1018 = for {
                  shift-right: [w3155] -> w3152
                  shift-left: w3151 -> [w3156]
                  tunnel: string[] ["STOP", "RESET ENCODERS", "RESET YAW", "ARDUINO MODE 0"] -> [w3154] mode=indexing
                  n1019 = Enqueue Element(queue=w3156, element=w3154) -> (queue out=w3155:refnum<queue>)  [unwired: 2 in, 2 out]
                }
              }
            }
          }
          frame "Task 9M: SCAN BOX 3" {
            # ">>> Motor control cluster >>>"
            # ">>> yStepper command>>>"
            # ">> Item Selection Bias >>"
            n1020 = Dequeue Element(queue=w3166, timeout in ms (-1)=w3165, error in (no error)=w3164) -> (element=w3170:T10)  [unwired: 3 out]
            n1021 = call "Box Colour FGV.vi"("Init/R/W State"=Box_Colour_FGV_States."Read") -> ("Colour to detect (output)"=w3160:T2)  [unwired: 9 in, 1 out]
            n1022 = Equal?(x=w3159, y=w3160) -> (x = y?=w3158:bool)
            n1023 = case shown="\"Start Task 1\", Default" w3170 {
              tunnel: w3157 -> [w3178 _]
              tunnel: [w3185 State_Type_Definitions,_for_0.26g_versions_and_later_3."True Stop" ("Enum")] -> w3168
              tunnel: w3163 -> [w3174 _]
              tunnel: w3167 -> [w3184 w3201]
              tunnel: [w3183 w3202] -> w3162
              tunnel: [State_Type_Definitions,_for_0.26g_versions_and_later_3."Idle" ("Enum") State_Type_Definitions,_for_0.26g_versions_and_later_3."Shutdown" ("Enum")] -> w3169
              tunnel: w3158 -> [w3176 _]
              frame "Start Task 1", Default {
                n1024 = case shown="True" w3178 {
                  tunnel: w3184 -> [w3188 w3195]
                  tunnel: [w3189 w3194] -> w3183
                  frame False {
                    n1025 = for {
                      tunnel: string[] ["", "", "", ""] ("element") -> [w3190] mode=indexing
                      shift-right: [w3192] -> w3189
                      shift-left: w3188 -> [w3191]
                      n1026 = Enqueue Element(queue=w3191, element=w3190) -> (queue out=w3192:refnum<queue>)  [unwired: 2 in, 2 out]
                    }
                  }
                  frame True {
                    n1027 = for {
                      shift-right: [w3197] -> w3194
                      shift-left: w3195 -> [w3198]
                      tunnel: string[] ["STOP", "RESET ENCODERS", "RESET FLAGS", "RESET YAW", "", ""] -> [w3196] mode=indexing
                      n1028 = Enqueue Element(queue=w3198, element=w3196) -> (queue out=w3197:refnum<queue>)  [unwired: 2 in, 2 out]
                    }
                  }
                }
                n1029 = Or(x=w3178, y=w3174) -> (x .or. y?=w3177:bool)
                n1030 = Or(x=w3176, y=w3174) -> (x .or. y?=w3175:bool)
                n1031 = Select(t=State_Type_Definitions,_for_0.26g_versions_and_later_3."True Stop" ("Enum"), s=w3175, f=State_Type_Definitions,_for_0.26g_versions_and_later_3."Task 9N: MOVE RIGHT" ("Enum")) -> (s? t:f=w3179:T18)
                n1032 = Select(t=w3179, s=w3177, f=State_Type_Definitions,_for_0.26g_versions_and_later_3."Task 9M: SCAN BOX 3" ("Enum")) -> (s? t:f=w3185:T18)
              }
              frame "Exit" {
                n1033 = for {
                  shift-right: [w3205] -> w3202
                  shift-left: w3201 -> [w3206]
                  tunnel: string[] ["STOP", "RESET ENCODERS", "RESET YAW", "ARDUINO MODE 0"] -> [w3204] mode=indexing
                  n1034 = Enqueue Element(queue=w3206, element=w3204) -> (queue out=w3205:refnum<queue>)  [unwired: 2 in, 2 out]
                }
              }
            }
          }
          frame "Task 9N: MOVE RIGHT" {
            # ">> Item Selection Bias >>"
            n1035 = Dequeue Element(queue=w3211, timeout in ms (-1)=w3210, error in (no error)=w3209) -> (element=w3216:T10)  [unwired: 3 out]
            n1036 = case shown="\"Start Task 1\", Default" w3216 {
              tunnel: w3207 -> [w3222 _]
              tunnel: [w3229 State_Type_Definitions,_for_0.26g_versions_and_later_3."True Stop" ("Enum")] -> w3214
              tunnel: w3208 -> [w3221 _]
              tunnel: w3212 -> [w3228 w3245]
              tunnel: [w3227 w3246] -> w3213
              tunnel: [State_Type_Definitions,_for_0.26g_versions_and_later_3."Idle" ("Enum") State_Type_Definitions,_for_0.26g_versions_and_later_3."Shutdown" ("Enum")] -> w3215
              frame "Start Task 1", Default {
                n1037 = case shown="True" w3222 {
                  tunnel: w3228 -> [w3232 w3239]
                  tunnel: [w3233 w3238] -> w3227
                  frame False {
                    n1038 = for {
                      tunnel: string[] ["READ LINE SENSOR", "READ NAVX", "RIGHT", "READ ENCODERS"] ("element") -> [w3234] mode=indexing
                      shift-right: [w3236] -> w3233
                      shift-left: w3232 -> [w3235]
                      n1039 = Enqueue Element(queue=w3235, element=w3234) -> (queue out=w3236:refnum<queue>)  [unwired: 2 in, 2 out]
                    }
                  }
                  frame True {
                    n1040 = for {
                      shift-right: [w3241] -> w3238
                      shift-left: w3239 -> [w3242]
                      tunnel: string[] ["STOP", "RESET ENCODERS", "RESET YAW", "RESET FLAGS", "BOX COLOUR", ""] -> [w3240] mode=indexing
                      n1041 = Enqueue Element(queue=w3242, element=w3240) -> (queue out=w3241:refnum<queue>)  [unwired: 2 in, 2 out]
                    }
                  }
                }
                n1042 = Or(x=w3222, y=w3221) -> (x .or. y?=w3220:bool)
                n1043 = Select(t=State_Type_Definitions,_for_0.26g_versions_and_later_3."True Stop" ("Enum"), s=w3221, f=State_Type_Definitions,_for_0.26g_versions_and_later_3."Task 9O: SCAN BOX 4" ("Enum")) -> (s? t:f=w3223:T18)
                n1044 = Select(t=w3223, s=w3220, f=State_Type_Definitions,_for_0.26g_versions_and_later_3."Task 9N: MOVE RIGHT" ("Enum")) -> (s? t:f=w3229:T18)
              }
              frame "Exit" {
                n1045 = for {
                  shift-right: [w3249] -> w3246
                  shift-left: w3245 -> [w3250]
                  tunnel: string[] ["STOP", "RESET ENCODERS", "RESET YAW", "ARDUINO MODE 0"] -> [w3248] mode=indexing
                  n1046 = Enqueue Element(queue=w3250, element=w3248) -> (queue out=w3249:refnum<queue>)  [unwired: 2 in, 2 out]
                }
              }
            }
          }
          frame "Task 9O: SCAN BOX 4" {
            # ">>> Motor control cluster >>>"
            # ">>> yStepper command>>>"
            # ">> Item Selection Bias >>"
            n1047 = Dequeue Element(queue=w3261, timeout in ms (-1)=w3260, error in (no error)=w3259) -> (element=w3265:T10)  [unwired: 3 out]
            n1048 = call "Box Colour FGV.vi"("Init/R/W State"=Box_Colour_FGV_States."Read") -> ("Colour to detect (output)"=w3263:T2)  [unwired: 9 in, 1 out]
            n1049 = Equal?(x=w3253, y=w3263) -> (x = y?=w3262:bool)
            n1050 = case shown="\"Start Task 1\", Default" w3265 {
              tunnel: w3251 -> [w3272 _]
              tunnel: [w3279 State_Type_Definitions,_for_0.26g_versions_and_later_3."True Stop" ("Enum")] -> w3255
              tunnel: w3258 -> [w3268 _]
              tunnel: w3252 -> [w3278 w3295]
              tunnel: [w3277 w3296] -> w3256
              tunnel: [State_Type_Definitions,_for_0.26g_versions_and_later_3."Idle" ("Enum") State_Type_Definitions,_for_0.26g_versions_and_later_3."Shutdown" ("Enum")] -> w3254
              tunnel: w3262 -> [w3270 _]
              frame "Start Task 1", Default {
                n1051 = case shown="True" w3272 {
                  tunnel: w3278 -> [w3282 w3289]
                  tunnel: [w3283 w3288] -> w3277
                  frame False {
                    n1052 = for {
                      tunnel: string[] ["", "", "", ""] ("element") -> [w3284] mode=indexing
                      shift-right: [w3286] -> w3283
                      shift-left: w3282 -> [w3285]
                      n1053 = Enqueue Element(queue=w3285, element=w3284) -> (queue out=w3286:refnum<queue>)  [unwired: 2 in, 2 out]
                    }
                  }
                  frame True {
                    n1054 = for {
                      shift-right: [w3291] -> w3288
                      shift-left: w3289 -> [w3292]
                      tunnel: string[] ["STOP", "RESET ENCODERS", "RESET FLAGS", "RESET YAW", "", ""] -> [w3290] mode=indexing
                      n1055 = Enqueue Element(queue=w3292, element=w3290) -> (queue out=w3291:refnum<queue>)  [unwired: 2 in, 2 out]
                    }
                  }
                }
                n1056 = Or(x=w3272, y=w3268) -> (x .or. y?=w3271:bool)
                n1057 = Or(x=w3270, y=w3268) -> (x .or. y?=w3269:bool)
                n1058 = Select(t=State_Type_Definitions,_for_0.26g_versions_and_later_3."True Stop" ("Enum"), s=w3269, f=State_Type_Definitions,_for_0.26g_versions_and_later_3."True Stop" ("Enum")) -> (s? t:f=w3273:T18)
                n1059 = Select(t=w3273, s=w3271, f=State_Type_Definitions,_for_0.26g_versions_and_later_3."Task 9O: SCAN BOX 4" ("Enum")) -> (s? t:f=w3279:T18)
              }
              frame "Exit" {
                n1060 = for {
                  shift-right: [w3299] -> w3296
                  shift-left: w3295 -> [w3300]
                  tunnel: string[] ["STOP", "RESET ENCODERS", "RESET YAW", "ARDUINO MODE 0"] -> [w3298] mode=indexing
                  n1061 = Enqueue Element(queue=w3300, element=w3298) -> (queue out=w3299:refnum<queue>)  [unwired: 2 in, 2 out]
                }
              }
            }
          }
        }
        "Object Detection" <- w324
        "Ultrasonic sensors" <- w347
        "Encoder values" <- w336
        "Stepper position values" <- w320
        "NAVX Values" <- w318
        "IR Sensors" <- w310
        "Line sensors" <- w305
        "Time cluster" <- w316
        "Box Colour Detection" <- w298
      }
    }
    "Object recognition mode" <- w222
    "Front Ultrasonic obstruct" <- w219
    "Front IR obstruct" <- w218
    "Table IR obstruct" <- w217
    "Same colour?" <- w212
    n1062 = local write "Green LED"(w232) -> ()
  }
  n1063 = while {
    tunnel: w47 -> [w4219]
    tunnel: w46 -> [w4216]
    stop <- w4213 stop-if-true
    # "Status Loop for Action Queues"
    n1064 = Get Queue Status(queue=w4219, return elements? (F)=TRUE) -> (error out=w4215:errorcluster, # elements in queue=→"Action Queue Items":i32, elements=→"Action Queues items":string[])  [unwired: 1 in, 5 out]
    n1065 = Get Queue Status(queue=w4216, return elements? (F)=TRUE) -> (# pending remove=→"State Logic Queue Items":i32, error out=w4214:errorcluster, elements=→"elements":T10[])  [unwired: 1 in, 5 out]
    n1066 = Merge Errors(w4215, w4214) -> (w4213:errorcluster)
    n1067 = Wait (ms)(milliseconds to wait=u32 500) -> ()  [unwired: 1 out]
  }
  n1068 = while {
    stop <- w4223 stop-if-true
    n1069 = call "MOTOR CONTROL WITH PID AE.vi"("AE Mode"=MOTOR_CONTROL_WITH_PID_AE_DATA_MODE_TYPE_DEF."Read from AE") -> ("Speed & distance"=→"Speed & distance":T15)  [unwired: 3 in]
    n1070 = call "FGV Bool.vi"("Init/Read/Write State"=States_for_Action_Engine."Read") -> ("Output node"=w4223:bool)  [unwired: 2 in, 1 out]
    n1071 = Wait (ms)(milliseconds to wait=u32 5) -> ()  [unwired: 1 out]
  }
  n1072 = call <vilib>:"DIO Close.vi"("error in (no error)"=w23, "DIO Info In"=w26) -> ()  [unwired: 9 in, 1 out]
  n1073 = call <vilib>:"DIO Close.vi"("error in (no error)"=w33, "DIO Info In"=w35) -> ()  [unwired: 9 in, 1 out]
  n1074 = call <vilib>:"NavX Close.vi"("error in (no error)"=w10, "NavX Info In"=w9) -> ()  [unwired: 9 in, 1 out]
  n1075 = call <vilib>:"DIO Close.vi"("error in (no error)"=w28, "DIO Info In"=w30) -> ()  [unwired: 9 in, 1 out]
  n1076 = call <vilib>:"DIO Close.vi"("error in (no error)"=w17, "DIO Info In"=w18) -> ()  [unwired: 9 in, 1 out]
  n1077 = call <vilib>:"DIO Close.vi"("error in (no error)"=w12, "DIO Info In"=w13) -> ()  [unwired: 9 in, 1 out]
  n1078 = Merge Errors "Merge Errors"(w63, w62) -> (w45:errorcluster)
  n1079 = Merge Errors(w49, w45) -> (w44:errorcluster)
  n1080 = Destroy User Event(user event=w67, error in=w44) -> ()  [unwired: 1 out]
  n1081 = Release Queue(queue=w40, error in (no error)=w44) -> (error out=→"Queue Errors":errorcluster)  [unwired: 1 in, 2 out]
  n1082 = Release Queue(queue=w57, error in (no error)=w44) -> ()  [unwired: 1 in, 3 out]
  n1083 = Destroy User Event(user event=w66, error in=w44) -> ()  [unwired: 1 out]
  n1084 = Unregister For Events(event registration refnum=w58, error in=w44) -> ()  [unwired: 1 out]
